vi "Results_file_Plotter.vi"() -> ()   [LabVIEW 2013]
uses:
  Anemometry/Anemometry Sub Vis/Data_plotting_vis/Plot_Slice.ctl
  Anemometry/Anemometry Sub Vis/Data_plotting_vis/Plotter_Mode.ctl
  Anemometry/Anemometry Sub Vis/Data_plotting_vis/Data_File_Type.ctl
  Anemometry/Anemometry Sub Vis/File/Setup_Filetype.ctl
  Anemometry/Anemometry Sub Vis/Controls/Global_mode.ctl
  Anemometry/Anemometry Sub Vis/Data_plotting_vis/Results_plotter_Global.vi
  Anemometry/Anemometry Sub Vis/Globals/Trav_pos_global.vi
  Instance           1 28Saved   Results_file_Plotter .vi
  Anemometry/Anemometry Sub Vis/Globals/Constants_global.vi
panel:
  out "Edit Raw DF?":bool
  in  "Tab Control":T1(tab)=enum."Save "
  in  "Template":path
  in  "Empty":bool
  in  "Result files to read":path[](array[path])
  in  "Add results file":bool
  in  "File Types to Read":T2
  in  "Dot Plot?":bool
  in  "Vector Plot?":bool
  in  "Ordinate Name":string
  out "2nd Add label":string
  out "First Add label":string
  in  "Additional X Values":dbl[](array[numeric]) format="%.2f"
  in  "Additional Y Values":dbl[](array[numeric]) format="%.2f"
  in  "Show Results Space Analysis":bool
  in  "Show Plot Space Analysis":bool
  in  "Multi Ordinate":i32[](listbox)
  in  "Multi Ordinate?":bool
  in  "Ordinate":u16(ring) items=["Project", "Case2", "Case", "Date", "File", "Ref Velocity (m/s) X=5m Y=-0.780m Z=1m", "Source Location X (mm)", "Source Location Y (mm)", "Source Location Z (mm)", "Source Internal Diameter (mm)", "Model Orientation", "Carrier Gas", "Trace Gas", "Q Source (l/min)", "Q Trace (l/min)", "Source Density Ratio", "Source", "X (mm)", "Y (mm)", "Z (mm)", "Location XY", "Location XZ", "Profiles", "U/U(ref)", "V/U(ref)", "W/U(ref)", "u^2/U_{ref}^2", "v^2/U_{ref}^2", "w^2/U_{ref}^2", "uv/U_{ref}^2", "-uw/U_{ref}^2", "CU(ref)/Q (m^{-2})", "c'U(ref)/Q (m^{-2})", "uc/Q (m^{-2})", "vc/Q (m^{-2})", "wc/Q (m^{-2})", "Measurement Time (min)", "U (m/s)", "U (m/s) St Error", "V (m/s)", "W (m/s)", "u^2 (m/s)^2", "v^2 (m/s)^2", "w^2 (m/s)^2", "uv (m/s)^2", "uw (m/s)^2", "C Trace (ppm)", "C Trace (ppm) St Error", "c^2 (ppm)^2", "uc (ppm m/s)", "vc (ppm m/s)", "wc (ppm m/s)", "Raw Data Filename", "EnFlo_Tunnel Inlet_Temp St Deviation", "Instrumentation", "Number of FFID Samples per Block", "Total Number of FFID Spikes Removed", "LDA (U) Timescale Estimate Integrated to 25%", "Number Of Measurement Blocks", "LDA Sampling Rate (Hz)", "Number of LDA Samples per Block", "Multi Run Start Time", "Bkgnd FF (C)", "Bkgnd Variance FF (C)", "Seconds since 1st Jan", "Drift%", "CU/Q Err", "EnFlo Lab labstrat1 Delta T", "GMU Carrier 2 Gas", "Emission Velocity m/s", "Emission Ratio", "FF (C) Standard Error in Variance", "GMU Source Type", "Aero_Tunnel Speed Meas Velocity", "Multi Run Row Number", "LDA (W) Standard Error in Mean", "LDA (U) Standard Error in Variance", "EnFlo_Tunnel FFID Temp", "FF (C) Calibration Filename", "Source2 Enable", "GMU Source Dem Q", "Multi Run Command Filename", "Thermistor Temp", "University Outside Temp", "Spires", "Run", "EnFlo_Tunnel Usonic_Ref_2 Velocity", "Roughness", "Dem_Uref", "Comments", "X Tunnel (mm)", "EnFlo_Tunnel Trav Origin X Offset", "Run_", "EnFlo_Tunnel Metadata Source Number", "EnFlo_Tunnel Metadata Model Trees"]
  in  "Intensity Plot?":bool
  in  "Absisca":u16(ring) items=["Project", "Case2", "Case", "Date", "File", "Ref Velocity (m/s) X=5m Y=-0.780m Z=1m", "Source Location X (mm)", "Source Location Y (mm)", "Source Location Z (mm)", "Source Internal Diameter (mm)", "Model Orientation", "Carrier Gas", "Trace Gas", "Q Source (l/min)", "Q Trace (l/min)", "Source Density Ratio", "Source", "X (mm)", "Y (mm)", "Z (mm)", "Location XY", "Location XZ", "Profiles", "U/U(ref)", "V/U(ref)", "W/U(ref)", "u^2/U_{ref}^2", "v^2/U_{ref}^2", "w^2/U_{ref}^2", "uv/U_{ref}^2", "-uw/U_{ref}^2", "CU(ref)/Q (m^{-2})", "c'U(ref)/Q (m^{-2})", "uc/Q (m^{-2})", "vc/Q (m^{-2})", "wc/Q (m^{-2})", "Measurement Time (min)", "U (m/s)", "U (m/s) St Error", "V (m/s)", "W (m/s)", "u^2 (m/s)^2", "v^2 (m/s)^2", "w^2 (m/s)^2", "uv (m/s)^2", "uw (m/s)^2", "C Trace (ppm)", "C Trace (ppm) St Error", "c^2 (ppm)^2", "uc (ppm m/s)", "vc (ppm m/s)", "wc (ppm m/s)", "Raw Data Filename", "EnFlo_Tunnel Inlet_Temp St Deviation", "Instrumentation", "Number of FFID Samples per Block", "Total Number of FFID Spikes Removed", "LDA (U) Timescale Estimate Integrated to 25%", "Number Of Measurement Blocks", "LDA Sampling Rate (Hz)", "Number of LDA Samples per Block", "Multi Run Start Time", "Bkgnd FF (C)", "Bkgnd Variance FF (C)", "Seconds since 1st Jan", "Drift%", "CU/Q Err", "EnFlo Lab labstrat1 Delta T", "GMU Carrier 2 Gas", "Emission Velocity m/s", "Emission Ratio", "FF (C) Standard Error in Variance", "GMU Source Type", "Aero_Tunnel Speed Meas Velocity", "Multi Run Row Number", "LDA (W) Standard Error in Mean", "LDA (U) Standard Error in Variance", "EnFlo_Tunnel FFID Temp", "FF (C) Calibration Filename", "Source2 Enable", "GMU Source Dem Q", "Multi Run Command Filename", "Thermistor Temp", "University Outside Temp", "Spires", "Run", "EnFlo_Tunnel Usonic_Ref_2 Velocity", "Roughness", "Dem_Uref", "Comments", "X Tunnel (mm)", "EnFlo_Tunnel Trav Origin X Offset", "Run_", "EnFlo_Tunnel Metadata Source Number", "EnFlo_Tunnel Metadata Model Trees"]
  in  "Job Directory":path
  in  "Save Averaged rows":bool
  in  "Save Surface Fit":bool
  in  "Output Filename":path
  in  "Save Data in Rows":bool
  in  "Save Plot data":bool
  in  "Header":string
  in  "Process Point":bool
  in  "Kill Point":bool
  out "Table":string[][](table)
  in  "Post Process Plotted Data":bool
  in  "...using routine":string
  in  "Calculate new metadata":bool
  in  "Add /Edit metadata":bool
  in  "Delete Plotted data from file":bool
  in  "Save Setup":bool
  in  "Load Setup":bool
  in  "stop":bool
  out "Current":string="Graph Scales"
  in  "Single Series":i32[](listbox)=[0]
  in  "Edit Template File":bool
  in  "color and symbol":bool
  out "nRows":i32
  in  "Filter Bins 2":i32[](listbox)=[0]
  in  "Filter 6":u16(ring)
  in  "Filter 5":u16(ring)
  in  "Filter 4":u16(ring)
  in  "Filter 3":u16(ring) items=["Show All (55)", "Lateral Profile (25)", "Vertical Profile (30)", "NOT Lateral Profile (30)", "NOT Vertical Profile (25)"]
  in  "Filter Array":u16[](array[ring])=[0, 0, 0, 0, 0, 0] items=["Don't Filter", "Project", "Case2", "Case", "Date", "File", "Ref Velocity (m/s) X=5m Y=-0.780m Z=1m", "Source Location X (mm)", "Source Location Y (mm)", "Source Location Z (mm)", "Source Internal Diameter (mm)", "Model Orientation", "Carrier Gas", "Trace Gas", "Q Source (l/min)", "Q Trace (l/min)", "Source Density Ratio", "Source", "X (mm)", "Y (mm)", "Z (mm)", "Location XY", "Location XZ", "Profiles", "U/U(ref)", "V/U(ref)", "W/U(ref)", "u^2/U_{ref}^2", "v^2/U_{ref}^2", "w^2/U_{ref}^2", "uv/U_{ref}^2", "-uw/U_{ref}^2", "CU(ref)/Q (m^{-2})", "c'U(ref)/Q (m^{-2})", "uc/Q (m^{-2})", "vc/Q (m^{-2})", "wc/Q (m^{-2})", "Measurement Time (min)", "U (m/s)", "U (m/s) St Error", "V (m/s)", "W (m/s)", "u^2 (m/s)^2", "v^2 (m/s)^2", "w^2 (m/s)^2", "uv (m/s)^2", "uw (m/s)^2", "C Trace (ppm)", "C Trace (ppm) St Error", "c^2 (ppm)^2", "uc (ppm m/s)", "vc (ppm m/s)", "wc (ppm m/s)", "Raw Data Filename", "EnFlo_Tunnel Inlet_Temp St Deviation", "Instrumentation", "Number of FFID Samples per Block", "Total Number of FFID Spikes Removed", "LDA (U) Timescale Estimate Integrated to 25%", "Number Of Measurement Blocks", "LDA Sampling Rate (Hz)", "Number of LDA Samples per Block", "Multi Run Start Time", "Bkgnd FF (C)", "Bkgnd Variance FF (C)", "Seconds since 1st Jan", "Drift%", "CU/Q Err", "EnFlo Lab labstrat1 Delta T", "GMU Carrier 2 Gas", "Emission Velocity m/s", "Emission Ratio", "FF (C) Standard Error in Variance", "GMU Source Type", "Aero_Tunnel Speed Meas Velocity", "Multi Run Row Number", "LDA (W) Standard Error in Mean", "LDA (U) Standard Error in Variance", "EnFlo_Tunnel FFID Temp", "FF (C) Calibration Filename", "Source2 Enable", "GMU Source Dem Q", "Multi Run Command Filename", "Thermistor Temp", "University Outside Temp", "Spires", "Run", "EnFlo_Tunnel Usonic_Ref_2 Velocity", "Roughness", "Dem_Uref", "Comments", "X Tunnel (mm)", "EnFlo_Tunnel Trav Origin X Offset", "Run_", "EnFlo_Tunnel Metadata Source Number", "EnFlo_Tunnel Metadata Model Trees"]
  in  "Filter Bins 1":i32[](listbox)=[0]
  in  "Create picture Vi Name":string caption="Picture VI:"
  in  "Save Plot as jpg":bool
  in  "Reload Files":bool
  out "Selected Row":i32
  out "Selected Row?":bool
  out "Warning!":string
  out "XY Plot":cluster{dbl[], dbl[]}[](graph)
  out "Edit Raw Data Header Info":bool
  out "Raw DF in Orig Pos?":bool
  out "Intensity Graph":dbl[][](graph)
  in  "Bkgnd Value":dbl
  in  "Update":bool
  in  "Plot Resolution":bool
  in  "Point Size":i32(slide)=1 scale=0.0..10.0
  in  "No of Contours":i32=20
  in  "Slice mode":T3
  in  "Z Ch Name":u16(ring) items=["Project", "Case2", "Case", "Date", "File", "Ref Velocity (m/s) X=5m Y=-0.780m Z=1m", "Source Location X (mm)", "Source Location Y (mm)", "Source Location Z (mm)", "Source Internal Diameter (mm)", "Model Orientation", "Carrier Gas", "Trace Gas", "Q Source (l/min)", "Q Trace (l/min)", "Source Density Ratio", "Source", "X (mm)", "Y (mm)", "Z (mm)", "Location XY", "Location XZ", "Profiles", "U/U(ref)", "V/U(ref)", "W/U(ref)", "u^2/U_{ref}^2", "v^2/U_{ref}^2", "w^2/U_{ref}^2", "uv/U_{ref}^2", "-uw/U_{ref}^2", "CU(ref)/Q (m^{-2})", "c'U(ref)/Q (m^{-2})", "uc/Q (m^{-2})", "vc/Q (m^{-2})", "wc/Q (m^{-2})", "Measurement Time (min)", "U (m/s)", "U (m/s) St Error", "V (m/s)", "W (m/s)", "u^2 (m/s)^2", "v^2 (m/s)^2", "w^2 (m/s)^2", "uv (m/s)^2", "uw (m/s)^2", "C Trace (ppm)", "C Trace (ppm) St Error", "c^2 (ppm)^2", "uc (ppm m/s)", "vc (ppm m/s)", "wc (ppm m/s)", "Raw Data Filename", "EnFlo_Tunnel Inlet_Temp St Deviation", "Instrumentation", "Number of FFID Samples per Block", "Total Number of FFID Spikes Removed", "LDA (U) Timescale Estimate Integrated to 25%", "Number Of Measurement Blocks", "LDA Sampling Rate (Hz)", "Number of LDA Samples per Block", "Multi Run Start Time", "Bkgnd FF (C)", "Bkgnd Variance FF (C)", "Seconds since 1st Jan", "Drift%", "CU/Q Err", "EnFlo Lab labstrat1 Delta T", "GMU Carrier 2 Gas", "Emission Velocity m/s", "Emission Ratio", "FF (C) Standard Error in Variance", "GMU Source Type", "Aero_Tunnel Speed Meas Velocity", "Multi Run Row Number", "LDA (W) Standard Error in Mean", "LDA (U) Standard Error in Variance", "EnFlo_Tunnel FFID Temp", "FF (C) Calibration Filename", "Source2 Enable", "GMU Source Dem Q", "Multi Run Command Filename", "Thermistor Temp", "University Outside Temp", "Spires", "Run", "EnFlo_Tunnel Usonic_Ref_2 Velocity", "Roughness", "Dem_Uref", "Comments", "X Tunnel (mm)", "EnFlo_Tunnel Trav Origin X Offset", "Run_", "EnFlo_Tunnel Metadata Source Number", "EnFlo_Tunnel Metadata Model Trees"]
  in  "Y Ch Name":u16(ring) items=["Project", "Case2", "Case", "Date", "File", "Ref Velocity (m/s) X=5m Y=-0.780m Z=1m", "Source Location X (mm)", "Source Location Y (mm)", "Source Location Z (mm)", "Source Internal Diameter (mm)", "Model Orientation", "Carrier Gas", "Trace Gas", "Q Source (l/min)", "Q Trace (l/min)", "Source Density Ratio", "Source", "X (mm)", "Y (mm)", "Z (mm)", "Location XY", "Location XZ", "Profiles", "U/U(ref)", "V/U(ref)", "W/U(ref)", "u^2/U_{ref}^2", "v^2/U_{ref}^2", "w^2/U_{ref}^2", "uv/U_{ref}^2", "-uw/U_{ref}^2", "CU(ref)/Q (m^{-2})", "c'U(ref)/Q (m^{-2})", "uc/Q (m^{-2})", "vc/Q (m^{-2})", "wc/Q (m^{-2})", "Measurement Time (min)", "U (m/s)", "U (m/s) St Error", "V (m/s)", "W (m/s)", "u^2 (m/s)^2", "v^2 (m/s)^2", "w^2 (m/s)^2", "uv (m/s)^2", "uw (m/s)^2", "C Trace (ppm)", "C Trace (ppm) St Error", "c^2 (ppm)^2", "uc (ppm m/s)", "vc (ppm m/s)", "wc (ppm m/s)", "Raw Data Filename", "EnFlo_Tunnel Inlet_Temp St Deviation", "Instrumentation", "Number of FFID Samples per Block", "Total Number of FFID Spikes Removed", "LDA (U) Timescale Estimate Integrated to 25%", "Number Of Measurement Blocks", "LDA Sampling Rate (Hz)", "Number of LDA Samples per Block", "Multi Run Start Time", "Bkgnd FF (C)", "Bkgnd Variance FF (C)", "Seconds since 1st Jan", "Drift%", "CU/Q Err", "EnFlo Lab labstrat1 Delta T", "GMU Carrier 2 Gas", "Emission Velocity m/s", "Emission Ratio", "FF (C) Standard Error in Variance", "GMU Source Type", "Aero_Tunnel Speed Meas Velocity", "Multi Run Row Number", "LDA (W) Standard Error in Mean", "LDA (U) Standard Error in Variance", "EnFlo_Tunnel FFID Temp", "FF (C) Calibration Filename", "Source2 Enable", "GMU Source Dem Q", "Multi Run Command Filename", "Thermistor Temp", "University Outside Temp", "Spires", "Run", "EnFlo_Tunnel Usonic_Ref_2 Velocity", "Roughness", "Dem_Uref", "Comments", "X Tunnel (mm)", "EnFlo_Tunnel Trav Origin X Offset", "Run_", "EnFlo_Tunnel Metadata Source Number", "EnFlo_Tunnel Metadata Model Trees"]
  in  "X Ch Name":u16(ring) items=["Project", "Case2", "Case", "Date", "File", "Ref Velocity (m/s) X=5m Y=-0.780m Z=1m", "Source Location X (mm)", "Source Location Y (mm)", "Source Location Z (mm)", "Source Internal Diameter (mm)", "Model Orientation", "Carrier Gas", "Trace Gas", "Q Source (l/min)", "Q Trace (l/min)", "Source Density Ratio", "Source", "X (mm)", "Y (mm)", "Z (mm)", "Location XY", "Location XZ", "Profiles", "U/U(ref)", "V/U(ref)", "W/U(ref)", "u^2/U_{ref}^2", "v^2/U_{ref}^2", "w^2/U_{ref}^2", "uv/U_{ref}^2", "-uw/U_{ref}^2", "CU(ref)/Q (m^{-2})", "c'U(ref)/Q (m^{-2})", "uc/Q (m^{-2})", "vc/Q (m^{-2})", "wc/Q (m^{-2})", "Measurement Time (min)", "U (m/s)", "U (m/s) St Error", "V (m/s)", "W (m/s)", "u^2 (m/s)^2", "v^2 (m/s)^2", "w^2 (m/s)^2", "uv (m/s)^2", "uw (m/s)^2", "C Trace (ppm)", "C Trace (ppm) St Error", "c^2 (ppm)^2", "uc (ppm m/s)", "vc (ppm m/s)", "wc (ppm m/s)", "Raw Data Filename", "EnFlo_Tunnel Inlet_Temp St Deviation", "Instrumentation", "Number of FFID Samples per Block", "Total Number of FFID Spikes Removed", "LDA (U) Timescale Estimate Integrated to 25%", "Number Of Measurement Blocks", "LDA Sampling Rate (Hz)", "Number of LDA Samples per Block", "Multi Run Start Time", "Bkgnd FF (C)", "Bkgnd Variance FF (C)", "Seconds since 1st Jan", "Drift%", "CU/Q Err", "EnFlo Lab labstrat1 Delta T", "GMU Carrier 2 Gas", "Emission Velocity m/s", "Emission Ratio", "FF (C) Standard Error in Variance", "GMU Source Type", "Aero_Tunnel Speed Meas Velocity", "Multi Run Row Number", "LDA (W) Standard Error in Mean", "LDA (U) Standard Error in Variance", "EnFlo_Tunnel FFID Temp", "FF (C) Calibration Filename", "Source2 Enable", "GMU Source Dem Q", "Multi Run Command Filename", "Thermistor Temp", "University Outside Temp", "Spires", "Run", "EnFlo_Tunnel Usonic_Ref_2 Velocity", "Roughness", "Dem_Uref", "Comments", "X Tunnel (mm)", "EnFlo_Tunnel Trav Origin X Offset", "Run_", "EnFlo_Tunnel Metadata Source Number", "EnFlo_Tunnel Metadata Model Trees"]
  in  "Resolution":dbl=1.0 min=0.0 format="%.4f"
  out "Surface Area":dbl format="%^_6g"
  out "Surface Integral":dbl format="%^_6g"
  out "Surface Average":dbl format="%^#.6g"
  out "Uadvec":dbl
  in  "Full_Res_Results_Folder":path
  out "Last used Template":path
  out "Cursor index":i32
  out "Choosen Path":path
  in  "VI Refnum Calculation":refnum<vi>
  out "Filetype":string[](array[string])
  out "Mode":T4
  out "Plotted rows only?":bool
  in  "type specifier VI Refnum (for type only) 2":refnum<vi>
  in  "type specifier VI Refnum (for type only)":refnum<vi>
  out "Accept Array":bool[][](array[boolean])
  out "Previous slice mode":T3
  out "Slice mode Change?":bool
  out "Non-Blank Rows":bool[](array[boolean])
  out "File Index":i32
  out "Tolerances":dbl[](array[numeric]) format="%.2f"
  in  "Results files choosen":path[](array[path])
  in  "Transpose":bool
  out "Plotted Series":bool[][](array[boolean])
  in  "Results file":path
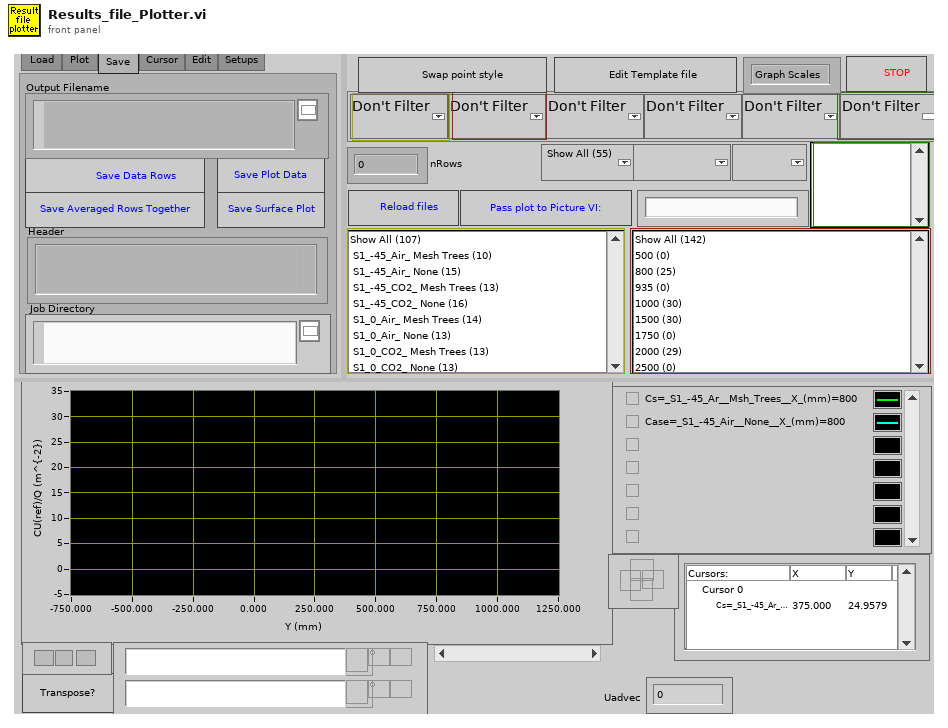
[diagram p1: front panel]
types:
  T1 = enum32{"Load ", "Plot ", "Save ", "Cursor", "Edit", "Setups"}
  T2 = typedef "Data_File_Type.ctl" = enum16{"Read All File Types", "Results Files Only", "Raw Data Files Only", "Calibration Files Only", "Gas Desk Files Only", "Old Results Files Only", "Tabulated Data Files Only"}
  T3 = typedef "Plot_Slice.ctl" = enum16{"XY Slice (Plan)", "YX Slice (Plan)", "YZ Slice (Cross)", "ZY Slice (Cross)", "XZ Slice (Side)", "ZX Slice (Side)"}
  T4 = typedef "Plotter_Mode.ctl" = enum16{"Save file", "Delete unwanted rows", "Edit Values with constants", "Edit values per row", "Edit Raw Data file header", "Post Process Plotted Rows"}
  T5 = typedef "Setup_Filetype.ctl" = enum16{"Measurement Setups", "Calibration Setups", "General", "Results File Plotter Setups", "Speed Calib Tweaks"}
  T6 = enum16{"Zero or one", "One", "Zero or more", "One or more"}
  T7 = typedef "Global_mode.ctl" = enum16{"Read Global", "Load Global From File", "Write Global to File"}
  T8 = enum16{"Edit Existing Template File", "Create New Template File"}
  T9 = enum16{"Show only data summary", "Show data summary", "No data summary"}
  T10 = typedef "All_Setup.ctl" = cluster{"Result files to read":path[], "Template":path, "Transpose":bool, "Additional X Values":dbl[], "Additional Y Values":dbl[], "Ordinate":u16, "Absisca":u16, "Filter Array":u16[], "color and symbol":bool, "Output Filename":path, "Jpg Vi Name":string, "Intensity Plot?":bool, "Multi Ordinate?":bool, "Filter Bins 1":i32[], "Filter Bins 2":i32[], "Multi Ordinate":i32[]}
  T11 = enum16{"Left Button", "Center Button", "Right Button", "Window Close"}
  T12 = enum32{"existing file", "new file", "new or existing file", "existing dir", "new dir", "new or existing dir", "existing file (use LLBs)", "new file (use LLBs)", "new or existing file (use LLBs)", "new or existing file or directory (use LLBs)"}
  T13 = cluster{"Plot Color":u32, "Plot Interpolation":u8, "Point Style":u8, "Line Style":u8, "Fill/Pt. Color":u32, "Line Width":u8, "Bar Plot Style":u8, "Fill To":i16}[]
  T14 = cluster{"X Max":dbl, "Y Max ":dbl, "X Scale":cluster{"Xo":dbl, "delta X":dbl}, "Y Scale":cluster{"Xo":dbl, "delta X":dbl}, "X Values":dbl[], "Y Values":dbl[], "Z Max":dbl, "Z Min":dbl}
  T15 = typedef "Group_Binning.ctl" = cluster{"Index":i32, "Tolerance":dbl, "Precision":string}
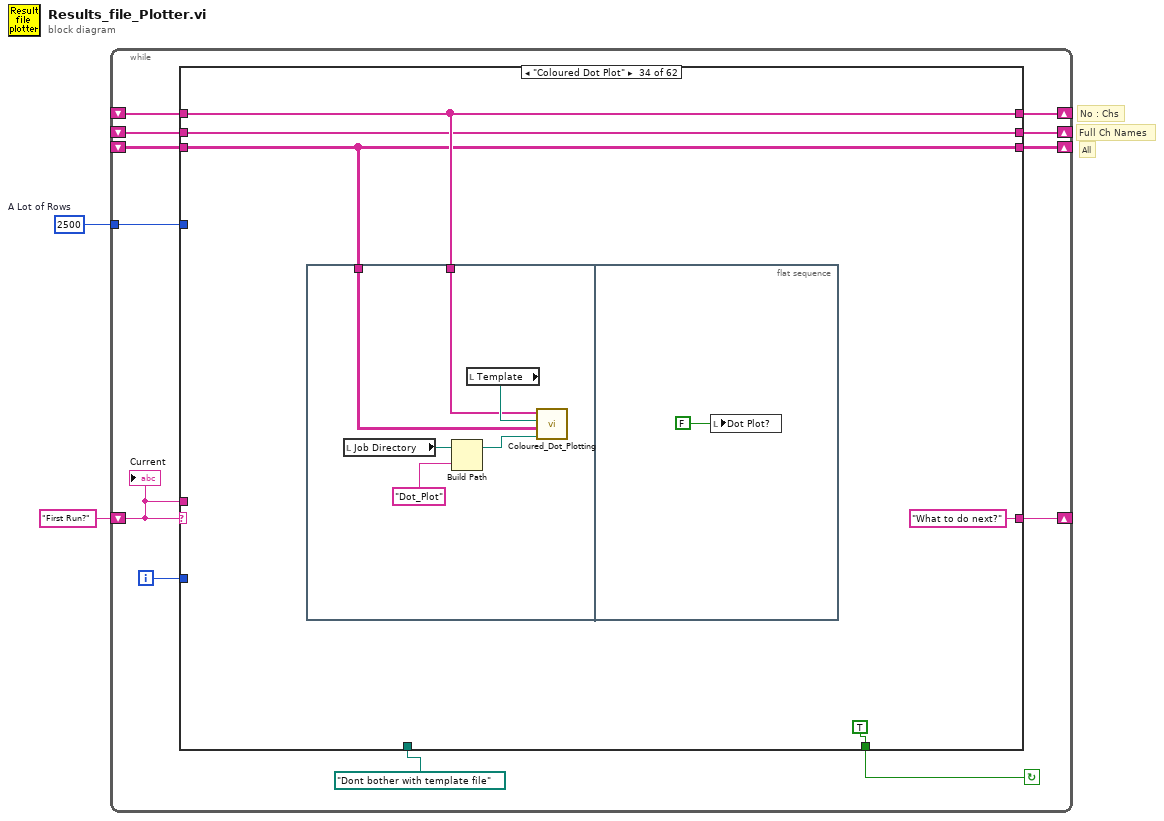
[diagram p0: block diagram]
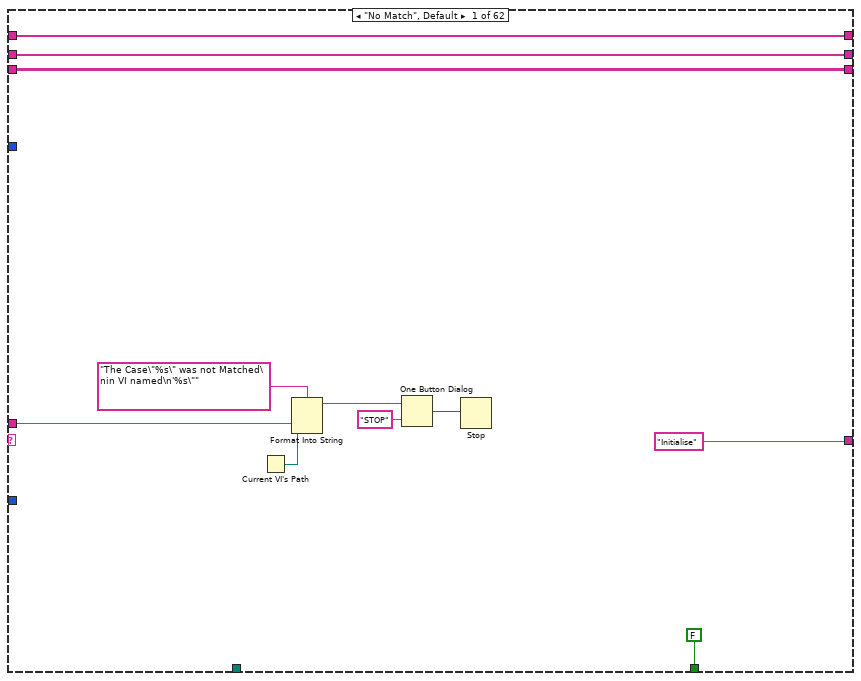
[diagram p2: hidden frame]
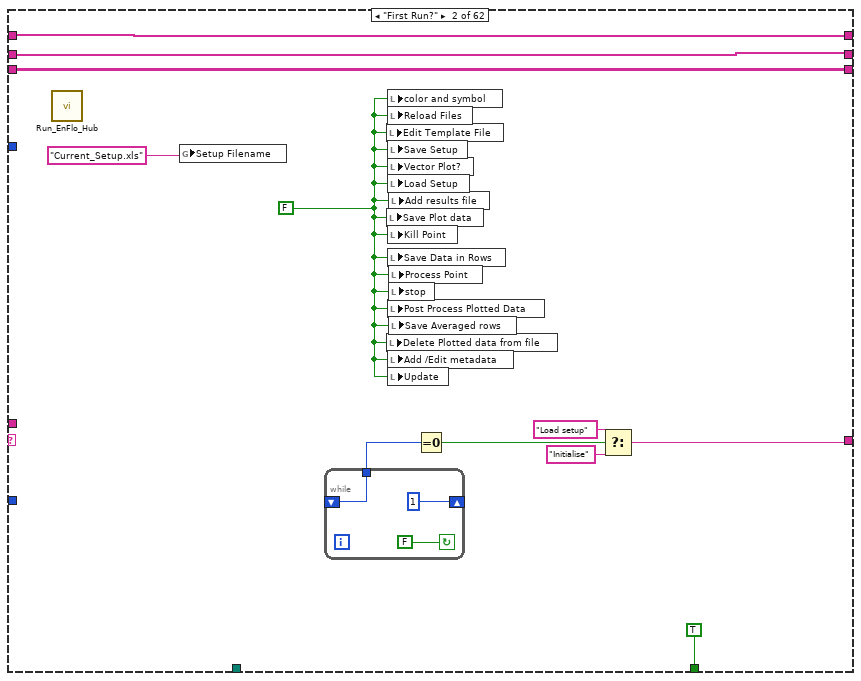
[diagram p3: hidden frame]
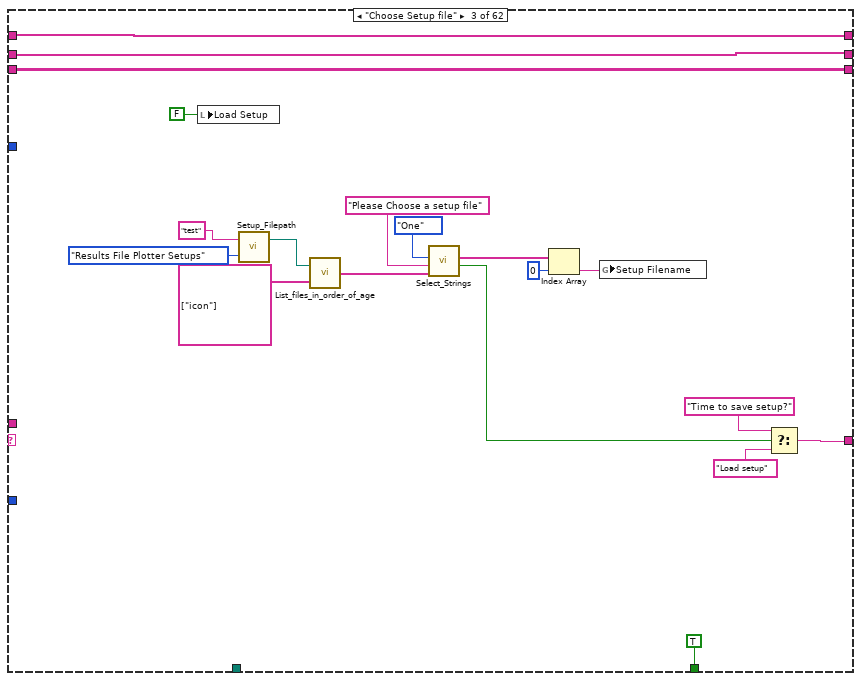
[diagram p4: hidden frame]
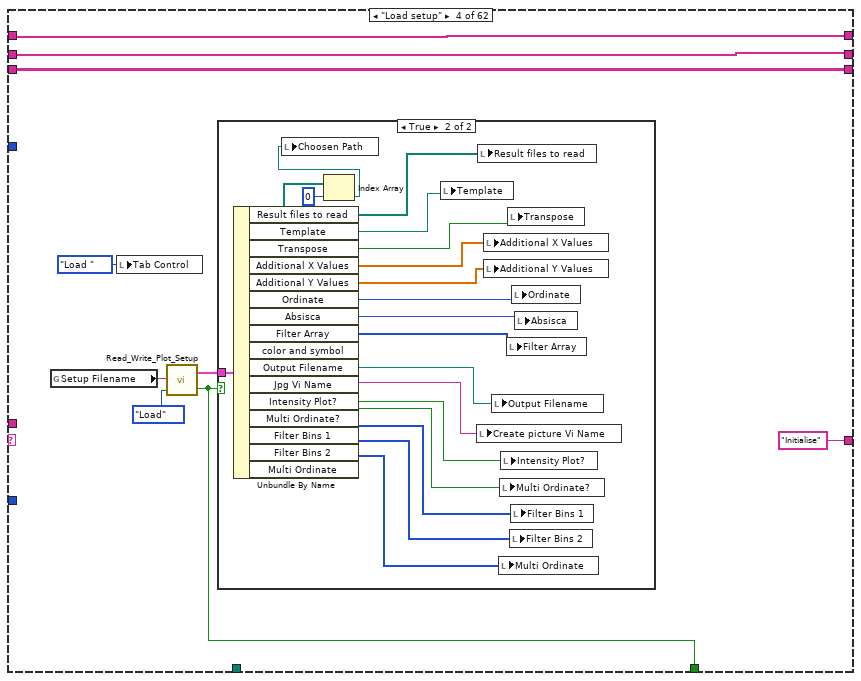
[diagram p5: hidden frame]
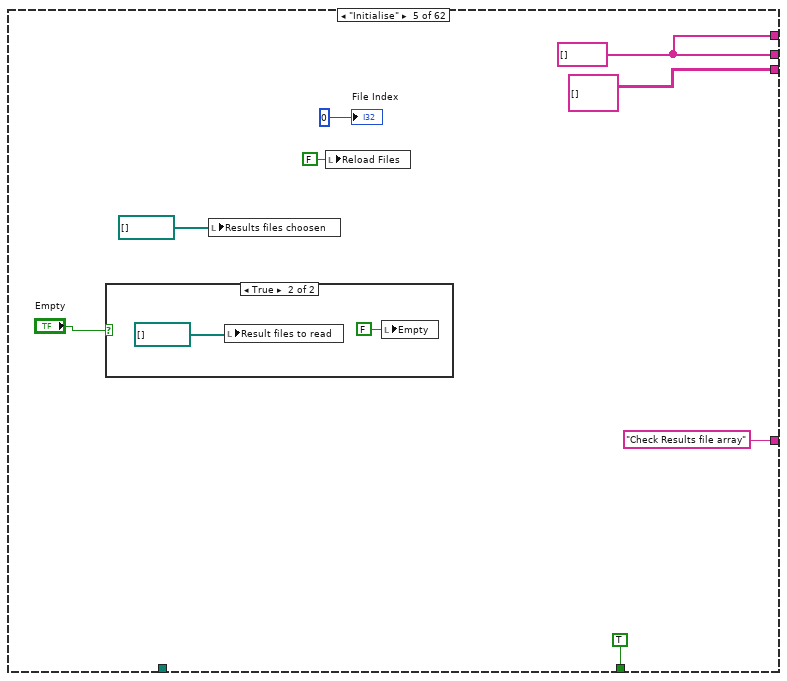
[diagram p7: hidden frame]
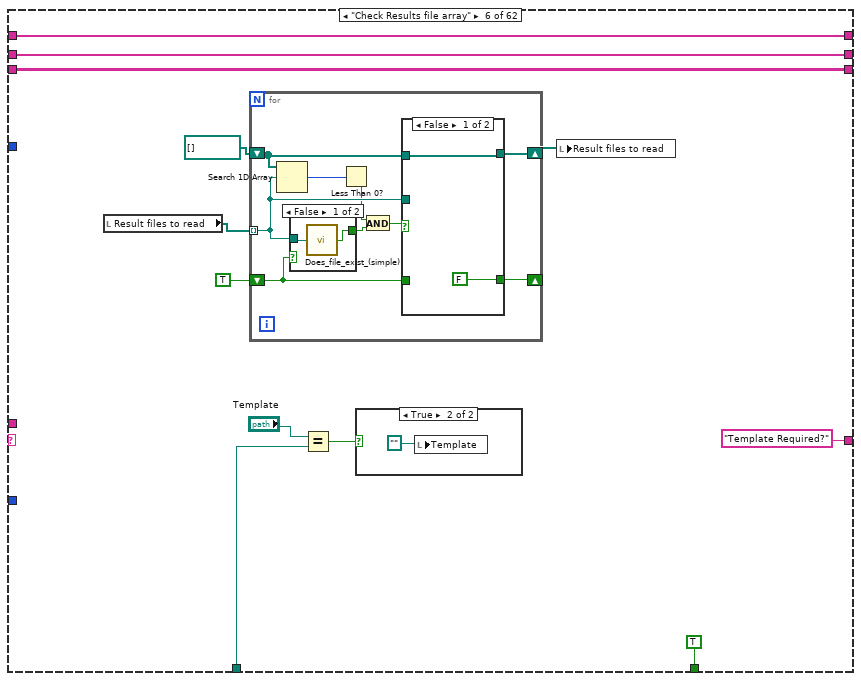
[diagram p9: hidden frame]
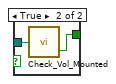
[diagram p11: hidden frame]
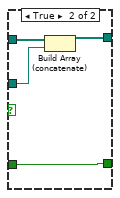
[diagram p12: hidden frame]
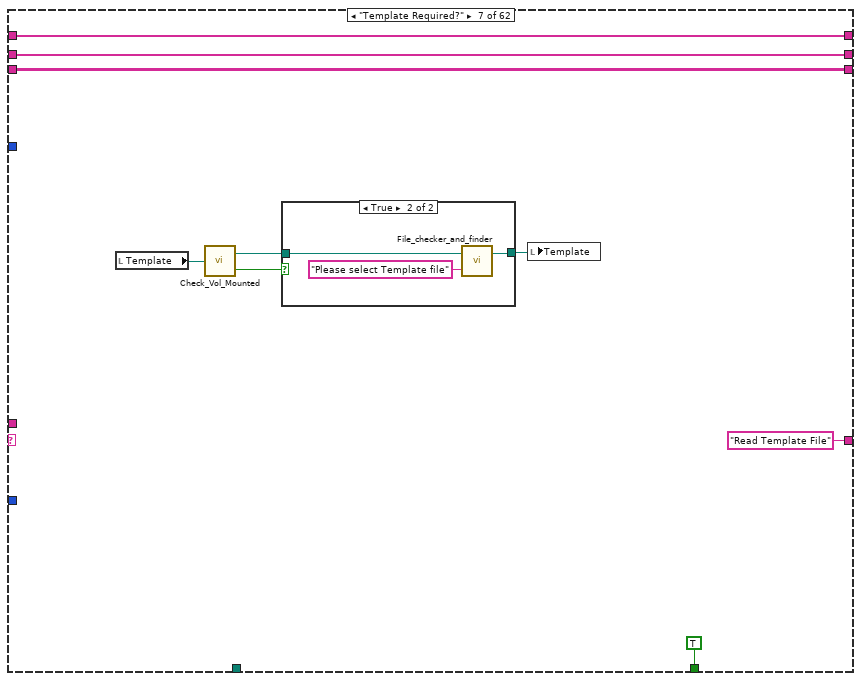
[diagram p13: hidden frame]
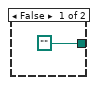
[diagram p14: hidden frame]
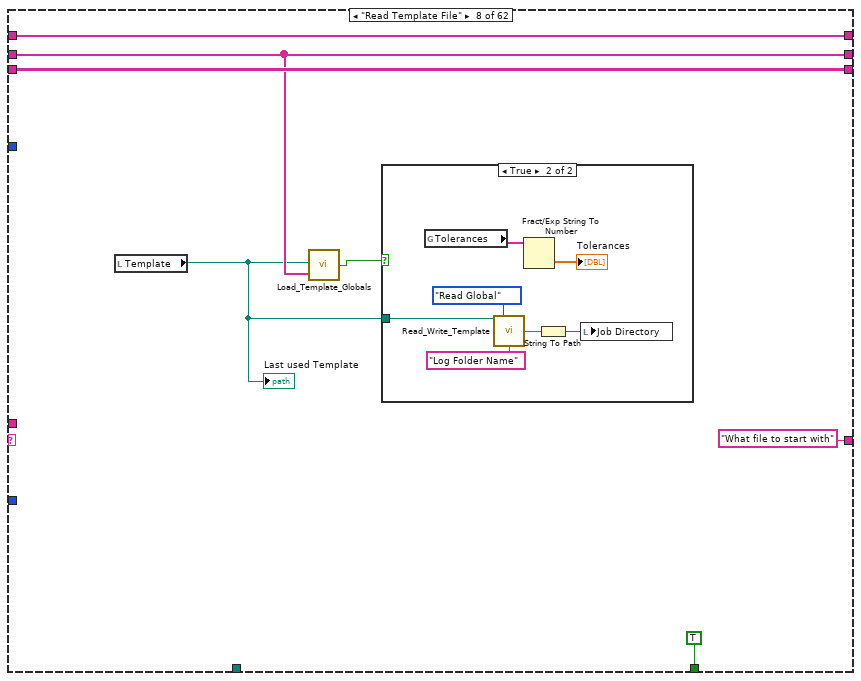
[diagram p15: hidden frame]
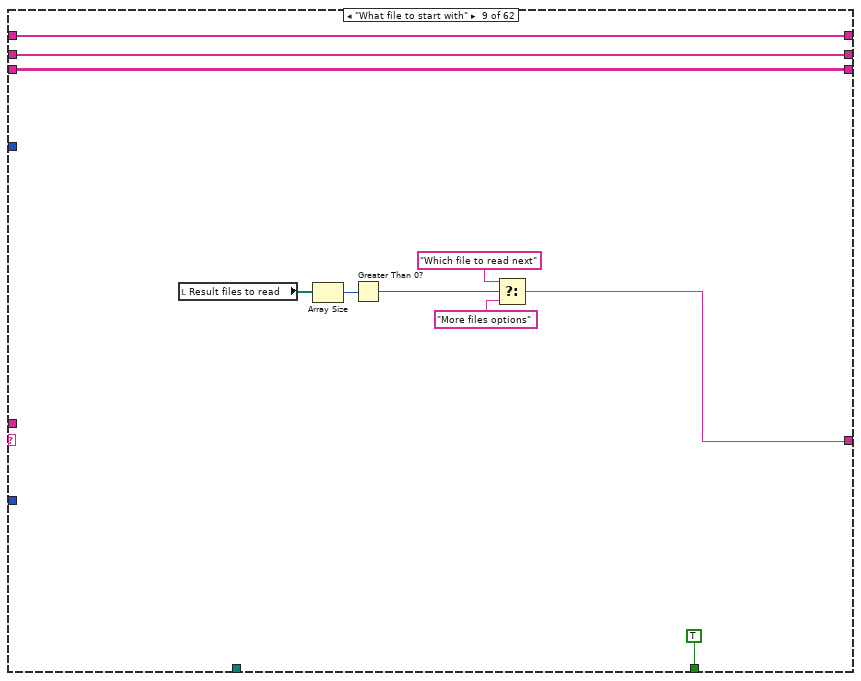
[diagram p17: hidden frame]
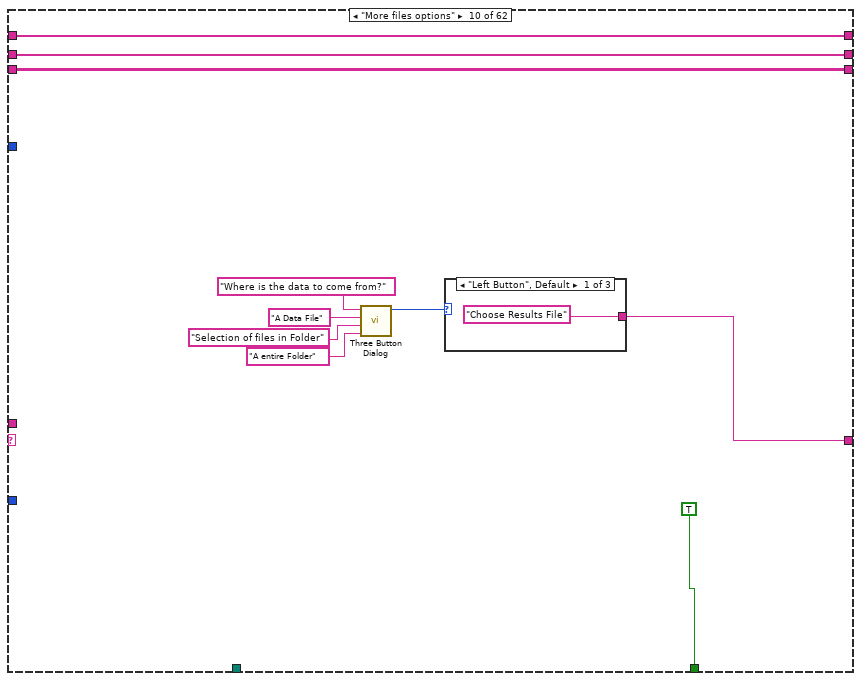
[diagram p18: hidden frame]
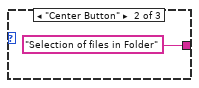
[diagram p19: hidden frame]
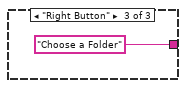
[diagram p20: hidden frame]
diagram:
  w1 = 2500  # A Lot of Rows
  # "No : Chs"
  # "Full Ch Names"
  # "All"
  n1 = while {
    shift-left: _ -> [w7]
    shift-right: [w8] -> _
    shift-left: "First Run?" -> [w11]
    shift-right: [w4] -> _
    shift-left: _ -> [w9]
    shift-right: [w14] -> _
    shift-left: _ -> [w12]
    shift-right: [w5] -> _
    tunnel: w1 -> [w3]
    i -> [w6]
    stop <- w13 continue-if-true
    n2 = case shown="\"Coloured Dot Plot\"" w11 {
      tunnel: w9 -> [w25 w35 w57 w65 _ w106 w134 w143 w164 w174 w186 w200 w231 w258 w281 w403 w425 w451 w476 w502 w556 w570 w607 w917 w988 w1043 w1068 w1087 w1173 w1224 w1254 w1554 w1570 w1582 w1609 w1639 w1705 w1738 w1813 w1836 w1851 w1915 w1967 w1993 w2202 w2214 w2240 w2366 w2510 w2544 w2559 w2584 w2611 w2654 w2672 w2715 w2818 w2852 w3216 w3231 w3267 w3275]
      tunnel: [w25 w35 w57 w65 w91 w106 w134 w143 w164 w174 w186 w200 w231 w258 w279 w403 w425 w451 w476 w502 w556 w570 w607 w917 w988 w1043 w1068 w1087 w1173 w1224 w1252 w1554 w1570 w1582 w1609 w1639 w1705 w1738 w1813 w1836 w1851 w1915 w1967 w1991 w2202 w2214 w2238 w2359 w2510 w2544 w2559 w2584 w2611 w2654 w2672 w2715 w2818 w2852 w3216 w3231 w3267 w3275] -> w14
      tunnel: ["Initialise" w28 w52 "Initialise" ("t") "Check Results file array" ("t") "Template Required?" "Read Template File" "What file to start with" w155 w170 "Which file to read next" "Which file to read next" "Which file to read next" w254 w276 w394 "What is present?" "Ordinate Selector Type" w473 "Which rows are Non-Blank?" w549 "Create Selectors" w596 "Re Plot Data?" w983 "Prepare Filter2 strings" "Plot Data" w1084 "Add Axis names" "Analyse Plot Space" w1255 "What to do next?" "What to do next?" ("t") "What to do next?" ("t") w1591 w1632 w1683 w1736 w1807 w1832 w1850 w1914 "Initialise" w1994 w2193 "Create Selectors" w2241 w2367 w2508 w2542 w2549 w2568 "Save XY plot as jpg" "Create Selectors" w2669 w2718 w2802 w2857 "Save Setup" ("t") "Initialise" ("t") w3236 "Time to save setup?"] -> w4
      tunnel: [FALSE TRUE TRUE w61 TRUE TRUE TRUE TRUE TRUE TRUE TRUE TRUE TRUE w249 w283 TRUE TRUE TRUE TRUE TRUE TRUE TRUE TRUE TRUE TRUE TRUE TRUE w1085 TRUE TRUE w1256 TRUE TRUE ("OK?") TRUE ("OK?") TRUE TRUE ("OK?") TRUE ("OK?") w1734 TRUE TRUE w1849 w1913 TRUE w1995 TRUE ("OK?") TRUE ("OK?") w2242 w2368 TRUE TRUE TRUE TRUE TRUE TRUE TRUE TRUE TRUE TRUE TRUE TRUE w3245 TRUE ("OK?")] -> w13
      tunnel: w12 -> [w24 w34 w56 w64 _ w105 w133 w145 w163 w173 w185 w199 w230 w257 w282 w399 w424 w452 w477 w503 w555 w568 w602 w919 w977 w1045 w1070 w1086 w1175 w1226 w1253 w1553 w1569 w1581 w1608 w1650 w1704 w1737 w1812 w1835 w1848 w1912 w1966 w1992 w2201 w2211 w2239 w2365 w2511 w2543 w2558 w2588 w2614 w2653 w2671 w2714 w2817 w2851 w3215 w3230 w3266 w3274]
      tunnel: w11 -> [w16 _ _ _ _ _ _ _ _ _ _ _ _ _ _ _ _ _ _ _ _ _ _ _ _ _ _ _ _ _ _ _ _ _ _ _ _ _ _ _ _ _ _ _ _ _ _ _ _ _ _ _ _ _ _ _ _ _ _ _ _ _]
      tunnel: path "Dont bother with template file" ("Template File") -> [_ _ _ _ _ w99 _ _ _ _ _ _ _ _ _ _ _ _ _ _ _ _ _ _ _ _ _ _ _ _ _ _ _ _ _ _ _ _ _ _ _ _ _ _ _ _ _ _ _ _ _ _ _ _ _ _ _ _ w3213 w3225 _ _]
      tunnel: [w15 w33 w55 w66 w91 w104 w132 w144 w161 w171 w183 w197 w228 w256 w278 w387 w423 w453 w475 w501 w547 w569 w600 w916 w979 w1036 w1063 w1083 w1167 w1219 w1248 w1550 w1571 w1583 w1607 w1640 w1706 w1739 w1811 w1834 w1847 w1911 w1965 w1985 w2203 w2219 w2229 w2362 w2520 w2545 w2560 w2585 w2612 w2655 w2673 w2719 w2819 w2858 w3217 w3232 w3268 w3276] -> w8
      tunnel: w7 -> [w15 w33 w55 w66 _ w104 w132 w144 w161 w171 w183 w197 w228 w256 w277 w387 w423 w453 w475 w501 w547 w569 w600 w916 w979 w1036 w1063 w1083 w1167 w1219 w1247 w1550 w1571 w1583 w1607 w1640 w1706 w1739 w1811 w1834 w1847 w1911 w1965 w1984 w2203 w2219 w2233 w2361 w2520 w2545 w2560 w2585 w2612 w2655 w2673 w2719 w2819 w2858 w3217 w3232 w3268 w3276]
      tunnel: w6 -> [_ _ _ _ _ _ _ _ _ _ _ _ _ _ _ _ _ _ _ _ _ _ _ _ _ _ _ _ _ _ _ _ _ _ _ _ _ w1735 _ _ _ _ _ _ _ _ _ _ _ _ _ _ _ _ _ _ _ _ _ _ _ _]
      tunnel: [w24 w34 w56 w64 string[][] [] w105 w133 w145 w163 w173 w185 w199 w230 w257 w280 w399 w424 w452 w477 w503 w555 w568 w602 w919 w977 w1045 w1070 w1086 w1175 w1226 w1251 w1553 w1569 w1581 w1608 w1650 w1704 w1737 w1812 w1835 w1848 w1912 w1966 w1990 w2201 w2211 w2237 w2358 w2511 w2543 w2558 w2588 w2614 w2653 w2671 w2714 w2817 w2851 w3215 w3230 w3266 w3274] -> w5
      tunnel: w3 -> [_ _ _ _ _ _ _ _ _ _ _ _ _ _ _ _ _ _ _ _ _ _ _ _ _ _ _ _ _ _ _ _ _ _ _ _ _ _ _ w1830 _ w1910 _ _ _ _ _ _ _ _ _ _ _ _ w2668 w2712 _ w2849 _ _ _ _]
      frame "No Match", Default {
        n3 = Current VI's Path() -> (path=w17:path)
        n4 = Format Into String(format string="The Case\"%s\" was not Matched\nin VI named\n'%s\"" ("Format String"), w16, w17) -> (resulting string=w20:string)  [unwired: 2 in, 1 out]
        n5 = One Button Dialog(message=w20, button name ("OK")="STOP") -> (true=w18:bool)
        n6 = Stop(stop? (T)=w18) -> ()
      }
      frame "First Run?" {
        w26 = FALSE ("Save Plot data")
        n7 = call "Run_EnFlo_Hub.vi"() -> ()  [unwired: 8 out]
        n8 = global write "Results_plotter_Global.vi" "Setup Filename"("Current_Setup.xls" ("Setup filename")) -> ()
        n9 = while {
          shift-right: [1] -> _
          shift-left: _ -> [w38]
          tunnel: [w38] -> w30
          stop <- FALSE continue-if-true
        }
        n10 = local write "Edit Template File"(w26) -> ()
        n11 = local write "Save Plot data"(w26) -> ()
        n12 = local write "Delete Plotted data from file"(w26) -> ()
        n13 = local write "color and symbol"(w26) -> ()
        n14 = local write "Reload Files"(w26) -> ()
        n15 = local write "Save Setup"(w26) -> ()
        n16 = local write "Vector Plot?"(w26) -> ()
        n17 = local write "Load Setup"(w26) -> ()
        n18 = local write "Kill Point"(w26) -> ()
        n19 = local write "Save Data in Rows"(w26) -> ()
        n20 = local write "Post Process Plotted Data"(w26) -> ()
        n21 = local write "Add /Edit metadata"(w26) -> ()
        n22 = local write "Update"(w26) -> ()
        n23 = local write "Add results file"(w26) -> ()
        n24 = local write "Process Point"(w26) -> ()
        n25 = local write "stop"(w26) -> ()
        n26 = local write "Save Averaged rows"(w26) -> ()
        n27 = Equal To 0?(x=w30) -> (x = 0?=w29:bool)
        n28 = Select(t="Load setup", s=w29, f="Initialise") -> (s? t:f=w28:string)
      }
      frame "Choose Setup file" {
        n29 = local write "Load Setup"(FALSE ("Save Setup")) -> ()
        n30 = call "Setup_Filepath.vi"("Setup File Type"=Setup_Filetype."Results File Plotter Setups", "Filename in"="test") -> ("Directory"=w40:path)  [unwired: 1 out]
        n31 = call "List_files_in_order_of_age.vi"("Files to Hide"=string[] ["icon"], "Folder"=w40) -> ("file names"=w51:string[])
        n32 = call "Select_Strings.vi"("Available Ch names"=w51, "Message"="Please Choose a setup file", "Selector mode"=T6."One") -> ("Cancel"=w45:bool, "Selected Channel Names"=w48:string[])  [unwired: 1 in, 3 out]
        n33 = Index Array(array=w48, index=0) -> (element=w46:string)
        n34 = global write "Results_plotter_Global.vi" "Setup Filename"(w46) -> ()
        n35 = Select(t="Time to save setup?", s=w45, f="Load setup") -> (s? t:f=w52:string)
      }
      frame "Load setup" {
        n36 = global read "Results_plotter_Global.vi" "Setup Filename"() -> (w60:string)
        n37 = local write "Tab Control"(T1."Load " ("Tab Control")) -> ()
        n38 = call "Read_Write_Plot_Setup.vi"("Mode"=enum16{"Load", "Save"}."Load", "Setup filename"=w60) -> ("OK?"=w61:bool, "Cluster 2"=w62:T10)  [unwired: 1 in]
        n39 = case shown="True" w61 {
          tunnel: w62 -> [_ w85]
          frame False {
          }
          frame True {
            n40 = Unbundle By Name(w85) -> ("Result files to read"=w70:path[], "Template"=w68:path, "Transpose"=w75:bool, "Additional X Values"=w76:dbl[], "Additional Y Values"=w77:dbl[], "Ordinate"=w78:u16, "Absisca"=w79:u16, "Filter Array"=w80:u16[], "Output Filename"=w81:path, "Jpg Vi Name"=w82:string, "Intensity Plot?"=w83:bool, "Multi Ordinate?"=w84:bool, "Filter Bins 1"=w74:i32[], "Filter Bins 2"=w73:i32[], "Multi Ordinate"=w72:i32[])  [unwired: 1 out]
            n41 = Index Array(array=w70, index=0) -> (element=w69:path)
            n42 = local write "Choosen Path"(w69) -> ()
            n43 = local write "Template"(w68) -> ()
            n44 = local write "Create picture Vi Name"(w82) -> ()
            n45 = local write "Result files to read"(w70) -> ()
            n46 = local write "Additional X Values"(w76) -> ()
            n47 = local write "Additional Y Values"(w77) -> ()
            n48 = local write "Output Filename"(w81) -> ()
            n49 = local write "Multi Ordinate"(w72) -> ()
            n50 = local write "Multi Ordinate?"(w84) -> ()
            n51 = local write "Intensity Plot?"(w83) -> ()
            n52 = local write "Filter Array"(w80) -> ()
            n53 = local write "Transpose"(w75) -> ()
            n54 = local write "Filter Bins 2"(w73) -> ()
            n55 = local write "Filter Bins 1"(w74) -> ()
            n56 = local write "Ordinate"(w78) -> ()
            n57 = local write "Absisca"(w79) -> ()
          }
        }
      }
      frame "Initialise" {
        w91 = string[] [] ("Channel names")
        n58 = case shown="True" "Empty" {
          frame False {
          }
          frame True {
            n59 = local write "Result files to read"(path[] [] ("Result files to read")) -> ()
            n60 = local write "Empty"(FALSE ("Empty")) -> ()
          }
        }
        n61 = local write "Results files choosen"(path[] [] ("Results file choosen")) -> ()
        n62 = local write "Reload Files"(FALSE ("Reload Files")) -> ()
        "File Index" <- 0
      }
      frame "Check Results file array" {
        n63 = local read "Result files to read"() -> (w103:path[])
        n64 = for {
          shift-right: [w117] -> w101
          shift-left: path[] [] -> [w116]
          tunnel: w103 -> [w115] mode=indexing
          shift-right: [w110] -> _
          shift-left: TRUE -> [w109]
          n65 = Search 1D Array(1D array=w116, element=w115) -> (index of element=w114:i32)  [unwired: 1 out]
          n66 = case shown="False" w109 {
            tunnel: w115 -> [w119 w121]
            tunnel: [w118 w120] -> w112
            frame False {
              n67 = call "Does_file_exist_(simple).vi"("Pathname"=w119) -> ("exists?"=w118:bool)
            }
            frame True {
              n68 = call "Check_Vol_Mounted.vi"("Filename"=w121) -> ("exists?"=w120:bool)  [unwired: 1 out]
            }
          }
          n69 = Less Than 0?(x=w114) -> (x < 0?=w111:bool)
          n70 = And(x=w111, y=w112) -> (x .and. y?=w113:bool)
          n71 = case shown="False" w113 {
            tunnel: w116 -> [w123 w127]
            tunnel: w115 -> [_ w126]
            tunnel: [w123 w125] -> w117
            tunnel: [FALSE w124] -> w110
            tunnel: w109 -> [_ w124]
            frame False {
            }
            frame True {
              n72 = Build Array (concatenate)(w127, w126) -> (w125:path[])
            }
          }
        }
        n73 = Equal?(x="Template", y=w99) -> (x = y?=w98:bool)
        n74 = case shown="True" w98 {
          frame False {
          }
          frame True {
            n75 = local write "Template"(path "") -> ()
          }
        }
        n76 = local write "Result files to read"(w101) -> ()
      }
      frame "Template Required?" {
        n77 = local read "Template"() -> (w131:path)
        n78 = call "Check_Vol_Mounted.vi"("Filename"=w131) -> ("Filename Out"=w130:path, "exists?"=w129:bool)
        n79 = case shown="True" w129 {
          tunnel: w130 -> [_ w139]
          tunnel: [path "" w138] -> w128
          frame False {
          }
          frame True {
            n80 = call "File_checker_and_finder.vi"("Promp if not found"="Please select Template file", "Filename In"=w139) -> ("Filename Out"=w138:path)  [unwired: 1 out]
          }
        }
        n81 = local write "Template"(w128) -> ()
      }
      frame "Read Template File" {
        n82 = local read "Template"() -> (w141:path)
        "Last used Template" <- w141
        n83 = call "Load_Template_Globals.vi"("Channel Names"=w143, "Template-read"=w141) -> ("Valid Template File?"=w142:bool)
        n84 = case shown="True" w142 {
          tunnel: w141 -> [_ w149]
          frame False {
          }
          frame True {
            n85 = global read "Results_plotter_Global.vi" "Tolerances"() -> (w153:string[])
            n86 = call "Read_Write_Template.vi"("Template File"=w149, "Mode"=Global_mode."Read Global", "Data type"="Log Folder Name" ("Variable name")) -> ("Single Value Out"=w151:string)  [unwired: 5 in, 7 out]
            n87 = Fract/Exp String To Number(string=w153) -> (number=→"Tolerances":dbl[])  [unwired: 4 out]
            n88 = String To Path(string=w151) -> (path=w148:path)
            n89 = local write "Job Directory"(w148) -> ()
          }
        }
      }
      frame "What file to start with" {
        n90 = local read "Result files to read"() -> (w160:path[])
        n91 = Array Size(array=w160) -> (size(s)=w159:i32)
        n92 = Greater Than 0?(x=w159) -> (x > 0?=w156:bool)
        n93 = Select(t="Which file to read next", s=w156, f="More files options") -> (s? t:f=w155:string)
      }
      frame "More files options" {
        n94 = call <vilib>:"Three Button Dialog.vi"("Right Button Text (\"Cancel\")"="A entire Folder" ("F button name (\"Cancel\")"), "Center Button Text (\"No\")"="Selection of files in Folder" ("T button name (\"OK\")"), "Left Button Text (\"Yes\")"="A Data File" ("T button name (\"OK\")"), "message"="Where is the data to come from?") -> ("Which Button?"=w169:T11)  [unwired: 1 in, 6 out]
        n95 = case shown="\"Left Button\", Default" w169 {
          tunnel: ["Choose Results File" "Selection of files in Folder" "Choose a Folder"] -> w170
          frame "Left Button", Default {
          }
          frame "Center Button" {
          }
          frame "Right Button" {
          }
        }
      }
      frame "Choose Results File" {
        (unwired) T12."existing file" ("select mode (2)")
        n96 = local read "Choosen Path"() -> (w178:path)
        n97 = File Dialog(7:"Please Choose a Results File" ("Promp if not found"), 11:w178) -> (1:w180:bool, 3:w179:path)  [unwired: 1 in, 6 out]
        "Choosen Path" <- w179
        n98 = case shown="False" w180 {
          tunnel: w179 -> [w187 _]
          frame False {
            n99 = local read "Result files to read"() -> (w188:path[])
            n100 = Build Array (concatenate)(w188, w187) -> (w189:path[])
            n101 = local write "Result files to read"(w189) -> ()
          }
          frame True {
          }
        }
      }
      frame "Choose a Folder" {
        n102 = local read "Choosen Path"() -> (w191:path)
        n103 = File Dialog(7:"Please Choose the folder that contains the Results files to be plotted" ("prompt"), 11:w191) -> (3:w190:path)  [unwired: 1 in, 7 out]
        n104 = local write "Choosen Path"(w190) -> ()
        n105 = call "Get_folder_and_filenames.vi"("file path (dialog if empty)"=w190) -> ("Files"=w192:path[])  [unwired: 1 out]
        n106 = for {
          shift-right: [w211] -> w193
          shift-left: "Result files to read" -> [w210]
          tunnel: w192 -> [w208] mode=indexing
          n107 = Search 1D Array(1D array=w210, element=w208) -> (index of element=w209:i32)  [unwired: 1 out]
          n108 = Strip Path(path=w208) -> (name=w207:string)  [unwired: 1 out]
          n109 = Less Than 0?(x=w209) -> (x < 0?=w206:bool)
          n110 = call "Add_filename_suffix.vi"("Filename"=w207) -> ("Original Suffix"=w204:string)  [unwired: 1 in, 3 out]
          n111 = call "Match_Pat_Case_In.vi"("String to match"=".jpg" ("x"), "String"=w204) -> ("offset past match"=w202:i32)  [unwired: 1 in, 3 out]
          n112 = Less Than 0?(x=w202) -> (x < 0?=w201:bool)
          n113 = And(x=w206, y=w201) -> (x .and. y?=w205:bool)
          n114 = case shown="True" w205 {
            tunnel: w210 -> [w212 w215]
            tunnel: w208 -> [_ w214]
            tunnel: [w212 w213] -> w211
            frame False {
            }
            frame True {
              n115 = Build Array (concatenate)(w215, w214) -> (w213:path[])
            }
          }
        }
        n116 = local write "Result files to read"(w193) -> ()
      }
      frame "Selection of files in Folder" {
        n117 = local read "Choosen Path"() -> (w217:path)
        n118 = local read "Result files to read"() -> (w220:path[])
        n119 = File Dialog(7:"Please Choose the folder that contains the Results files to be plotted" ("prompt"), 11:w217) -> (3:w216:path)  [unwired: 1 in, 7 out]
        n120 = call "Get_folder_and_filenames.vi"("file path (dialog if empty)"=w216) -> ("Files"=w222:path[])  [unwired: 1 out]
        n121 = local write "Choosen Path"(w216) -> ()
        n122 = for {
          tunnel: w222 -> [w245] mode=indexing
          tunnel: [w244] -> w225 mode=indexing
          n123 = Strip Path(path=w245) -> (name=w244:string)  [unwired: 1 out]
        }
        n124 = call "Select_Strings.vi"("Available Ch names"=w225, "Message"="Please select the desired data files", "Selector mode"=T6."Zero or more") -> ("Ch Indicies Choosen"=w223:i32[])  [unwired: 1 in, 4 out]
        n125 = for {
          tunnel: w223 -> [w243] mode=indexing
          tunnel: w222 -> [w242]
          tunnel: [w241] -> w218 mode=indexing
          n126 = Index Array(array=w242, index=w243) -> (element=w241:path)
        }
        n127 = for {
          shift-right: [w236] -> w219
          shift-left: w220 -> [w235]
          tunnel: w218 -> [w234] mode=indexing
          n128 = Search 1D Array(1D array=w235, element=w234) -> (index of element=w233:i32)  [unwired: 1 out]
          n129 = Less Than 0?(x=w233) -> (x < 0?=w232:bool)
          n130 = case shown="True" w232 {
            tunnel: w235 -> [w237 w240]
            tunnel: w234 -> [_ w239]
            tunnel: [w237 w238] -> w236
            frame False {
            }
            frame True {
              n131 = Build Array (concatenate)(w240, w239) -> (w238:path[])
            }
          }
        }
        n132 = local write "Result files to read"(w219) -> ()
      }
      frame "Which file to read next" {
        n133 = local read "Result files to read"() -> (w255:path[])
        n134 = local read "File Index"() -> (w252:i32)
        n135 = Array Size(array=w255) -> (size(s)=w253:i32)
        n136 = Equal?(x=w253, y=w252) -> (x = y?=w251:bool)
        n137 = case shown="False" w251 {
          tunnel: w255 -> [w261 _]
          tunnel: [w262 "Load Selectors"] -> w254
          tunnel: w252 -> [w260 w274]
          tunnel: [w259 w274] -> w247
          frame False {
            n138 = Index Array(array=w261, index=w260) -> (element=w263:path)
            n139 = Search 1D Array(1D array="Results files choosen", element=w263) -> (index of element=w265:i32)  [unwired: 1 out]
            n140 = call "Add_filename_suffix.vi"() -> ()  [unwired: 2 in, 4 out]
            n141 = case shown="-1" w265 {
              tunnel: "Results files choosen" -> [_ w273]
              tunnel: w263 -> [w269 w272]
              tunnel: ["Which file to read next" "Load Data"] -> w262
              frame 0, Default {
                n142 = Format Into String(format string="The filename\n \"%s\"\n has already been chosen" ("Format String"), w269) -> (resulting string=w267:string)  [unwired: 2 in, 1 out]
                n143 = One Button Dialog(message=w267) -> ()  [unwired: 2 out]
              }
              frame -1 {
                n144 = Build Array (concatenate)(w273, w272) -> (w271:path[])
                n145 = local write "Results files choosen"(w271) -> ()
              }
            }
            n146 = local write "Results file"(w263) -> ()
            n147 = Increment(x=w260) -> (x+1=w259:i32)
          }
          frame True {
          }
        }
        n148 = local read "stop"() -> (w250:bool)
        n149 = Decrement(x=w247) -> (x-1=w246:i32)
        n150 = Build Array(w246) -> (w248:i32[])
        n151 = Not(x=w250) -> (.not. x?=w249:bool)
        n152 = local write "File Index"(w247) -> ()
        n153 = property on="Result files to read" class="Arr (strict)"("Index Values"=w248) -> ()  [unwired: 2 in, 2 out]
      }
      frame "Load Data" {
        n154 = stacked-sequence {
          seq-local: [w288 _] -> [_ w348]
          seq-local: [w287 _] -> [_ w353]
          seq-local: [w286 _] -> [_ w352]
          seq-local: [w284 _] -> [_ w351]
          tunnel: [TRUE _] -> w283
          tunnel: w282 -> [w302 w354]
          tunnel: w281 -> [w301 _]
          tunnel: [w300 _] -> w280
          tunnel: [w299 _] -> w279
          tunnel: [w298 _] -> w278
          tunnel: w277 -> [w297 _]
          tunnel: ["Which file to read next" _] -> w276
          frame #0 {
            w291 = TRUE  # Add Extra Channels?
            n155 = local read "Template"() -> (w295:path)
            n156 = call "Read_Data_file.vi"("Results file"="Results file", "Add Extra Channels?"=w291, "Template File"=w295, "Desired File Types"="File Types to Read") -> ("Row numbers"=w286:i32[], "Template File Out"=w292:path, "Filetype"=w287:string, "Results file Out"=w288:path, "Ch names Out"=w293:string[], "Channel Values Out"=w289:string[][])  [unwired: 1 in, 9 out]
            n157 = local write "Template"(w292) -> ()
            n158 = Array Size(array=w293) -> (size(s)=w294:i32)
            n159 = Greater Than 0?(x=w294) -> (x > 0?=w284:bool)
            n160 = case shown="True" w284 {
              tunnel: w302 -> [w304 w318]
              tunnel: w301 -> [w306 w312]
              tunnel: w289 -> [_ w310]
              tunnel: [w304 w308] -> w300
              tunnel: [w306 w316] -> w299
              tunnel: [w305 w307] -> w298
              tunnel: w297 -> [w305 _]
              tunnel: w293 -> [_ w311]
              frame False {
              }
              frame True {
                n161 = for {
                  tunnel: w310 -> [w320] mode=indexing
                  tunnel: [w319] -> w309 mode=indexing
                  n162 = for {
                    tunnel: w320 -> [w322] mode=indexing
                    tunnel: [w321] -> w319 mode=indexing
                    n163 = call "Fast_string_Replace.vi"("Replace match with:"="[", "Input String"=w322, "regular expression"="(") -> ("Output String"=w323:string)  [unwired: 2 out]
                    n164 = call "Fast_string_Replace.vi"("Replace match with:"="]", "Input String"=w323, "regular expression"=")") -> ("Output String"=w321:string)  [unwired: 2 out]
                  }
                }
                n165 = call "Merge_channel_names.vi"("Preferred Channel array"=w312, "Channel array"=w311) -> ("Merged Channels"=w316:string[], "Preferred Channels Changed?"=w314:bool, "Channel Array Changed?"=w315:bool)
                n166 = for {
                  tunnel: w316 -> [w345] mode=indexing
                  tunnel: [w342] -> w307 mode=indexing
                  n167 = call "Fast_string_Replace.vi"("Replace match with:"=" ", "Input String"=w345, "regular expression"=":") -> ("Output String"=w341:string)  [unwired: 2 out]
                  n168 = call "Fast_string_Replace.vi"("Replace match with:"=" ", "Input String"=w341, "regular expression"="  ") -> ("Output String"=w340:string)  [unwired: 2 out]
                  n169 = call <vilib>:"Trim Whitespace.vi"("string"=w340) -> ("trimmed string"=w342:string)  [unwired: 1 in]
                }
                n170 = case shown="True" w314 {
                  tunnel: w318 -> [w333 w335]
                  tunnel: w312 -> [_ w337]
                  tunnel: [w333 w334] -> w313
                  tunnel: w316 -> [_ w336]
                  frame False {
                  }
                  frame True {
                    n171 = call "Merge_2D_values.vi"("Values In"=w335, "Present Channels"=w337, "Desired Channels"=w336) -> ("Values Out"=w334:string[][])
                  }
                }
                n172 = case shown="True" w315 {
                  tunnel: [w328 w332] -> w317
                  tunnel: w311 -> [_ w331]
                  tunnel: w309 -> [w328 w330]
                  tunnel: w316 -> [_ w329]
                  frame False {
                  }
                  frame True {
                    n173 = call "Merge_2D_values.vi"("Values In"=w330, "Present Channels"=w331, "Desired Channels"=w329) -> ("Values Out"=w332:string[][])
                  }
                }
                n174 = global write "Results_plotter_Global.vi" "Channel names"(w307) -> ()
                n175 = Build Array (concatenate)(w313, w317) -> (w308:string[][])
                n176 = global write "Results_plotter_Global.vi" "All Data"(w308) -> ()
              }
            }
          }
          frame #1 {
            n177 = local read "File Index"() -> (w350:i32)
            n178 = Decrement(x=w350) -> (x-1=w349:i32)
            n179 = local read "Result files to read"() -> (w347:path[])
            n180 = case shown="True" w351 {
              tunnel: w354 -> [_ w367]
              tunnel: w353 -> [_ w365]
              tunnel: w352 -> [_ w363]
              tunnel: w349 -> [w355 w361]
              tunnel: w348 -> [_ w360]
              tunnel: w347 -> [w357 w362]
              tunnel: [w356 w359] -> w346
              frame False {
                n181 = Delete From Array(array=w357, length=1, index=w355) -> (array with subset deleted=w356:path[])  [unwired: 1 out]
                n182 = local write "File Index"(w355) -> ()
              }
              frame True {
                n183 = Array Size(array=w367) -> (size(s)=w369:i32[])
                n184 = Index Array(array=w369, index=0 ("Index")) -> (element=w366:i32)
                n185 = for {
                  tunnel: w361 -> [w386]
                  tunnel: [w385] -> w371 mode=indexing
                  tunnel: w366 -> [w382]
                  tunnel: w363 -> [w381] mode=indexing
                  i -> [w383]
                  n186 = Add(x=w383, y=w382) -> (x+y=w384:i32)
                  n187 = Build Array(w386, w381, w384) -> (w385:i32[])
                }
                n188 = case shown="1, Default" w361 {
                  tunnel: w371 -> [w374 w379]
                  tunnel: [w374 w378] -> w370
                  tunnel: w365 -> [w373 w377]
                  tunnel: [w372 w375] -> w364
                  frame 0 {
                    n189 = Build Array(w373) -> (w372:string[])
                  }
                  frame 1, Default {
                    n190 = global read "Results_plotter_Global.vi" "Row Reference"() -> (w380:i32[][])
                    n191 = local read "Filetype"() -> (w376:string[])
                    n192 = Build Array (concatenate)(w376, w377) -> (w375:string[])
                    n193 = Build Array (concatenate)(w380, w379) -> (w378:i32[][])
                  }
                }
                "Filetype" <- w364
                n194 = Replace Array Subset(array=w362, new element=w360, index=w361) -> (w359:path[])
                n195 = global write "Results_plotter_Global.vi" "Row Reference"(w370) -> ()
              }
            }
            n196 = local write "Result files to read"(w346) -> ()
          }
        }
      }
      frame "Load Selectors" {
        n197 = while {
          shift-right: [w407] -> w392
          shift-left: _ -> [w409]
          tunnel: [w409] -> w391
          tunnel: w387 -> [w407]
          stop <- FALSE continue-if-true
        }
        n198 = Array Size(array=w399) -> (size(s)=w398:i32[])
        n199 = local read "Tolerances"() -> (w395:dbl[])
        n200 = Index Array(array=w398, index=0 ("Index")) -> (element=→"nRows":i32)
        n201 = Equal?(x=w392, y=w391) -> (x = y?=w390:bool)
        n202 = Build Array (concatenate)("Don't Filter" ("Input Element"), w387) -> (w404:string[])
        n203 = Array Size(array=w387) -> (size(s)=w401:i32)
        n204 = Array Size(array=w395) -> (size(s)=w400:i32)
        n205 = property on="Multi Ordinate" class="LstBox (strict)"("Item Names"=w387) -> ()  [unwired: 2 in, 2 out]
        n206 = property on="Z Ch Name" class="Ring (strict)"("Strings []"=w387) -> ()  [unwired: 2 in, 2 out]
        n207 = property on="Y Ch Name" class="Ring (strict)"("Strings []"=w387) -> ()  [unwired: 2 in, 2 out]
        n208 = property on="X Ch Name" class="Ring (strict)"("Strings []"=w387) -> ()  [unwired: 2 in, 2 out]
        n209 = property on="X Axis" class="Ring (strict)"("Strings []"=w387) -> ()  [unwired: 2 in, 2 out]
        n210 = property on="Ordinate" class="Ring (strict)"("Strings []"=w387) -> ()  [unwired: 2 in, 2 out]
        n211 = property on="Filter on column 1:" class="Ring (strict)"("Strings []"=w404) -> ()  [unwired: 2 in, 2 out]
        n212 = Not Equal?(x=w401, y=w400) -> (x != y?=w402:bool)
        n213 = case shown="True" w402 {
          tunnel: w401 -> [_ w416]
          tunnel: w400 -> [_ w415]
          tunnel: w395 -> [_ w412]
          frame False {
          }
          frame True {
            n214 = Subtract(x=w416, y=w415) -> (x-y=w414:i32)
            n215 = Initialize Array(1.0 ("Element Data"), w414) -> (w411:dbl[])
            n216 = Build Array (concatenate)(w412, w411) -> (w410:dbl[])
            n217 = local write "Tolerances"(w410) -> ()
          }
        }
        n218 = global write "Results_plotter_Global.vi" "First Loop"(TRUE) -> ()
        n219 = Select(t="What is present?", s=w390, f="Set Axis Channels") -> (s? t:f=w394:string)
      }
      frame "Set Axis Channels" {
        n220 = Array Size(array=w423) -> (size(s)=w422:i32)
        n221 = Build Array("X" ("regular expression"), "Y" ("regular expression"), "Z" ("regular expression")) -> (w417:string[])
        n222 = Decrement(x=w422) -> (x-1=w421:i32)
        n223 = for {
          tunnel: w423 -> [w435]
          tunnel: w421 -> [w434]
          tunnel: w417 -> [w433] mode=indexing
          i -> [w429]
          n224 = while {
            tunnel: w435 -> [w449] mode=indexing
            tunnel: w434 -> [w448]
            tunnel: w433 -> [w446]
            tunnel: [w439] -> w432
            tunnel: [w444] -> w431
            i -> [w444]
            stop <- w447 continue-if-true
            n225 = call "Match_Pat_Case_In.vi"("String to match"=w446, "String"=w449) -> ("offset past match"=w443:i32)  [unwired: 1 in, 3 out]
            n226 = In Range and Coerce(upper limit=4, x=w443, lower limit=0) -> (In Range?=w440:bool)  [unwired: 1 out]
            n227 = Less?(x=w444, y=w448) -> (x < y?=w445:bool)
            n228 = Not(x=w440) -> (.not. x?=w439:bool)
            n229 = And(x=w439, y=w445) -> (x .and. y?=w447:bool)
          }
          n230 = Select(t=0, s=w432, f=w431) -> (s? t:f=w428:i32)
          n231 = case shown="1" w429 {
            tunnel: w428 -> [w436 w437 w438]
            frame 0, Default {
              n232 = local write "X Ch Name"(w436) -> ()
            }
            frame 1 {
              n233 = local write "Y Ch Name"(w437) -> ()
            }
            frame 2 {
              n234 = local write "Z Ch Name"(w438) -> ()
            }
          }
        }
      }
      frame "What is present?" {
        n235 = case shown="True" "Show Results Space Analysis" {
          tunnel: w453 -> [_ w457]
          tunnel: w452 -> [_ w456]
          frame False {
          }
          frame True {
            n236 = stacked-sequence {
              tunnel: w457 -> [w461]
              tunnel: w456 -> [w460]
              frame #0 {
                w458 = FALSE  # Summarise All
                n237 = call "Summarise.vi"("Channel Names"=w461, "Data"=w460, "Summarise All"=w458) -> ("Summary"=w459:string[][])  [unwired: 2 in]
                n238 = call "Results_Space_Analysis.vi"("Table"=w459) -> ()
              }
            }
          }
        }
      }
      frame "Ordinate Selector Type" {
        n239 = while {
          tunnel: [w480] -> w471
          shift-left: _ -> [w480]
          shift-right: ["Slice mode"] -> w472
          stop <- FALSE continue-if-true
          "Previous slice mode" <- w480
        }
        n240 = Not(x="Multi Ordinate?") -> (.not. x?=w466:bool)
        n241 = property on="Multi Ordinate" class="LstBox (strict)"("Visible"="Multi Ordinate?") -> ()  [unwired: 2 in, 2 out]
        n242 = property on="Ordinate Name" class="Str"("Visible"="Multi Ordinate?") -> ()  [unwired: 2 in, 2 out]
        n243 = property on="Ordinate" class="Ring (strict)"("Visible"=w466) -> ()  [unwired: 2 in, 2 out]
        n244 = property on="First Add label" class="Str"("Visible"=w466) -> ()  [unwired: 2 in, 2 out]
        n245 = property on="2nd Add label" class="Str"("Visible"=w466) -> ()  [unwired: 2 in, 2 out]
        n246 = property on="Additional Y Values" class="Arr (strict)"("Visible"=w466) -> ()  [unwired: 2 in, 2 out]
        n247 = property on="Additional X Values" class="Arr (strict)"("Visible"=w466) -> ()  [unwired: 2 in, 2 out]
        n248 = Not Equal?(x=w472, y=w471) -> (x != y?=w463:bool)
        n249 = local read "Intensity Plot?"() -> (w470:bool)
        n250 = Or(x=w463, y="Update") -> (x .or. y?=w464:bool)
        n251 = global read "Results_plotter_Global.vi" "First Loop"() -> (w467:bool)
        n252 = case shown="False" "Multi Ordinate?" {
          frame False {
            n253 = Build Array("Ordinate") -> (w482:u16[])
            n254 = local write "Multi Ordinate"(w482) -> ()
          }
          frame True {
          }
        }
        n255 = Compound Arithmetic op=AND(invert w467, w464, w470) -> (w469:bool)
        "Slice mode Change?" <- w469
        n256 = Select(t="Change Slice mode", s=w469, f="Which rows are Non-Blank?") -> (s? t:f=w473:string)
      }
      frame "Change Slice mode" {
        n257 = local read "Previous slice mode"() -> (w486:T3)
        n258 = local read "Slice mode"() -> (w500:T3)
        n259 = case shown="\"YX Slice (Plan)\"" w500 {
          tunnel: [w512 w517 w524 w529 w536 w542] -> w499
          tunnel: "Y Ch Name" -> [w510 w517 w524 w530 w535 w540]
          tunnel: "X Ch Name" -> [w512 w516 w523 w528 w536 w541]
          tunnel: [w511 w518 w523 w528 w535 w540] -> w490
          tunnel: "Z Ch Name" -> [w511 w518 w522 w529 w534 w542]
          tunnel: [w510 w516 w522 w530 w534 w541] -> w488
          tunnel: w486 -> [w509 w514 w520 w526 w533 w538]
          tunnel: [w507 w513 w519 w525 w532 w537] -> w485
          frame "XY Slice (Plan)" {
            n260 = Equal?(x=Plot_Slice."YX Slice (Plan)" ("Previous slice mode"), y=w509) -> (x = y?=w507:bool)
          }
          frame "YX Slice (Plan)" {
            n261 = Equal?(x=Plot_Slice."XY Slice (Plan)" ("Previous slice mode"), y=w514) -> (x = y?=w513:bool)
          }
          frame "YZ Slice (Cross)" {
            n262 = Equal?(x=Plot_Slice."ZY Slice (Cross)" ("Previous slice mode"), y=w520) -> (x = y?=w519:bool)
          }
          frame "ZY Slice (Cross)" {
            n263 = Equal?(x=Plot_Slice."YZ Slice (Cross)" ("Previous slice mode"), y=w526) -> (x = y?=w525:bool)
          }
          frame "XZ Slice (Side)" {
            n264 = Equal?(x=Plot_Slice."ZX Slice (Side)" ("Previous slice mode"), y=w533) -> (x = y?=w532:bool)
          }
          frame "ZX Slice (Side)" {
            n265 = Equal?(x=Plot_Slice."XZ Slice (Side)" ("Previous slice mode"), y=w538) -> (x = y?=w537:bool)
          }
        }
        n266 = case shown="True" w485 {
          frame False {
          }
          frame True {
            n267 = local read "Transpose"() -> (w506:bool)
            n268 = Not(x=w506) -> (.not. x?=w505:bool)
            n269 = local write "Transpose"(w505) -> ()
          }
        }
        n270 = local write "Update"(FALSE ("Update")) -> ()
        n271 = Increment(x=w490) -> (x+1=w493:u16)
        n272 = Increment(x=w488) -> (x+1=w492:u16)
        n273 = local read "Filter Array"() -> (w497:u16[])
        n274 = Array Subset(array=w497, index=2 ("Array Index")) -> (w495:u16[])  [unwired: 1 in]
        n275 = Build Array (concatenate)(w493, w492, w495) -> (w494:u16[])
        n276 = local write "Filter Array"(w494) -> ()
        n277 = local write "Absisca"(w499) -> ()
      }
      frame "Which rows are Non-Blank?" {
        n278 = while {
          tunnel: [w559] -> w553
          tunnel: [w560] -> w554
          shift-left: _ -> [w561]
          shift-right: [w562] -> w546
          shift-left: _ -> [w564]
          shift-right: [w563] -> _
          stop <- FALSE continue-if-true
          n279 = local read "Multi Ordinate"() -> (w562:i32[])
          n280 = local read "Absisca"() -> (w563:u16)
          n281 = Equal?(x=w563, y=w564) -> (x = y?=w560:bool)
          n282 = Equal?(x=w562, y=w561) -> (x = y?=w559:bool)
        }
        n283 = global read "Results_plotter_Global.vi" "First Loop"() -> (w548:bool)
        n284 = Compound Arithmetic op=AND(invert w548, w554, w553) -> (w552:bool)
        n285 = Array Size(array=w546) -> (size(s)=w545:i32)
        n286 = Greater?(x=w545, y=1) -> (0:w543:bool)
        n287 = global write "Results_plotter_Global.vi" "Multi Ordinate?"(w543) -> ()
        n288 = Select(t="Create Selectors", s=w552, f="Evaluate Blank Rows") -> (s? t:f=w549:string)
      }
      frame "Evaluate Blank Rows" {
        n289 = local read "Multi Ordinate"() -> (w566:i32[])
        n290 = local read "Absisca"() -> (w567:u16)
        n291 = for {
          tunnel: w568 -> [w574] mode=indexing
          tunnel: w567 -> [w577]
          tunnel: w566 -> [w576]
          tunnel: [w573] -> w565 mode=indexing
          n292 = Index Array(array=w574, index=w577) -> (element=w578:string)
          n293 = call "Convert_to_number.vi"("string"=w578) -> ("Number"=w579:dbl)  [unwired: 1 out]
          n294 = Not A Number/Path/Refnum?(number/path/refnum=w579) -> (NaN/Path/Refnum?=w575:bool)
          n295 = case shown="False" w575 {
            tunnel: w576 -> [w583 _]
            tunnel: w574 -> [w582 _]
            tunnel: [w580 FALSE] -> w573
            frame False {
              n296 = for {
                tunnel: w583 -> [w589] mode=indexing
                tunnel: w582 -> [w587]
                tunnel: [w584] -> w581 mode=indexing
                n297 = Index Array(array=w587, index=w589) -> (element=w588:string)
                n298 = call "Convert_to_number.vi"("string"=w588) -> ("Number"=w586:dbl)  [unwired: 1 out]
                n299 = Not A Number/Path/Refnum?(number/path/refnum=w586) -> (NaN/Path/Refnum?=w585:bool)
                n300 = Not(x=w585) -> (.not. x?=w584:bool)
              }
              n301 = Or Array Elements(Boolean array=w581) -> (logical OR=w580:bool)
            }
            frame True {
            }
          }
        }
        "Non-Blank Rows" <- w565
      }
      frame "Create Selectors" {
        n302 = local read "Non-Blank Rows"() -> (w594:bool[])
        n303 = local read "Tolerances"() -> (w592:dbl[])
        n304 = global read "Results_plotter_Global.vi" "Precision"() -> (w591:string[])
        n305 = Array Size(array=w602) -> (size(s)=w601:i32[])
        n306 = Index Array(array=w601, index=0 ("Index")) -> (element=w604:i32)
        n307 = for {
          tunnel: w602 -> [w620]
          tunnel: "Filter Array" -> [w612] mode=indexing
          shift-right: [w619] -> w593
          shift-left: _ -> [w617]
          tunnel: w604 -> [w618]
          tunnel: [w615] -> w599 mode=indexing
          tunnel: w594 -> [w614]
          tunnel: w592 -> [w613]
          tunnel: w591 -> [w610]
          i -> [w616]
          n308 = Decrement(x=w612) -> (x-1=w609:u16)
          n309 = Index Array(array=w610, index=w609) -> (element=w608:string)
          n310 = Index Array(array=w613, index=w609) -> (element=w611:dbl)
          n311 = case shown="0, Default" w616 {
            tunnel: w620 -> [w633 w669 w710 w751 w792 w835 w876]
            tunnel: w612 -> [w632 w668 w709 w750 w791 w834 w875]
            tunnel: w611 -> [w631 w667 w708 w749 w790 w833 w874]
            tunnel: [w630 w666 w707 w748 w789 w832 w873] -> w619
            tunnel: w618 -> [w628 w665 w706 w747 w788 w831 w872]
            tunnel: w617 -> [_ w664 w705 w746 w787 w830 w871]
            tunnel: w616 -> [w627 w663 w702 w743 w784 w829 w868]
            tunnel: [w623 w658 w701 w742 w783 w824 w867] -> w615
            tunnel: w614 -> [w622 w657 w700 w741 w782 w823 w866]
            tunnel: w608 -> [w621 w656 w699 w740 w781 w822 w865]
            frame 0, Default {
              n312 = case shown="1, Default" w632 {
                tunnel: w633 -> [w639 w649]
                tunnel: w632 -> [w640 w648]
                tunnel: w631 -> [_ w655]
                tunnel: [w635 w652] -> w630
                tunnel: "Filter Bins 1" -> [_ w653]
                tunnel: [string[] [] ("Write Attribute") w654] -> w629
                tunnel: w628 -> [w637 _]
                tunnel: w627 -> [w643 w651]
                tunnel: [i32[] [0] ("Filter Bins Out") w650] -> w625
                tunnel: [TRUE ("Unchanged?") w647] -> w623
                tunnel: w622 -> [_ w646]
                tunnel: w621 -> [_ w645]
                frame 0 {
                  n313 = call "Create_filter_points.vi"("Channel to Filter On"=w640, "Index"=w643, "Ch Values In"=w639) -> ()  [unwired: 4 in, 4 out]
                  n314 = Initialize Array(TRUE, w637) -> (w636:bool[])
                  n315 = Build Array(w636) -> (w635:bool[][])
                }
                frame 1, Default {
                  n316 = call "Create_filter_points.vi"("Non-Blank Rows"=w646, "Precision"=w645, "Channel to Filter On"=w648, "Tolerance"=w655, "Index"=w651, "Filter Bins 1"=w653, "Ch Values In"=w649) -> ("Unchanged?"=w647:bool, "Accept array"=w652:bool[][], "Filter Bins Out"=w650:i32[], "Bin Names"=w654:string[])
                }
              }
              n317 = Equal?(x="Filter Bins 1", y=w625) -> (x = y?=w624:bool)
              n318 = case shown="False" w624 {
                tunnel: w625 -> [w634 _]
                frame False {
                  n319 = local write "Filter Bins 1"(w634) -> ()
                }
                frame True {
                }
              }
              n320 = property on="Filter bins 1" class="LstBox (strict)"("Item Names"=w629) -> ()  [unwired: 2 in, 2 out]
            }
            frame 1 {
              n321 = case shown="0" w668 {
                tunnel: w669 -> [_ w681]
                tunnel: w668 -> [w672 w680]
                tunnel: w667 -> [_ w688]
                tunnel: [w676 w684] -> w666
                tunnel: "Filter Bins 2" -> [_ w686]
                tunnel: [string[] [] ("Write Attribute") w690] -> w662
                tunnel: w665 -> [_ _]
                tunnel: w664 -> [w676 w689]
                tunnel: w663 -> [w675 w687]
                tunnel: [i32[] [0] ("Filter Bins Out") w682] -> w661
                tunnel: [TRUE ("Unchanged?") w679] -> w658
                tunnel: w657 -> [_ w678]
                tunnel: w656 -> [_ w677]
                frame 0 {
                  n322 = call "Create_filter_points.vi"("Channel to Filter On"=w672, "Index"=w675) -> ()  [unwired: 5 in, 4 out]
                }
                frame 1, Default {
                  n323 = call "Create_filter_points.vi"("Non-Blank Rows"=w678, "Precision"=w677, "Channel to Filter On"=w680, "Tolerance"=w688, "Index"=w687, "Filter Bins 1"=w686, "Ch Values In"=w681) -> ("Unchanged?"=w679:bool, "Accept array"=w685:bool[][], "Filter Bins Out"=w682:i32[], "Bin Names"=w690:string[])
                  n324 = for {
                    tunnel: w689 -> [w695]
                    tunnel: w685 -> [w694] mode=indexing
                    shift-right: [w691] -> w684
                    shift-left: bool[][] [] -> [w693]
                    n325 = for {
                      tunnel: w694 -> [w698]
                      tunnel: w695 -> [w697] mode=indexing
                      tunnel: [w696] -> _ mode=indexing
                      tunnel: [w696] -> w692 mode=indexing
                      n326 = And(x=w698, y=w697) -> (x .and. y?=w696:bool[])
                    }
                    n327 = Build Array (concatenate)(w693, w692) -> (w691:bool[][])
                  }
                }
              }
              n328 = Equal?(x="Filter Bins 2", y=w661) -> (x = y?=w659:bool)
              n329 = case shown="False" w659 {
                tunnel: w661 -> [w670 _]
                frame False {
                  n330 = local write "Filter Bins 2"(w670) -> ()
                }
                frame True {
                }
              }
              n331 = property on="Filter Bins 2" class="LstBox (strict)"("Item Names"=w662) -> ()  [unwired: 2 in, 2 out]
            }
            frame 2 {
              n332 = case shown="0" w709 {
                tunnel: w710 -> [_ w720]
                tunnel: w709 -> [w713 w721]
                tunnel: w708 -> [_ w732]
                tunnel: [w716 w733] -> w707
                tunnel: "Filter 3" -> [_ w724]
                tunnel: [string[] [] ("Write Attribute") w735] -> w703
                tunnel: w706 -> [_ _]
                tunnel: w705 -> [w716 w734]
                tunnel: w702 -> [w715 w727]
                tunnel: [TRUE ("Unchanged?") w719] -> w701
                tunnel: w700 -> [_ w718]
                tunnel: w699 -> [_ w717]
                frame 0 {
                  n333 = call "Create_filter_points.vi"("Channel to Filter On"=w713, "Index"=w715) -> ()  [unwired: 5 in, 4 out]
                  n334 = local write "Filter 3"(0) -> ()
                }
                frame 1, Default {
                  n335 = Build Array(w724) -> (w731:u16[])
                  n336 = call "Create_filter_points.vi"("Non-Blank Rows"=w718, "Precision"=w717, "Channel to Filter On"=w721, "Tolerance"=w732, "Index"=w727, "Filter Bins 1"=w731, "Ch Values In"=w720) -> ("Unchanged?"=w719:bool, "Accept array"=w729:bool[][], "Filter Bins Out"=w725:i32[], "Bin Names"=w735:string[])
                  n337 = Index Array(array=w725, index=0 ("Index")) -> (element=w722:i32)
                  n338 = Index Array(array=w729, index (row)=0 ("Index")) -> (element=w728:bool[])  [unwired: 1 in]
                  n339 = Equal?(x=w724, y=w722) -> (x = y?=w723:bool)
                  n340 = case shown="True" w723 {
                    tunnel: w722 -> [w736 _]
                    frame False {
                      n341 = local write "Filter 3"(w736) -> ()
                    }
                    frame True {
                    }
                  }
                  n342 = for {
                    tunnel: w728 -> [w739]
                    tunnel: w734 -> [w738] mode=indexing
                    tunnel: [w737] -> w733 mode=indexing
                    n343 = And(x=w739, y=w738) -> (x .and. y?=w737:bool[])
                  }
                }
              }
              n344 = property on="Filter 3" class="Ring (strict)"("Strings []"=w703) -> ()  [unwired: 2 in, 2 out]
            }
            frame 3 {
              n345 = case shown="1, Default" w750 {
                tunnel: w751 -> [_ w762]
                tunnel: w750 -> [w754 w761]
                tunnel: w749 -> [_ w773]
                tunnel: [w757 w774] -> w748
                tunnel: "Filter 4" -> [_ w765]
                tunnel: [string[] [] ("Write Attribute") w776] -> w744
                tunnel: w747 -> [_ _]
                tunnel: w746 -> [w757 w775]
                tunnel: w743 -> [w756 w768]
                tunnel: [TRUE ("Unchanged?") w760] -> w742
                tunnel: w741 -> [_ w759]
                tunnel: w740 -> [_ w758]
                frame 0 {
                  n346 = call "Create_filter_points.vi"("Channel to Filter On"=w754, "Index"=w756) -> ()  [unwired: 5 in, 4 out]
                  n347 = local write "Filter 4"(0) -> ()
                }
                frame 1, Default {
                  n348 = Build Array(w765) -> (w772:u16[])
                  n349 = call "Create_filter_points.vi"("Non-Blank Rows"=w759, "Precision"=w758, "Channel to Filter On"=w761, "Tolerance"=w773, "Index"=w768, "Filter Bins 1"=w772, "Ch Values In"=w762) -> ("Unchanged?"=w760:bool, "Accept array"=w770:bool[][], "Filter Bins Out"=w766:i32[], "Bin Names"=w776:string[])
                  n350 = Index Array(array=w766, index=0 ("Index")) -> (element=w764:i32)
                  n351 = Equal?(x=w765, y=w764) -> (x = y?=w763:bool)
                  n352 = Index Array(array=w770, index (row)=0 ("Index")) -> (element=w769:bool[])  [unwired: 1 in]
                  n353 = case shown="False" w763 {
                    tunnel: w764 -> [w777 _]
                    frame False {
                      n354 = local write "Filter 4"(w777) -> ()
                    }
                    frame True {
                    }
                  }
                  n355 = for {
                    tunnel: w769 -> [w780]
                    tunnel: w775 -> [w779] mode=indexing
                    tunnel: [w778] -> w774 mode=indexing
                    n356 = And(x=w780, y=w779) -> (x .and. y?=w778:bool[])
                  }
                }
              }
              n357 = property on="Filter 4" class="Ring (strict)"("Strings []"=w744) -> ()  [unwired: 2 in, 2 out]
            }
            frame 4 {
              n358 = case shown="1, Default" w791 {
                tunnel: w792 -> [_ w803]
                tunnel: w791 -> [w795 w802]
                tunnel: w790 -> [_ w814]
                tunnel: [w798 w815] -> w789
                tunnel: "Filter 5" -> [_ w805]
                tunnel: [string[] [] ("Write Attribute") w817] -> w785
                tunnel: w788 -> [_ _]
                tunnel: w787 -> [w798 w816]
                tunnel: w784 -> [w797 w809]
                tunnel: [TRUE ("Unchanged?") w801] -> w783
                tunnel: w782 -> [_ w800]
                tunnel: w781 -> [_ w799]
                frame 0 {
                  n359 = call "Create_filter_points.vi"("Channel to Filter On"=w795, "Index"=w797) -> ()  [unwired: 5 in, 4 out]
                  n360 = local write "Filter 5"(0) -> ()
                }
                frame 1, Default {
                  n361 = Build Array(w805) -> (w813:u16[])
                  n362 = call "Create_filter_points.vi"("Non-Blank Rows"=w800, "Precision"=w799, "Channel to Filter On"=w802, "Tolerance"=w814, "Index"=w809, "Filter Bins 1"=w813, "Ch Values In"=w803) -> ("Unchanged?"=w801:bool, "Accept array"=w811:bool[][], "Filter Bins Out"=w807:i32[], "Bin Names"=w817:string[])
                  n363 = Index Array(array=w807, index=0 ("Index")) -> (element=w806:i32)
                  n364 = Equal?(x=w805, y=w806) -> (x = y?=w804:bool)
                  n365 = Index Array(array=w811, index (row)=0 ("Index")) -> (element=w810:bool[])  [unwired: 1 in]
                  n366 = case shown="False" w804 {
                    tunnel: w806 -> [w818 _]
                    frame False {
                      n367 = local write "Filter 5"(w818) -> ()
                    }
                    frame True {
                    }
                  }
                  n368 = for {
                    tunnel: w810 -> [w821]
                    tunnel: w816 -> [w820] mode=indexing
                    tunnel: [w819] -> w815 mode=indexing
                    n369 = And(x=w821, y=w820) -> (x .and. y?=w819:bool[])
                  }
                }
              }
              n370 = property on="Filter 5" class="Ring (strict)"("Strings []"=w785) -> ()  [unwired: 2 in, 2 out]
            }
            frame 5 {
              n371 = case shown="1, Default" w834 {
                tunnel: w835 -> [_ w852]
                tunnel: w834 -> [w838 w851]
                tunnel: w833 -> [_ w856]
                tunnel: [w842 w843] -> w832
                tunnel: "Single Series" -> [_ w854]
                tunnel: [string[] [] ("Write Attribute") w858] -> w828
                tunnel: w831 -> [_ _]
                tunnel: w830 -> [w842 w857]
                tunnel: w829 -> [w841 w855]
                tunnel: [i32[] [0] ("Filter Bins Out") w853] -> w827
                tunnel: [TRUE ("Unchanged?") w850] -> w824
                tunnel: w823 -> [_ w849]
                tunnel: w822 -> [_ w848]
                frame 0 {
                  n372 = call "Create_filter_points.vi"("Channel to Filter On"=w838, "Index"=w841) -> ()  [unwired: 5 in, 4 out]
                }
                frame 1, Default {
                  n373 = call "Create_filter_points.vi"("Non-Blank Rows"=w849, "Precision"=w848, "Channel to Filter On"=w851, "Tolerance"=w856, "Index"=w855, "Filter Bins 1"=w854, "Ch Values In"=w852) -> ("Unchanged?"=w850:bool, "Accept array"=w845:bool[][], "Filter Bins Out"=w853:i32[], "Bin Names"=w858:string[])
                  n374 = Index Array(array=w845, index (row)=0 ("Index")) -> (element=w846:bool[])  [unwired: 1 in]
                  n375 = for {
                    shift-right: [w859] -> w844
                    shift-left: w846 -> [w861]
                    tunnel: w845 -> [w860] mode=indexing
                    n376 = Or(x=w860, y=w861) -> (x .or. y?=w859:bool[])
                  }
                  n377 = for {
                    tunnel: w844 -> [w864]
                    tunnel: w857 -> [w863] mode=indexing
                    tunnel: [w862] -> w843 mode=indexing
                    n378 = And(x=w864, y=w863) -> (x .and. y?=w862:bool[])
                  }
                }
              }
              n379 = Equal?(x="Single Series", y=w827) -> (x = y?=w825:bool)
              n380 = case shown="False" w825 {
                tunnel: w827 -> [w836 _]
                frame False {
                  n381 = local write "Single Series"(w836) -> ()
                }
                frame True {
                }
              }
              n382 = property on="Single Series" class="LstBox (strict)"("Item Names"=w828) -> ()  [unwired: 2 in, 2 out]
            }
            frame 6 {
              n383 = case shown="1, Default" w875 {
                tunnel: w876 -> [_ w887]
                tunnel: w875 -> [w879 w886]
                tunnel: w874 -> [_ w894]
                tunnel: [w882 w899] -> w873
                tunnel: "Filter 6" -> [_ w889]
                tunnel: [string[] [] ("Write Attribute") w901] -> w869
                tunnel: w872 -> [_ _]
                tunnel: w871 -> [w882 w900]
                tunnel: w868 -> [w881 w893]
                tunnel: [TRUE ("Unchanged?") w885] -> w867
                tunnel: w866 -> [_ w884]
                tunnel: w865 -> [_ w883]
                frame 0 {
                  n384 = call "Create_filter_points.vi"("Channel to Filter On"=w879, "Index"=w881) -> ()  [unwired: 5 in, 4 out]
                  n385 = local write "Filter 6"(0) -> ()
                }
                frame 1, Default {
                  n386 = Build Array(w889) -> (w895:u16[])
                  n387 = call "Create_filter_points.vi"("Non-Blank Rows"=w884, "Precision"=w883, "Channel to Filter On"=w886, "Tolerance"=w894, "Index"=w893, "Filter Bins 1"=w895, "Ch Values In"=w887) -> ("Unchanged?"=w885:bool, "Accept array"=w897:bool[][], "Filter Bins Out"=w891:i32[], "Bin Names"=w901:string[])
                  n388 = Index Array(array=w891, index=0 ("Index")) -> (element=w890:i32)
                  n389 = Equal?(x=w889, y=w890) -> (x = y?=w888:bool)
                  n390 = Index Array(array=w897, index (row)=0 ("Index")) -> (element=w896:bool[])  [unwired: 1 in]
                  n391 = case shown="False" w888 {
                    tunnel: w890 -> [w902 _]
                    frame False {
                      n392 = local write "Filter 6"(w902) -> ()
                    }
                    frame True {
                    }
                  }
                  n393 = for {
                    tunnel: w896 -> [w905]
                    tunnel: w900 -> [w904] mode=indexing
                    tunnel: [w903] -> w899 mode=indexing
                    n394 = And(x=w905, y=w904) -> (x .and. y?=w903:bool[])
                  }
                }
              }
              n395 = property on="Filter 6" class="Ring (strict)"("Strings []"=w869) -> ()  [unwired: 2 in, 2 out]
            }
          }
        }
        "Accept Array" <- w593
        n396 = And Array Elements(Boolean array=w599) -> (logical AND=w598:bool)
        n397 = Select(t="Select all for Filter 2", s=w598, f="Create Selectors") -> (s? t:f=w596:string)
      }
      frame "Select all for Filter 2" {
        n398 = local read "Slice mode Change?"() -> (w915:bool)
        n399 = property on="Filter bins 1" class="LstBox (strict)"() -> ("Item Names"=w911:string[], "Top Row"=w910:i32)  [unwired: 2 in, 2 out]
        n400 = case shown="True" w915 {
          frame False {
          }
          frame True {
            n401 = property on="Filter Bins 2" class="LstBox (strict)"() -> ("Item Names"=w931:string[])  [unwired: 2 in, 2 out]
            n402 = Array Size(array=w931) -> (size(s)=w930:i32)
            n403 = Build Array("Blanks", "Numeric", "Non Numeric", "Non Blanks", "Show All" ("Input Element")) -> (w924:string[])
            n404 = local read "Filter Bins 1"() -> (w933:i32[])
            n405 = while {
              tunnel: w931 -> [w946] mode=indexing
              tunnel: w930 -> [w949]
              shift-right: [w940] -> w922
              shift-left: i32[] [] -> [w941]
              tunnel: w924 -> [w943]
              i -> [w942]
              stop <- w947 stop-if-true
              n406 = String Subset(string=w946, length (rest)=4 ("length (rest)")) -> (substring=w951:string)  [unwired: 1 out]
              n407 = Match Pattern(string=w946, regular expression=" (") -> (before substring=w944:string)  [unwired: 4 out]
              n408 = Search 1D Array(1D array=w943, element=w944) -> (index of element=w939:i32)  [unwired: 1 out]
              n409 = Equal?(x="NOT ", y=w951) -> (x = y?=w938:bool)
              n410 = Equal?(x=w949, y=w942) -> (x = y?=w948:bool)
              n411 = Less Than 0?(x=w939) -> (x < 0?=w937:bool)
              n412 = Or(x=w938, y=w948) -> (x .or. y?=w947:bool)
              n413 = Compound Arithmetic op=AND(w937, invert w938) -> (w936:bool)
              n414 = case shown="False" w936 {
                tunnel: w942 -> [_ w956]
                tunnel: w941 -> [w953 w955]
                tunnel: [w953 w954] -> w940
                frame False {
                }
                frame True {
                  n415 = Build Array (concatenate)(w955, w956) -> (w954:i32[])
                }
              }
            }
            n416 = Array Size(array=w933) -> (size(s)=w935:i32)
            n417 = case shown="1" w935 {
              tunnel: [w957 w960] -> w934
              tunnel: w933 -> [_ w959]
              tunnel: i32[] [1] ("Filter Bins 1") -> [w957 w958]
              frame 0, Default {
              }
              frame 1 {
                n418 = Index Array(array=w959, index=0 ("Index")) -> (element=w962:i32)
                n419 = Greater Than 0?(x=w962) -> (x > 0?=w961:bool)
                n420 = Select(t=w959, s=w961, f=w958) -> (s? t:f=w960:i32[])
              }
            }
            n421 = local write "Filter Bins 1"(w934) -> ()
            n422 = local write "Filter Bins 2"(w922) -> ()
          }
        }
        n423 = Array Size(array=w911) -> (size(s)=w912:i32)
        n424 = Less?(x=w912, y=w910) -> (x < y?=w913:bool)
        n425 = case shown="True" w913 {
          frame False {
          }
          frame True {
            n426 = property on="Filter bins 1" class="LstBox (strict)"("Top Row"=0 ("Active Row:Active Row Number")) -> ()  [unwired: 2 in, 2 out]
          }
        }
        n427 = property on="Filter Bins 2" class="LstBox (strict)"() -> ("Item Names"=w909:string[], "Top Row"=w907:i32)  [unwired: 2 in, 2 out]
        n428 = Array Size(array=w909) -> (size(s)=w908:i32)
        n429 = Less?(x=w908, y=w907) -> (x < y?=w906:bool)
        n430 = case shown="True" w906 {
          frame False {
          }
          frame True {
            n431 = property on="Filter Bins 2" class="LstBox (strict)"("Top Row"=0 ("Active Row:Active Row Number")) -> ()  [unwired: 2 in, 2 out]
          }
        }
      }
      frame "Re Plot Data?" {
        n432 = while {
          tunnel: [w1010] -> w972
          shift-left: _ -> [w1012]
          shift-right: [w1011] -> _
          tunnel: [w1015] -> w978
          shift-left: _ -> [w1013]
          shift-right: [w1014] -> _
          tunnel: [w1019] -> w980
          shift-left: _ -> [w1018]
          shift-right: [w1017] -> w964
          tunnel: [w1020] -> w981
          shift-left: _ -> [w1022]
          shift-right: [w1021] -> _
          tunnel: [w1024] -> w982
          shift-left: _ -> [w1023]
          shift-right: [w1016] -> _
          tunnel: [w1025] -> w985
          tunnel: [w1026] -> w986
          shift-left: _ -> [w1027]
          shift-right: [w1028] -> _
          shift-left: _ -> [w1030]
          shift-right: [w1029] -> _
          tunnel: [w1031] -> w965
          shift-left: _ -> [w1032]
          shift-right: [w1033] -> _
          tunnel: [w1008] -> w975
          shift-right: [w1005] -> _
          shift-left: _ -> [w1004]
          tunnel: [w1007] -> w974
          shift-right: [w1003] -> _
          shift-left: _ -> [w1006]
          tunnel: [w1000] -> w973
          shift-right: [w1001] -> _
          shift-left: _ -> [w1002]
          shift-right: [w998] -> _
          shift-left: _ -> [w999]
          tunnel: [w997] -> w967
          stop <- FALSE continue-if-true
          n433 = local read "Ordinate Name"() -> (w998:string)
          n434 = local read "Additional X Values"() -> (w1005:dbl[])
          n435 = local read "Additional Y Values"() -> (w1003:dbl[])
          n436 = local read "Intensity Plot?"() -> (w1017:bool)
          n437 = local read "color and symbol"() -> (w1001:bool)
          n438 = local read "Accept Array"() -> (w1033:bool[][])
          n439 = local read "No of Contours"() -> (w1014:i32)
          n440 = local read "Point Size"() -> (w1011:i32)
          n441 = local read "Multi Ordinate"() -> (w1028:i32[])
          n442 = local read "Resolution"() -> (w1021:dbl)
          n443 = local read "Transpose"() -> (w1016:bool)
          n444 = local read "Absisca"() -> (w1029:u16)
          n445 = Equal?(x=w998, y=w999) -> (x = y?=w997:bool)
          n446 = Equal?(x=w1016, y=w1023) -> (x = y?=w1024:bool)
          n447 = Equal?(x=w1001, y=w1002) -> (x = y?=w1000:bool)
          n448 = Equal?(x=w1014, y=w1013) -> (x = y?=w1015:bool)
          n449 = Equal?(x=w1011, y=w1012) -> (x = y?=w1010:bool)
          n450 = Equal?(x=w1021, y=w1022) -> (x = y?=w1020:bool)
          n451 = Equal?(x=w1005, y=w1004) -> (x = y?=w1008:bool)
          n452 = Equal?(x=w1003, y=w1006) -> (x = y?=w1007:bool)
          n453 = Equal?(x=w1029, y=w1030) -> (x = y?=w1026:bool)
          n454 = Equal?(x=w1033, y=w1032) -> (x = y?=w1031:bool)
          n455 = Equal?(x=w1017, y=w1018) -> (x = y?=w1019:bool)
          n456 = Equal?(x=w1028, y=w1027) -> (x = y?=w1025:bool)
        }
        n457 = global read "Results_plotter_Global.vi" "First Loop"() -> (w976:bool)
        n458 = while {
          shift-right: [w996] -> _
          shift-left: _ -> [w995]
          shift-right: [w993] -> _
          shift-left: _ -> [w994]
          tunnel: [w992] -> w971
          tunnel: [w991] -> w970
          stop <- FALSE continue-if-true
          n459 = local read "Filter Bins 1"() -> (w993:i32[])
          n460 = local read "Filter Bins 2"() -> (w996:i32[])
          n461 = Equal?(x=w993, y=w994) -> (x = y?=w991:bool)
          n462 = Equal?(x=w996, y=w995) -> (x = y?=w992:bool)
        }
        n463 = Not(x=w964) -> (.not. x?=w968:bool)
        n464 = property on="Resolution" class="DigNum (strict)"("Visible"=w964) -> ()  [unwired: 2 in, 2 out]
        n465 = property on="Bkgnd Value" class="DigNum (strict)"("Visible"=w964) -> ()  [unwired: 2 in, 2 out]
        n466 = property on="Intensity Graph" class="IntGraph (strict)"("Visible"=w964) -> ()  [unwired: 2 in, 2 out]
        n467 = property on="XY Plot" class="XYGraph (strict)"("Visible"=w968) -> ()  [unwired: 2 in, 2 out]
        n468 = Compound Arithmetic op=AND(w971, w970) -> (w969:bool)
        n469 = Compound Arithmetic op=AND(w967, w969, w972, w973, w978, w981, w982, w986, w985, w965, w980, w975, w974, invert w976) -> (w984:bool)
        n470 = Select(t="What to do next?", s=w984, f="Prepare for Plotting") -> (s? t:f=w983:string)
      }
      frame "Prepare for Plotting" {
        n471 = local read "Filter Array"() -> (w1042:u16[])
        n472 = local read "Multi Ordinate"() -> (w1037:i32[])
        n473 = Index Array(array=w1042, index=0 ("Index")) -> (element=w1039:u16)
        n474 = Equal To 0?(x=w1039) -> (x = 0?=w1040:bool)
        n475 = for {
          tunnel: w1037 -> [w1048] mode=indexing
          tunnel: [w1047] -> w1035 mode=indexing
          tunnel: w1036 -> [w1046]
          n476 = Index Array(array=w1046, index=w1048) -> (element=w1047:string)
        }
        n477 = case shown="False" w1040 {
          tunnel: w1039 -> [w1054 _]
          tunnel: w1036 -> [w1052 _]
          tunnel: [w1049 string[] []] -> w1034
          frame False {
            n478 = Decrement(x=w1054) -> (x-1=w1053:u16)
            n479 = local read "Filter Bins 1"() -> (w1056:i32[])
            n480 = property on="Filter bins 1" class="LstBox (strict)"() -> ("Item Names"=w1055:string[])  [unwired: 2 in, 2 out]
            n481 = Index Array(array=w1052, index=w1053) -> (element=w1050:string)
            n482 = for {
              tunnel: w1056 -> [w1059] mode=indexing
              tunnel: w1055 -> [w1058]
              tunnel: [w1057] -> w1051 mode=indexing
              n483 = Index Array(array=w1058, index=w1059) -> (element=w1057:string)
            }
            n484 = Build Array (concatenate)(w1050, w1051) -> (w1049:string[])
          }
          frame True {
          }
        }
        n485 = global write "Results_plotter_Global.vi" "Ordinate Strings"(w1035) -> ()
        n486 = global write "Results_plotter_Global.vi" "Filter 1 Strings"(w1034) -> ()
      }
      frame "Prepare Filter2 strings" {
        n487 = local read "Filter Array"() -> (w1067:u16[])
        n488 = Index Array(array=w1067, index=1 ("Index")) -> (element=w1064:u16)
        n489 = Equal To 0?(x=w1064) -> (x = 0?=w1065:bool)
        n490 = case shown="False" w1065 {
          tunnel: w1064 -> [w1076 _]
          tunnel: w1063 -> [w1074 _]
          tunnel: [w1071 string[] []] -> w1061
          frame False {
            n491 = Decrement(x=w1076) -> (x-1=w1075:u16)
            n492 = local read "Filter Bins 2"() -> (w1078:i32[])
            n493 = property on="Filter Bins 2" class="LstBox (strict)"() -> ("Item Names"=w1077:string[])  [unwired: 2 in, 2 out]
            n494 = Index Array(array=w1074, index=w1075) -> (element=w1072:string)
            n495 = for {
              tunnel: w1078 -> [w1081] mode=indexing
              tunnel: w1077 -> [w1080]
              tunnel: [w1079] -> w1073 mode=indexing
              n496 = Index Array(array=w1080, index=w1081) -> (element=w1079:string)
            }
            n497 = Build Array (concatenate)(w1072, w1073) -> (w1071:string[])
          }
          frame True {
          }
        }
        n498 = global write "Results_plotter_Global.vi" "Filter 2 Strings"(w1061) -> ()
      }
      frame "Plot Data" {
        n499 = stacked-sequence {
          seq-local: [w1088 _ _] -> [_ w1124 _]
          seq-local: [w1089 _ _] -> [_ w1123 _]
          tunnel: w1086 -> [_ w1133 _]
          tunnel: [_ TRUE _] -> w1085
          tunnel: [_ _ w1151] -> w1084
          tunnel: w1083 -> [w1090 _ _]
          frame #0 {
            n500 = global read "Results_plotter_Global.vi" "Ordinate Strings"() -> (w1088:string[])
            n501 = for {
              tunnel: w1088 -> [w1092] mode=indexing
              tunnel: w1090 -> [w1095]
              tunnel: [w1093] -> w1089 mode=indexing
              n502 = String Length(string=w1092) -> (length=w1091:i32)
              n503 = for {
                tunnel: w1092 -> [w1099]
                tunnel: w1095 -> [w1096] mode=indexing
                shift-right: [w1103] -> w1093
                shift-left: -1 -> [w1101]
                tunnel: w1091 -> [w1097]
                i -> [w1102]
                n504 = String Subset(string=w1096, length (rest)=w1097) -> (substring=w1098:string)  [unwired: 1 out]
                n505 = Equal?(x=w1098, y=w1099) -> (x = y?=w1100:bool)
                n506 = case shown="True" w1100 {
                  tunnel: [w1115 w1118] -> w1103
                  tunnel: w1102 -> [w1114 _]
                  tunnel: w1101 -> [w1113 w1118]
                  tunnel: w1097 -> [w1112 _]
                  tunnel: w1096 -> [w1111 _]
                  frame True {
                    n507 = String Subset(string=w1111, offset (0)=w1112) -> (substring=w1105:string)  [unwired: 1 out]
                    n508 = call <vilib>:"Trim Whitespace.vi"("string"=w1105) -> ("trimmed string"=w1104:string)  [unwired: 1 in]
                    n509 = Equal?(x=w1104, y="Err") -> (x = y?=w1107:bool)
                    n510 = Equal?(x=w1104, y="err") -> (x = y?=w1108:bool)
                    n511 = Or(x=w1107, y=w1108) -> (x .or. y?=w1106:bool)
                    n512 = case shown="True" w1106 {
                      tunnel: [w1116 w1117] -> w1115
                      tunnel: w1114 -> [w1116 _]
                      tunnel: w1113 -> [_ w1117]
                      frame True {
                      }
                      frame False {
                      }
                    }
                  }
                  frame False {
                  }
                }
              }
            }
          }
          frame #1 {
            n513 = global read "Results_plotter_Global.vi" "Filter 1 Strings"() -> (w1119:string[])
            n514 = global read "Results_plotter_Global.vi" "Filter 2 Strings"() -> (w1120:string[])
            n515 = local read "Accept Array"() -> (w1135:bool[][])
            n516 = local read "Multi Ordinate?"() -> (w1129:bool)
            n517 = Select(t=5, s=w1129, f=2 ("y")) -> (s? t:f=w1127:i32)
            n518 = global write "Results_plotter_Global.vi" "Ordinate"("Multi Ordinate") -> ()
            n519 = global write "Results_plotter_Global.vi" "Absisca"("Absisca") -> ()
            n520 = global write "Results_plotter_Global.vi" "Transpose"("Transpose") -> ()
            n521 = while {
              shift-right: [w1138] -> w1132
              shift-left: _ -> [w1139]
              tunnel: "color and symbol" -> [w1140]
              tunnel: w1127 -> [w1136]
              stop <- FALSE continue-if-true
              n522 = case shown="True" w1140 {
                tunnel: w1139 -> [w1147 w1149]
                tunnel: [w1146 w1149] -> w1138
                tunnel: w1136 -> [w1141 _]
                frame True {
                  n523 = Add(x=w1147, y=1) -> (x+y=w1144:i32)
                  n524 = local write "color and symbol"(FALSE ("color and symbol")) -> ()
                  n525 = Greater?(x=w1144, y=w1141) -> (0:w1145:bool)
                  n526 = Select(t=0, s=w1145, f=w1144) -> (s? t:f=w1146:i32)
                }
                frame False {
                }
              }
            }
            n527 = call "Plot_XY_data.vi"("Channel Values"=w1133, "Ordinate Strings"=w1124, "Swap color and symbol"=w1132, "Error Bar Chs"=w1123, "Accept Array"=w1135, "Filter 1 Strings"=w1119, "Filter 2 Strings"=w1120, "Ordinate"="Multi Ordinate", "Absisca"="Absisca", "Transpose"="Transpose") -> ("Accept Array Out"=→"Plotted Series":bool[][])  [unwired: 5 out]
          }
          frame #2 {
            n528 = Select(t="Intensity plot", s="Intensity Plot?", f="Add Legend and scales") -> (s? t:f=w1151:string)
            n529 = property on="Surface Area" class="DigNum (strict)"("Visible"="Intensity Plot?") -> ()  [unwired: 2 in, 2 out]
            n530 = property on="Surface Integral" class="DigNum (strict)"("Visible"="Intensity Plot?") -> ()  [unwired: 2 in, 2 out]
            n531 = property on="Surface Average" class="DigNum (strict)"("Visible"="Intensity Plot?") -> ()  [unwired: 2 in, 2 out]
            n532 = property on="X Ch Name" class="Ring (strict)"("Visible"="Intensity Plot?") -> ()  [unwired: 2 in, 2 out]
            n533 = property on="Y Ch Name" class="Ring (strict)"("Visible"="Intensity Plot?") -> ()  [unwired: 2 in, 2 out]
            n534 = property on="Z Ch Name" class="Ring (strict)"("Visible"="Intensity Plot?") -> ()  [unwired: 2 in, 2 out]
            n535 = property on="Point Size" class="Slide (strict)"("Visible"="Intensity Plot?") -> ()  [unwired: 2 in, 2 out]
            n536 = property on="No of Contours" class="DigNum (strict)"("Visible"="Intensity Plot?") -> ()  [unwired: 2 in, 2 out]
            n537 = property on="Slice mode" class="Enum (strict)"("Visible"="Intensity Plot?") -> ()  [unwired: 2 in, 2 out]
            n538 = property on="Plot Resolution" class="Bool (strict)"("Visible"="Intensity Plot?") -> ()  [unwired: 2 in, 2 out]
            n539 = property on="Update" class="Bool (strict)"("Visible"="Intensity Plot?") -> ()  [unwired: 2 in, 2 out]
          }
        }
      }
      frame "Add Legend and scales" {
        n540 = local read "Transpose"() -> (w1157:bool)
        n541 = global read "Results_plotter_Global.vi" "Plot Index values"() -> (w1160:dbl[][])
        n542 = global read "Results_plotter_Global.vi" "XY Graph Cluster"() -> (→"XY Plot":cluster{dbl[], dbl[]}[])
        n543 = Select(t=1 ("index (row)"), s=w1157, f=0 ("index (row)")) -> (s? t:f=w1154:i32)
        n544 = Index Array(array=w1160, index (row)=w1154) -> (element=w1159:dbl[])  [unwired: 1 in]
        n545 = Array Max & Min(array=w1159) -> (max value=w1158:dbl)  [unwired: 3 out]
        n546 = global read "Results_plotter_Global.vi" "Point info"() -> (w1165:T13)
        n547 = global read "Results_plotter_Global.vi" "Legend"() -> (w1166:string[])
        n548 = Greater?(x=w1158, y=2680560000.0) -> (0:w1162:bool)
        n549 = case shown="False" w1162 {
          tunnel: [w1177 u8 7 ("X Scale.Format & Precision:Precision")] -> w1161
          tunnel: w1158 -> [w1183 _]
          frame False {
            n550 = Absolute Value(x=w1183) -> (abs(x)=w1176:dbl)
            n551 = In Range and Coerce(upper limit=100000.0 ("y"), x=w1176, lower limit=0.0001) -> (In Range?=w1180:bool)  [unwired: 1 out]
            n552 = Select(t=u8 0 ("f"), s=w1180, f=u8 1) -> (s? t:f=w1177:u8)
          }
          frame True {
          }
        }
        n553 = local write "Warning!"("") -> ()
        n554 = for {
          tunnel: w1166 -> [w1193] mode=indexing
          tunnel: w1165 -> [w1202] mode=indexing
          tunnel: [w1203] -> w1170
          i -> [w1203]
          n555 = String Length(string=w1193) -> (length=w1199:i32)
          n556 = Subtract(x=w1199, y=2) -> (x-y=w1197:i32)
          n557 = String Subset(string=w1193, length (rest)=w1197) -> (substring=w1191:string)  [unwired: 1 out]
          n558 = call "Abbreviate_string.vi"("Input String"=w1191, "Max String Length"=35) -> ("Output String"=w1190:string)
          n559 = Unbundle By Name(w1202) -> ("Point Style"=w1201:u8, "Fill/Pt. Color"=w1200:u32)
          n560 = call "Fast_string_Replace.vi"("Replace match with:"="_", "Input String"=w1190, "regular expression"=" ") -> ("Output String"=w1194:string)  [unwired: 1 in, 1 out]
          n561 = property on="XY Plot" class="XYGraph (strict)"("Active Plot"=w1203, "Plot.Plot Name"=w1194, "Plot.Point Style"=w1201, "Plot.Fill/Point Color"=w1200, "Plot.Plot Color"=w1200) -> ()  [unwired: 2 in, 2 out]
        }
        n562 = Increment(x=w1170) -> (x+1=w1169:i32)
        n563 = property on="XY Plot" class="XYGraph (strict)"("X Scale.Format & Precision:Format"=w1161) -> ()  [unwired: 2 in, 2 out]
        n564 = for {
          N: 10 -> [_]
          tunnel: w1169 -> [w1188]
          i -> [w1189]
          w1185 = u32 0
          n565 = Add(x=w1188, y=w1189) -> (x+y=w1187:i32)
          n566 = property on="XY Plot" class="XYGraph (strict)"("Active Plot"=w1187, "Plot.Plot Name"="" ("Write Attribute"), "Plot.Plot Color"=w1185, "Plot.Fill/Point Color"=w1185) -> ()  [unwired: 2 in, 2 out]
        }
      }
      frame "Add Axis names" {
        n567 = local read "Multi Ordinate"() -> (w1218:i32[])
        n568 = for {
          tunnel: w1218 -> [w1235] mode=indexing
          shift-right: [w1232] -> w1211
          shift-left: "" -> [w1231]
          tunnel: w1219 -> [w1234]
          tunnel: [w1227] -> w1210
          i -> [w1227]
          n569 = Index Array(array=w1234, index=w1235) -> (element=w1233:string)
          n570 = String Length(string=w1231) -> (length=w1230:i32)
          n571 = Less?(x=w1230, y=40) -> (x < y?=w1228:bool)
          n572 = case shown="True" w1228 {
            tunnel: w1233 -> [_ w1240]
            tunnel: [w1236 w1239] -> w1232
            tunnel: w1231 -> [w1236 w1237]
            frame False {
            }
            frame True {
              n573 = Concatenate Strings(w1237, w1240, "   ") -> (w1239:string)
            }
          }
        }
        n574 = Greater Than 0?(x=w1210) -> (x > 0?=w1208:bool)
        n575 = local read "Transpose"() -> (w1221:bool)
        n576 = local read "Absisca"() -> (w1222:u16)
        n577 = Index Array(array=w1219, index=w1222) -> (element=w1220:string)
        n578 = String Length(string=w1211) -> (length=w1214:i32)
        n579 = Empty String/Path?(string/path="Ordinate Name") -> (empty?=w1209:bool)
        n580 = Subtract(x=w1214, y=3) -> (x-y=w1212:i32)
        n581 = Compound Arithmetic op=AND(invert w1209, w1208) -> (w1207:bool)
        n582 = String Subset(string=w1211, length (rest)=w1212) -> (substring=w1206:string)  [unwired: 1 out]
        n583 = Select(t="Ordinate Name", s=w1207, f=w1206) -> (s? t:f=w1204:string)
        n584 = case shown="False" w1221 {
          tunnel: [w1241 w1244] -> w1217
          tunnel: w1204 -> [w1242 w1244]
          tunnel: [w1242 w1243] -> w1216
          tunnel: w1220 -> [w1241 w1243]
          frame False {
          }
          frame True {
          }
        }
        n585 = global write "Results_plotter_Global.vi" "X Axis Name"(w1217) -> ()
        n586 = global write "Results_plotter_Global.vi" "Y Axis Name"(w1216) -> ()
        n587 = global write "Results_plotter_Global.vi" "Value plotted Name"(w1204) -> ()
        n588 = property on="XY Plot" class="XYGraph (strict)"("X Scale.Name Label.Text"=w1217, "Y Scale.Name Label.Text"=w1216) -> ()  [unwired: 2 in, 2 out]
      }
      frame "Intensity plot" {
        # "Max"
        # "Min"
        n589 = global read "Results_plotter_Global.vi" "XY Graph Cluster"() -> (w1245:cluster{dbl[], dbl[]}[])
        n590 = local read "Tolerances"() -> (w1250:dbl[])
        n591 = local read "Absisca"() -> (w1249:u16)
        n592 = local read "Transpose"() -> (w1246:bool)
        n593 = stacked-sequence {
          seq-local: [w1263 _ _ _ _ _ _ _ _ _ _ _ _ _] -> [_ _ _ w1328 w1335 _ w1362 _ _ _ _ _ _ _]
          seq-local: [_ w1279 _ _ _ _ _ _ _ _ _ _ _ _] -> [_ _ _ _ w1334 _ w1361 _ _ _ _ _ _ _]
          seq-local: [_ _ w1311 _ _ _ _ _ _ _ _ _ _ _] -> [_ _ _ _ _ _ w1370 _ _ _ _ _ _ _]
          seq-local: [_ _ _ _ _ _ w1372 _ _ _ _ _ _ _] -> [_ _ _ _ _ _ _ _ _ w1405 _ _ _ _]
          seq-local: [_ _ _ _ _ _ w1371 _ _ _ _ _ _ _] -> [_ _ _ _ _ _ _ _ _ w1406 _ _ _ _]
          seq-local: [_ w1275 _ _ _ _ _ _ _ _ _ _ _ _] -> [_ _ _ _ _ _ _ _ _ _ w1470 _ _ _]
          seq-local: [_ _ _ w1326 _ _ _ _ _ _ _ _ _ _] -> [_ _ _ _ w1333 _ w1366 _ _ _ _ _ _ _]
          seq-local: [_ _ _ _ _ _ _ _ _ _ _ _ w1496 _] -> [_ _ _ _ _ _ _ _ _ _ _ _ _ w1546]
          seq-local: [_ _ _ _ _ _ _ _ _ _ _ _ w1495 _] -> [_ _ _ _ _ _ _ _ _ _ _ _ _ w1547]
          seq-local: [_ _ _ w1325 _ _ _ _ _ _ _ _ _ _] -> [_ _ _ _ _ w1348 _ _ _ _ _ _ _ _]
          seq-local: [_ _ _ _ _ _ _ _ _ _ _ _ w1493 _] -> [_ _ _ _ _ _ _ _ _ _ _ _ _ w1539]
          seq-local: [_ _ _ _ _ _ w1354 _ _ _ _ _ _ _] -> [_ _ _ _ _ _ _ w1383 _ _ _ _ _ _]
          tunnel: [_ _ _ TRUE _ _ _ _ _ _ _ _ _ _] -> w1256
          tunnel: [_ _ _ _ _ _ _ _ _ _ _ _ _ "Analyse Plot Space"] -> w1255
          tunnel: w1253 -> [w1260 _ _ _ _ _ _ _ _ _ _ _ _ _]
          tunnel: w1254 -> [w1261 _ w1312 _ _ _ _ _ _ _ w1451 _ _ _]
          tunnel: [w1261 _ _ _ _ _ _ _ _ _ _ _ _ _] -> w1252
          tunnel: [w1260 _ _ _ _ _ _ _ _ _ _ _ _ _] -> w1251
          tunnel: w1250 -> [w1265 _ _ _ _ _ _ _ _ _ _ _ _ _]
          tunnel: w1245 -> [w1264 _ _ w1330 _ _ _ _ _ _ _ _ _ _]
          tunnel: w1249 -> [w1262 _ _ _ _ _ _ _ _ _ w1467 _ _ _]
          tunnel: w1246 -> [w1259 _ _ w1327 _ _ w1374 _ _ _ w1465 _ _ _]
          tunnel: [_ w1280 _ _ _ _ _ _ _ _ _ _ _ _] -> w1248
          tunnel: w1247 -> [_ w1280 _ _ _ _ _ _ _ _ w1452 _ _ _]
          frame #0 {
            n594 = Not(x=w1259) -> (.not. x?=w1258:bool)
            n595 = for {
              tunnel: w1264 -> [w1274] mode=indexing
              tunnel: w1258 -> [w1271]
              shift-right: [w1269] -> w1266
              shift-left: dbl[] [] -> [w1270]
              n596 = Unbundle(w1274) -> (w1273:dbl[], w1272:dbl[])
              n597 = Select(t=w1273, s=w1271, f=w1272) -> (s? t:f=w1268:dbl[])
              n598 = Build Array (concatenate)(w1270, w1268) -> (w1269:dbl[])
            }
            n599 = Index Array(array=w1265, index=w1262) -> (element=w1257:dbl)
            n600 = call "Numeric_bins.vi"("Values"=w1266, "Tolerance"=w1257) -> ("Bin Centres"=w1263:dbl[])  [unwired: 2 out]
          }
          frame #1 {
            n601 = local read "Filter Bins 2"() -> (w1281:i32[])
            n602 = local read "Filter Bins 1"() -> (w1283:i32[])
            n603 = Array Size(array=w1281) -> (size(s)=w1285:i32)
            n604 = Array Size(array=w1283) -> (size(s)=w1286:i32)
            n605 = Greater?(x=w1286, y=w1285) -> (0:w1284:bool)
            n606 = case shown="False" w1284 {
              tunnel: w1283 -> [_ w1308]
              tunnel: [w1304 w1308] -> w1282
              tunnel: [w1305 w1307] -> w1277
              tunnel: w1281 -> [w1304 _]
              tunnel: [1 0] -> w1275
              frame False {
                n607 = property on="Filter Bins 2" class="LstBox (strict)"() -> ("Item Names"=w1305:string[])  [unwired: 2 in, 2 out]
              }
              frame True {
                n608 = property on="Filter Bins 1" class="LstBox (strict)"() -> ("Item Names"=w1307:string[])  [unwired: 2 in, 2 out]
              }
            }
            n609 = Array Size(array=w1277) -> (size(s)=w1276:i32)
            n610 = for {
              tunnel: w1282 -> [w1291] mode=indexing
              tunnel: w1277 -> [w1297]
              shift-right: [w1294] -> w1279
              shift-left: dbl[] [] -> [w1295]
              tunnel: w1276 -> [w1290]
              n611 = Index Array(array=w1297, index=w1291) -> (element=w1293:string)
              n612 = Less?(x=w1291, y=w1290) -> (x < y?=w1289:bool)
              n613 = Match Pattern(string=w1293, regular expression=" (0)") -> (offset past match=w1292:i32)  [unwired: 4 out]
              n614 = Less Than 0?(x=w1292) -> (x < 0?=w1288:bool)
              n615 = And(x=w1288, y=w1289) -> (x .and. y?=w1287:bool)
              n616 = case shown="True" w1287 {
                tunnel: w1295 -> [w1298 w1302]
                tunnel: [w1298 w1301] -> w1294
                tunnel: w1293 -> [_ w1300]
                frame False {
                }
                frame True {
                  n617 = Fract/Exp String To Number(string=w1300) -> (number=w1299:dbl)  [unwired: 4 out]
                  n618 = Build Array (concatenate)(w1302, w1299) -> (w1301:dbl[])
                }
              }
            }
          }
          frame #2 {
            n619 = local read "Template"() -> (w1310:path)
            n620 = call "Valid_Path.vi"("Filename"=w1310) -> ("Valid Path?"=w1309:bool)
            n621 = case shown="True" w1309 {
              tunnel: w1310 -> [_ w1322]
              tunnel: w1312 -> [_ w1321]
              tunnel: [nan w1318] -> w1311
              frame False {
              }
              frame True {
                n622 = local read "Multi Ordinate"() -> (w1317:i32[])
                n623 = call "Read_Write_Template.vi"("Template File"=w1322, "Mode"=Global_mode."Read Global", "Channel names In"=w1321, "Data type"="Minimum Value") -> ("1D Info Out"=w1320:string[])  [unwired: 4 in, 7 out]
                n624 = Index Array(array=w1317, index=0 ("Index")) -> (element=w1316:i32)
                n625 = Index Array(array=w1320, index=w1316) -> (element=w1319:string)
                n626 = Fract/Exp String To Number(string=w1319, default (0 dbl)=nan) -> (number=w1318:dbl)  [unwired: 3 out]
              }
            }
          }
          frame #3 {
            n627 = call "Grid_Data.vi"("Transpose"=w1327, "XY Graph"=w1330, "Bin Centres"=w1328) -> ("No of Duplicates"=w1325:i32, "Grided data"=w1326:dbl[][])
          }
          frame #4 {
            n628 = for {
              tunnel: w1335 -> [w1340]
              tunnel: w1334 -> [w1339] mode=indexing
              tunnel: w1333 -> [w1338] mode=indexing
              shift-right: [w1336] -> w1331
              shift-left: dbl[][] [] -> [w1337]
              n629 = for {
                tunnel: w1340 -> [w1346] mode=indexing
                tunnel: w1339 -> [w1341]
                tunnel: w1338 -> [w1345] mode=indexing
                shift-right: [w1342] -> w1336
                shift-left: w1337 -> [w1344]
                n630 = Build Array(w1346, w1341, w1345) -> (w1343:dbl[])
                n631 = Build Array (concatenate)(w1344, w1343) -> (w1342:dbl[][])
              }
            }
            n632 = global write "Results_plotter_Global.vi" "Intensity Plot data in rows"(w1331) -> ()
          }
          frame #5 {
            n633 = case shown="1, Default" w1348 {
              tunnel: w1348 -> [_ w1352]
              tunnel: ["" w1350] -> w1347
              frame 0 {
              }
              frame 1, Default {
                n634 = Format Into String(format string="%d duplicate points have been averaged together!", w1352) -> (resulting string=w1350:string)  [unwired: 2 in, 1 out]
              }
            }
            "Warning!" <- w1347
          }
          frame #6 {
            n635 = call "Insert_extra_rows_and_col.vi"("Row Values In"=w1361, "Additional Row Values"="Additional X Values", "Column Values In"=w1362, "Data In"=w1366, "Additional Column Values"="Additional Y Values") -> ("Row Values Out"=w1363:dbl[], "Column Values Out"=w1364:dbl[], "Data Out"=w1365:dbl[][])  [unwired: 2 out]
            n636 = Select(t="Resolution", s="Plot Resolution", f=0.0) -> (s? t:f=w1356:dbl)
            n637 = call "2D_interpolation.vi"("X Axis Current"=w1364, "Min Z Value In"=w1370, "Y axis Current"=w1363, "Bkgnd Value"="Bkgnd Value", "Plot In"=w1365, "Increment Value"=w1356, "Transpose"=w1374, "Point Size"="Point Size") -> ("min Z value"=w1372:dbl, "max Z value"=w1371:dbl, "Increment Value Out"=w1360:dbl, "Axis info"=w1354:T14, "Plot Out"=→"Intensity Graph":dbl[][], "Raw Interpolation"=w1353:dbl[][])  [unwired: 2 out]
            n638 = global write "Results_plotter_Global.vi" "Raw Interpolation"(w1353) -> ()
            n639 = local write "Resolution"(w1360) -> ()
          }
          frame #7 {
            n640 = Unbundle By Name(w1383) -> ("X Max"=w1382:dbl, "Y Max"=w1381:dbl, "X Scale"=w1380:cluster{"Xo":dbl, "delta X":dbl}, "Y Scale"=w1379:cluster{"Xo":dbl, "delta X":dbl}, "X Values"=w1378:dbl[], "Y Values"=w1377:dbl[], "Z Max"=w1376:dbl, "Z Min"=w1375:dbl)
            n641 = global write "Results_plotter_Global.vi" "X Scale"(w1380) -> ()
            n642 = global write "Results_plotter_Global.vi" "X Values"(w1378) -> ()
            n643 = global write "Results_plotter_Global.vi" "Y Values"(w1377) -> ()
            n644 = global write "Results_plotter_Global.vi" "Y Scale"(w1379) -> ()
            n645 = global write "Results_plotter_Global.vi" "Y Max"(w1381) -> ()
            n646 = global write "Results_plotter_Global.vi" "Z Max"(w1376) -> ()
            n647 = global write "Results_plotter_Global.vi" "Z Min"(w1375) -> ()
            n648 = global write "Results_plotter_Global.vi" "X Max"(w1382) -> ()
          }
          frame #8 {
            n649 = global read "Results_plotter_Global.vi" "X Scale"() -> (w1391:cluster{"Xo":dbl, "delta X":dbl})
            n650 = global read "Results_plotter_Global.vi" "Y Scale"() -> (w1387:cluster{"Xo":dbl, "delta X":dbl})
            n651 = global read "Results_plotter_Global.vi" "Y Max"() -> (w1388:dbl)
            n652 = global read "Results_plotter_Global.vi" "X Max"() -> (w1389:dbl)
            n653 = Unbundle By Name(w1387) -> ("Xo"=w1386:dbl)
            n654 = Unbundle By Name(w1391) -> ("Xo"=w1390:dbl)
            n655 = Subtract(x=w1388, y=w1386) -> (x-y=w1392:dbl)
            n656 = Subtract(x=w1389, y=w1390) -> (x-y=w1401:dbl)
            n657 = Greater?(x=w1401, y=5.0) -> (0:w1399:bool)
            n658 = Greater?(x=w1392, y=5.0) -> (0:w1394:bool)
            n659 = Select(t=u8 0 ("Write Attribute"), s=w1399, f=u8 3) -> (s? t:f=w1385:u8)
            n660 = Select(t=u8 0 ("Write Attribute"), s=w1394, f=u8 3) -> (s? t:f=w1384:u8)
            n661 = property on="Intensity Graph" class="IntGraph (strict)"("X Scale.Offset and Multiplier"=w1391, "X Scale.Range:Maximum"=w1389, "Y Scale.Offset and Multiplier"=w1387, "Y Scale.Range:Maximum"=w1388, "X Scale.Format & Precision:Precision"=w1385, "Y Scale.Format & Precision:Precision"=w1384) -> ()  [unwired: 2 in, 2 out]
          }
          frame #9 {
            n662 = Greater Than 0?(x=w1406) -> (x > 0?=w1403:bool)
            n663 = Less Than 0?(x=w1405) -> (x < 0?=w1404:bool)
            n664 = And(x=w1403, y=w1404) -> (x .and. y?=w1402:bool)
            n665 = case shown="False" w1402 {
              tunnel: w1406 -> [w1435 w1449]
              tunnel: [w1443 w1447] -> w1408
              tunnel: w1405 -> [w1431 w1444]
              frame True {
                (unwired) u32 3743
                (unwired) u32 16721152
                n666 = Absolute Value(x=w1431) -> (abs(x)=w1430:dbl)
                n667 = Absolute Value(x=w1435) -> (abs(x)=w1437:dbl)
                n668 = Absolute Value(x=w1431) -> (abs(x)=w1438:dbl)
                n669 = Max & Min(x=w1437, y=w1438) -> (max(x,y)=w1433:dbl)  [unwired: 1 out]
                n670 = Divide(x=w1430, y=w1433) -> (x/y=w1424:dbl)
                n671 = Subtract(x=1.0, y=w1424) -> (x-y=w1423:dbl)
                n672 = Multiply(x=w1423, y=u32 255) -> (x*y=w1429:dbl)
                n673 = To Unsigned Long Integer(number=w1429) -> (unsigned 32bit integer=w1413:u32)
                n674 = Multiply(x=w1413, y=u32 256) -> (x*y=w1415:u32)
                n675 = Multiply(x=w1413, y=u32 65536) -> (x*y=w1412:u32)
                n676 = Compound Arithmetic op=ADD(w1412, w1415, u32 255) -> (w1411:u32)
                n677 = Bundle("min Z value"=w1431, w1411) -> (w1440:cluster{"min Z value":dbl, u32})  [unwired: 1 out]
                n678 = Divide(x=w1435, y=w1433) -> (x/y=w1428:dbl)
                n679 = Bundle("max Z value"=0.0, u32 16777215) -> (w1439:cluster{"max Z value":dbl, u32})  [unwired: 1 out]
                n680 = Subtract(x=1.0, y=w1428) -> (x-y=w1426:dbl)
                n681 = Multiply(x=w1426, y=u32 255) -> (x*y=w1422:dbl)
                n682 = To Unsigned Long Integer(number=w1422) -> (unsigned 32bit integer=w1409:u32)
                n683 = Multiply(x=w1409, y=u32 256) -> (x*y=w1419:u32)
                n684 = Compound Arithmetic op=ADD(w1409, w1419, u32 16711680) -> (w1410:u32)
                n685 = Bundle("max Z value"=w1435, w1410) -> (w1442:cluster{"max Z value":dbl, u32})  [unwired: 1 out]
                n686 = Build Array(w1442, w1440) -> (w1441:cluster{"min Z value":dbl, u32}[])
                n687 = Build Array (concatenate)(w1441, w1439) -> (w1443:cluster{"max Z value":dbl, u32}[])
              }
              frame False {
                n688 = Bundle("max Z value"=w1449, u32 16721152) -> (w1446:cluster{"max Z value":dbl, u32})  [unwired: 1 out]
                n689 = Bundle("min Z value"=w1444, u32 3743) -> (w1445:cluster{"min Z value":dbl, u32})  [unwired: 1 out]
                n690 = Build Array(w1446, w1445) -> (w1447:cluster{"min Z value":dbl, u32}[])
              }
            }
            n691 = property on="Intensity Graph" class="IntGraph (strict)"("Ignore Array"=FALSE ("Write Attribute"), "Z Scale.Marker Values[]"=w1408) -> ()  [unwired: 2 in, 2 out]
          }
          frame #10 {
            n692 = local read "Filter Array"() -> (w1469:u16[])
            n693 = Index Array(array=w1469, index=w1470) -> (element=w1468:u16)
            n694 = Decrement(x=w1468) -> (x-1=w1466:u16)
            n695 = local read "Multi Ordinate"() -> (w1456:i32[])
            n696 = Index Array(array=w1452, index=w1466) -> (element=w1460:string)
            n697 = Index Array(array=w1452, index=w1467) -> (element=w1459:string)
            n698 = case shown="False" w1465 {
              tunnel: [w1472 w1474] -> w1458
              tunnel: w1460 -> [w1472 w1473]
              tunnel: w1459 -> [w1471 w1474]
              tunnel: [w1471 w1473] -> w1457
              frame False {
              }
              frame True {
              }
            }
            n699 = Index Array(array=w1456, index=0) -> (element=w1454:i32)
            n700 = Index Array(array=w1451, index=w1454) -> (element=w1453:string)
            n701 = global write "Results_plotter_Global.vi" "Value plotted Name"(w1453) -> ()
            n702 = property on="Intensity Graph" class="IntGraph (strict)"("X Scale.Name Label.Text"=w1457, "Y Scale.Name Label.Text"=w1458) -> ()  [unwired: 2 in, 2 out]
            n703 = global write "Results_plotter_Global.vi" "Y Axis Name"(w1457) -> ()
            n704 = global write "Results_plotter_Global.vi" "X Axis Name"(w1458) -> ()
            n705 = Format Into String(format string="Add %s values", w1460) -> (resulting string=→"First Add label":string)  [unwired: 2 in, 1 out]
            n706 = Format Into String(format string="Add %s values", w1459) -> (resulting string=→"2nd Add label":string)  [unwired: 2 in, 1 out]
          }
          frame #11 {
            n707 = property on="Intensity Graph" class="IntGraph (strict)"() -> ("Color Table"=w1476:u32[])  [unwired: 2 in, 2 out]
            n708 = Increment(x="No of Contours") -> (x+1=w1477:i32)
            n709 = Divide(x=255, y=w1477) -> (x/y=w1481:dbl)
            n710 = To Long Integer(number=w1481) -> (32bit integer=w1480:i32)
            n711 = for {
              tunnel: w1480 -> [w1489]
              tunnel: [w1486] -> w1475 mode=indexing
              tunnel: w1476 -> [w1485] mode=indexing
              tunnel: u32 0 -> [w1484]
              i -> [w1490]
              n712 = Increment(x=w1490) -> (x+1=w1487:i32)
              n713 = Quotient & Remainder(x=w1487, y=w1489) -> (x-y*floor(x/y)=w1488:i32)  [unwired: 1 out]
              n714 = case shown="0" w1488 {
                tunnel: [w1491 w1492] -> w1486
                tunnel: w1485 -> [_ w1492]
                tunnel: w1484 -> [w1491 _]
                frame 0 {
                }
                frame 1, Default {
                }
              }
            }
            n715 = property on="Intensity Graph" class="IntGraph (strict)"("Ignore Array"=TRUE ("Write Attribute"), "Color Table"=w1475) -> ()  [unwired: 2 in, 2 out]
          }
          frame #12 {
            n716 = global read "Results_plotter_Global.vi" "Raw Interpolation"() -> (w1494:dbl[][])
            n717 = Add Array Elements(numeric array=w1494) -> (sum=w1493:dbl)
            n718 = Array Size(array=w1494) -> (size(s)=w1504:i32[])
            n719 = Decrement(x=w1504) -> (x-1=w1502:i32[])
            n720 = Index Array(array=w1502, index=0) -> (element=w1503:i32)
            n721 = Index Array(array=w1502, index=1) -> (element=w1499:i32)
            n722 = for {
              N: w1503 -> [_]
              tunnel: w1494 -> [w1512]
              tunnel: w1499 -> [w1511]
              shift-right: [w1507] -> w1496
              shift-left: 0.0 -> [w1508]
              shift-right: [w1506] -> w1495
              shift-left: 0 -> [w1505]
              i -> [w1510]
              n723 = Increment(x=w1510) -> (x+1=w1509:i32)
              n724 = for {
                N: w1511 -> [_]
                tunnel: w1512 -> [w1521]
                tunnel: w1510 -> [w1526]
                tunnel: w1509 -> [w1524]
                shift-right: [w1517] -> w1507
                shift-left: w1508 -> [w1516]
                shift-right: [w1513] -> w1506
                shift-left: w1505 -> [w1514]
                i -> [w1525]
                n725 = Increment(x=w1525) -> (x+1=w1523:i32)
                n726 = Index Array(array=w1521, index (row)=w1526, index (col)=w1523) -> (element=w1522:dbl)
                n727 = Index Array(array=w1521, index (row)=w1524, index (col)=w1523) -> (element=w1519:dbl)
                n728 = Index Array(array=w1521, index (row)=w1526, index (col)=w1525) -> (element=w1527:dbl)
                n729 = Index Array(array=w1521, index (row)=w1524, index (col)=w1525) -> (element=w1520:dbl)
                n730 = Compound Arithmetic op=ADD(w1527, w1522, w1520, w1519) -> (w1515:dbl)
                n731 = Not A Number/Path/Refnum?(number/path/refnum=w1515) -> (NaN/Path/Refnum?=w1518:bool)
                n732 = case shown="False" w1518 {
                  tunnel: [w1531 w1535] -> w1517
                  tunnel: w1516 -> [w1533 w1535]
                  tunnel: w1515 -> [w1532 _]
                  tunnel: [w1530 w1534] -> w1513
                  tunnel: w1514 -> [w1529 w1534]
                  frame False {
                    n733 = Add(x=w1532, y=w1533) -> (x+y=w1531:dbl)
                    n734 = Add(x=1, y=w1529) -> (x+y=w1530:i32)
                  }
                  frame True {
                  }
                }
              }
            }
          }
          frame #13 {
            n735 = local read "Resolution"() -> (w1548:dbl)
            n736 = Divide(x=w1546, y=4.0) -> (x/y=w1544:dbl)
            n737 = Multiply(x=w1548, y=w1548) -> (x*y=w1540:dbl)
            n738 = Multiply(x=w1540, y=w1539) -> ()  [unwired: 1 out]
            n739 = Multiply(x=w1540, y=w1547) -> (x*y=w1541:dbl)
            "Surface Area" <- w1541
            n740 = Multiply(x=w1540, y=w1544) -> (x*y=w1537:dbl)
            "Surface Integral" <- w1537
            n741 = global write "Results_plotter_Global.vi" "Surface Area"(w1541) -> ()
            n742 = global write "Results_plotter_Global.vi" "Surface Integral"(w1537) -> ()
            n743 = Divide(x=16666667, y=w1537) -> (x/y=→"Uadvec":dbl)
            n744 = Divide(x=w1537, y=w1541) -> (x/y=→"Surface Average":dbl)
          }
        }
      }
      frame "Analyse Plot Space" {
        n745 = case shown="True" "Show Plot Space Analysis" {
          tunnel: w1553 -> [_ w1563]
          tunnel: w1550 -> [_ w1562]
          frame False {
          }
          frame True {
            w1559 = TRUE  # Summarise All
            n746 = global read "Results_plotter_Global.vi" "Plot Index values"() -> (w1557:dbl[][])
            n747 = Index Array(array=w1557, index (row)=2) -> (element=w1556:dbl[])  [unwired: 1 in]
            n748 = To Long Integer(number=w1556) -> (32bit integer=w1555:i32[])
            n749 = for {
              tunnel: w1555 -> [w1566] mode=indexing
              tunnel: w1563 -> [w1565]
              tunnel: [w1564] -> w1560 mode=indexing
              n750 = Index Array(array=w1565, index (row)=w1566) -> (element=w1564:string[])  [unwired: 1 in]
            }
            n751 = call "Summarise.vi"("Channel Names"=w1562, "Data"=w1560, "Summarise All"=w1559) -> ("Summary"=w1561:string[][])  [unwired: 2 in]
            n752 = call "Plot_Space_Analysis.vi"("Table"=w1561) -> ()
          }
        }
      }
      frame "Vector Plot" {
        n753 = flat-sequence {
          tunnel: w1571 -> [w1576]
          tunnel: w1569 -> [w1575]
          frame #0 {
            n754 = local read "Job Directory"() -> (w1574:path)
            n755 = Build Path(base path=w1574, name or relative path="Vectors") -> (appended path=w1573:path)
            n756 = local read "Template"() -> (w1577:path)
            n757 = call "Vector_Plotting.vi"("JobVectorDirectory"=w1573, "Data"=w1575, "Template Filename"=w1577, "Channel Names"=w1576) -> ()  [unwired: 1 in]
          }
          frame #1 {
            n758 = local write "Vector Plot?"(FALSE ("Vector Plot?")) -> ()
          }
        }
      }
      frame "Coloured Dot Plot" {
        n759 = flat-sequence {
          tunnel: w1583 -> [w1588]
          tunnel: w1581 -> [w1587]
          frame #0 {
            n760 = local read "Job Directory"() -> (w1586:path)
            n761 = Build Path(base path=w1586, name or relative path="Dot_Plot") -> (appended path=w1585:path)
            n762 = local read "Template"() -> (w1589:path)
            n763 = call "Coloured_Dot_Plotting.vi"("JobVectorDirectory"=w1585, "Data"=w1587, "Template Filename"=w1589, "Channel Names"=w1588) -> ()  [unwired: 1 in]
          }
          frame #1 {
            n764 = local write "Dot Plot?"(FALSE ("Vector Plot?")) -> ()
          }
        }
      }
      frame "What to do next?" {
        n765 = local read "Warning!"() -> (w1602:string)
        n766 = Empty String/Path?(string/path=w1602) -> (empty?=w1601:bool)
        n767 = Not(x=w1601) -> (.not. x?=w1600:bool)
        n768 = property on="Warning!" class="Str" props=["Visible", "Blinking", "Caption"]("Visible"=w1600, "Blinking"=w1600) -> ()  [unwired: 2 in, 3 out]
        n769 = case shown="False" "Add results file" {
          tunnel: [w1624 "More files options"] -> w1605
          tunnel: "Add results file" -> [_ _]
          tunnel: "Edit Template File" -> [w1615 _]
          frame False {
            n770 = Select(t="Edit template file", s=w1615, f="What to do next 2nd?") -> (s? t:f=w1613:string)
            n771 = Or(x="Save Plot data", y="Save Surface Fit") -> (x .or. y?=w1617:bool)
            n772 = Select(t="Save Plot Data", s=w1617, f=w1613) -> (s? t:f=w1620:string)
            n773 = Select(t="Create Plot summary", s="Save Plot as jpg", f=w1620) -> (s? t:f=w1611:string)
            n774 = Select(t="Save Data in Rows", s="Save Data in Rows", f=w1611) -> (s? t:f=w1624:string)
          }
          frame True {
            n775 = local write "Add results file"(FALSE) -> ()
          }
        }
        n776 = Select(t="End", s="stop", f=w1605) -> (s? t:f=w1596:string)
        n777 = Select(t="Vector Plot", s="Vector Plot?", f=w1596) -> (s? t:f=w1592:string)
        n778 = Select(t="Coloured Dot Plot", s="Dot Plot?", f=w1592) -> (s? t:f=w1591:string)
      }
      frame "What to do next 2nd?" {
        n779 = local read "Empty"() -> (w1648:bool)
        n780 = local read "Last used Template"() -> (w1636:path)
        n781 = local read "Template"() -> (w1628:path)
        n782 = Select(t="Empty Results file array", s=w1648, f="What to do next 3rd?") -> (s? t:f=w1631:string)
        n783 = global write "Results_plotter_Global.vi" "Template"(w1628) -> ()
        n784 = Not Equal?(x=w1636, y=w1628) -> (x != y?=w1635:bool)
        n785 = local read "Selected Row"() -> (w1627:i32)
        n786 = Select(t="What type of row averaging?", s="Save Averaged rows", f=w1631) -> (s? t:f=w1643:string)
        n787 = case shown="True" "Delete Plotted data from file" {
          tunnel: [w1678 "Full Res file manipulator" ("t")] -> w1641
          tunnel: w1643 -> [w1678 _]
          frame False {
          }
          frame True {
            n788 = local write "Plotted rows only?"(TRUE ("Save Plotted rows only?")) -> ()
            n789 = local write "Mode"(Plotter_Mode."Delete unwanted rows" ("Mode")) -> ()
          }
        }
        n790 = case shown="True" "Add /Edit metadata" {
          tunnel: [w1653 w1670] -> w1633
          tunnel: w1641 -> [w1654 w1671]
          tunnel: w1639 -> [_ w1669]
          tunnel: "Reload Files" -> [w1655 _]
          tunnel: [string[] [] ("New Chs Out") w1663] -> w1630
          tunnel: [string[][] [] w1662] -> w1629
          tunnel: w1627 -> [_ w1658]
          frame False {
            n791 = Select(t="Initialise", s=w1655, f=w1654) -> (s? t:f=w1653:string)
          }
          frame True {
            n792 = local read "Result files to read"() -> (w1664:path[])
            n793 = call "Edit_Channel_Panel.vi"("All Channel names"=w1669, "Result files to read"=w1664, "Selected Row"=w1658) -> ("New Values Out"=w1677:string[], "New Chs Out"=w1663:string[], "Cancel Out"=w1666:bool, "Edit Raw Data Header Info Out"=w1660:bool, "Plotted rows only?"=w1676:bool, "Selected Row?"=→"Selected Row?":bool, "Edit Raw data files?"=→"Edit Raw DF?":bool, "Raw data files in Orig Positions?"=→"Raw DF in Orig Pos?":bool, "Mode"=w1674:T4)  [unwired: 4 out]
            "Edit Raw Data Header Info" <- w1660
            n794 = Array Size(array=w1663) -> (size(s)=w1673:i32)
            n795 = Build Array(w1677) -> (w1662:string[][])
            n796 = local write "Add /Edit metadata"(FALSE ("Add /Edit metadata")) -> ()
            n797 = Greater Than 0?(x=w1673) -> (x > 0?=w1661:bool)
            n798 = local write "Plotted rows only?"(w1676) -> ()
            n799 = Or(x=w1660, y=w1661) -> (x .or. y?=w1659:bool)
            n800 = local write "Mode"(w1674) -> ()
            n801 = Compound Arithmetic op=AND(invert w1666, w1659) -> (w1665:bool)
            n802 = Select(t="Full Res file manipulator", s=w1665, f=w1671) -> (s? t:f=w1670:string)
          }
        }
        n803 = global write "Results_plotter_Global.vi" "New Chs In"(w1630) -> ()
        n804 = global write "Results_plotter_Global.vi" "New Values In"(w1629) -> ()
        n805 = Select(t="Initialise", s=w1635, f=w1633) -> (s? t:f=w1632:string)
      }
      frame "What to do next 3rd?" {
        n806 = local read "Show Results Space Analysis"() -> (w1693:bool)
        n807 = local read "Show Plot Space Analysis"() -> (w1692:bool)
        n808 = while {
          shift-right: [w1716] -> _
          shift-left: _ -> [w1715]
          shift-left: _ -> [w1714]
          shift-left: _ -> [w1713]
          tunnel: w1693 -> [w1716]
          shift-right: [w1721] -> _
          shift-left: _ -> [w1720]
          shift-left: _ -> [w1719]
          shift-left: _ -> [w1718]
          tunnel: w1692 -> [w1721]
          tunnel: [w1717] -> w1691
          tunnel: [w1712] -> w1690
          stop <- TRUE stop-if-true
          n809 = Compound Arithmetic op=AND(w1716, w1715, w1714, w1713) -> (w1712:bool)
          n810 = Compound Arithmetic op=AND(w1721, w1720, w1719, w1718) -> (w1717:bool)
        }
        n811 = Select(t="Run Calculation Routine", s="Calculate new metadata", f="Time to save setup?") -> (s? t:f=w1699:string)
        n812 = case shown="True" w1691 {
          frame False {
          }
          frame True {
            n813 = Open VI Reference(vi path="Plot_Space_Analysis.vi" ("VI path")) -> (vi reference=w1733:refnum<vi>, error out=w1732:errorcluster)  [unwired: 1 in, 4 out]
            n814 = property class="VI"(reference=w1733, error in=w1732) -> (reference out=w1731:refnum<vi>, error out=w1730:errorcluster, "Front Panel Window:Open"=w1728:bool)
            n815 = local write "Show Plot Space Analysis"(w1728) -> ()
            n816 = Close Reference(reference=w1731, error in (no error)=w1730) -> ()  [unwired: 1 out]
          }
        }
        n817 = case shown="True" w1690 {
          frame False {
          }
          frame True {
            n818 = Open VI Reference(vi path="Results_Space_Analysis.vi" ("VI path")) -> (vi reference=w1727:refnum<vi>, error out=w1726:errorcluster)  [unwired: 1 in, 4 out]
            n819 = property class="VI"(reference=w1727, error in=w1726) -> (reference out=w1725:refnum<vi>, error out=w1724:errorcluster, "Front Panel Window:Open"=w1722:bool)
            n820 = local write "Show Results Space Analysis"(w1722) -> ()
            n821 = Close Reference(reference=w1725, error in (no error)=w1724) -> ()  [unwired: 1 out]
          }
        }
        n822 = Select(t="Save Setup", s="Save Setup", f=w1699) -> (s? t:f=w1696:string)
        n823 = Select(t="Choose Setup file", s="Load Setup", f=w1696) -> (s? t:f=w1689:string)
        n824 = Or(x="Kill Point", y="Process Point") -> (x .or. y?=w1686:bool)
        n825 = Select(t="Process cursor point", s=w1686, f=w1689) -> (s? t:f=w1682:string)
        n826 = case shown="False" "Post Process Plotted Data" {
          tunnel: [w1707 "Full Res file manipulator" ("t")] -> w1683
          tunnel: w1682 -> [w1707 _]
          frame False {
          }
          frame True {
            n827 = local write "Plotted rows only?"(TRUE ("Plotted rows only?")) -> ()
            n828 = local write "Mode"(Plotter_Mode."Post Process Plotted Rows" ("Mode")) -> ()
          }
        }
      }
      frame "Time to save setup?" {
        n829 = stacked-sequence {
          seq-local: [w1743 _] -> [_ w1787]
          seq-local: [w1742 _] -> [_ w1786]
          tunnel: [w1751 _] -> w1736
          tunnel: w1735 -> [w1741 _]
          tunnel: [w1740 _] -> w1734
          frame #0 {
            n830 = while {
              shift-right: [w1773] -> _
              shift-left: _ -> [w1771]
              shift-right: [w1760] -> _
              shift-left: _ -> [w1768]
              tunnel: [w1760] -> w1750
              tunnel: [w1759] -> w1749
              shift-right: [w1761] -> _
              shift-left: _ -> [w1767]
              tunnel: [w1765] -> w1744
              tunnel: [w1762] -> w1745
              tunnel: [w1761] -> w1746
              tunnel: [w1758] -> w1742
              tunnel: w1741 -> [w1754]
              tunnel: [w1753] -> w1740
              stop <- FALSE continue-if-true
              n831 = Get Date/Time In Seconds() -> (seconds since 1Jan1904=w1769:timestamp)
              n832 = To Double Precision Float(number=w1769) -> (double precision float=w1772:dbl)
              n833 = local read "Show Plot Space Analysis"() -> (w1761:bool)
              n834 = Subtract(x=w1772, y=w1771) -> (x-y=w1775:dbl)
              n835 = local read "Show Results Space Analysis"() -> (w1760:bool)
              n836 = Greater?(x=w1775, y=600.0) -> (0:w1756:bool)
              n837 = Greater?(x=w1754, y=300) -> (0:w1752:bool)
              n838 = And(x=w1756, y=w1752) -> (x .and. y?=w1755:bool)
              n839 = case shown="False" w1755 {
                tunnel: [w1776 w1785] -> w1773
                tunnel: w1772 -> [w1777 w1785]
                tunnel: w1771 -> [w1778 _]
                tunnel: ["Check modification dates?" "Save Setup"] -> w1764
                tunnel: [TRUE w1782] -> w1753
                tunnel: w1752 -> [w1779 _]
                frame False {
                  n840 = Select(t=w1778, s=w1779, f=w1777) -> (s? t:f=w1776:dbl)
                }
                frame True {
                  n841 = global read "Trav_pos_global.vi" "Estimated Completion time"() -> (w1784:string)
                  n842 = Empty String/Path?(string/path=w1784) -> (empty?=w1782:bool)
                }
              }
              n843 = Not Equal?(x=w1761, y=w1767) -> (x != y?=w1762:bool)
              n844 = Not Equal?(x=w1760, y=w1768) -> (x != y?=w1759:bool)
              n845 = Compound Arithmetic op=AND(invert w1760, w1759) -> (w1758:bool)
              n846 = And(x=w1761, y=w1762) -> (x .and. y?=w1766:bool)
              n847 = Select(t="Analyse Plot Space", s=w1766, f=w1764) -> (s? t:f=w1765:string)
            }
            n848 = Compound Arithmetic op=AND(invert w1746, w1745) -> (w1743:bool)
            n849 = And(x=w1750, y=w1749) -> (x .and. y?=w1748:bool)
            n850 = Select(t="What is present?", s=w1748, f=w1744) -> (s? t:f=w1751:string)
          }
          frame #1 {
            n851 = case shown="True" w1786 {
              frame False {
              }
              frame True {
                n852 = Open VI Reference(vi path="Results_Space_Analysis.vi" ("VI path")) -> (vi reference=w1793:refnum<vi>, error out=w1792:errorcluster)  [unwired: 1 in, 4 out]
                n853 = property class="VI"(reference=w1793, error in=w1792, "Front Panel Window:Open"=FALSE) -> (reference out=w1791:refnum<vi>, error out=w1790:errorcluster)
                n854 = Close Reference(reference=w1791, error in (no error)=w1790) -> ()  [unwired: 1 out]
              }
            }
            n855 = case shown="True" w1787 {
              frame False {
              }
              frame True {
                n856 = Open VI Reference(vi path="Plot_Space_Analysis.vi" ("VI path")) -> (vi reference=w1799:refnum<vi>, error out=w1798:errorcluster)  [unwired: 1 in, 4 out]
                n857 = property class="VI"(reference=w1799, error in=w1798, "Front Panel Window:Open"=FALSE) -> (reference out=w1797:refnum<vi>, error out=w1796:errorcluster)
                n858 = Close Reference(reference=w1797, error in (no error)=w1796) -> ()  [unwired: 1 out]
              }
            }
          }
        }
      }
      frame "Check modification dates?" {
        n859 = while {
          shift-right: [w1819] -> _
          shift-left: _ -> [w1817]
          tunnel: [w1816] -> w1808
          stop <- FALSE continue-if-true
          n860 = Get Date/Time In Seconds() -> (seconds since 1Jan1904=w1814:timestamp)
          n861 = To Double Precision Float(number=w1814) -> (double precision float=w1818:dbl)
          n862 = Subtract(x=w1818, y=w1817) -> (x-y=w1822:dbl)
          n863 = Greater?(x=w1822, y=200.0) -> (0:w1820:bool)
          n864 = case shown="True" w1820 {
            tunnel: [w1824 w1827] -> w1819
            tunnel: w1818 -> [_ w1827]
            tunnel: w1817 -> [w1824 _]
            tunnel: [FALSE w1825] -> w1816
            frame False {
            }
            frame True {
              n865 = global read "Results_plotter_Global.vi" "First Loop"() -> (w1826:bool)
              n866 = Not(x=w1826) -> (.not. x?=w1825:bool)
            }
          }
        }
        n867 = Equal?(x="Tab Control", y=enum32{"Load ", "Plot ", "Save ", "Cursor"}."Cursor" ("Tab Control")) -> (x = y?=w1804:bool)
        n868 = global write "Results_plotter_Global.vi" "First Loop"(FALSE) -> ()
        n869 = Select(t="Read Cursor", s=w1804, f="Ordinate Selector Type") -> (s? t:f=w1802:string)
        n870 = Select(t="Files Modified?", s=w1808, f=w1802) -> (s? t:f=w1807:string)
      }
      frame "Files Modified?" {
        n871 = local read "nRows"() -> (w1831:i32)
        n872 = Less?(x=w1831, y=w1830) -> (x < y?=w1828:bool)
        n873 = case shown="True" w1828 {
          tunnel: [w1837 w1843] -> w1832
          tunnel: "Ordinate Selector Type" -> [w1837 w1838]
          frame False {
          }
          frame True {
            n874 = local read "Result files to read"() -> (w1842:path[])
            n875 = for {
              tunnel: w1842 -> [w1846] mode=indexing
              tunnel: [w1844] -> w1841 mode=indexing
              n876 = call "File_Modified_Since_Check.vi"("Pathname"=w1846, "Just Modified?"=TRUE) -> ("Modified?"=w1844:bool)
            }
            n877 = Or Array Elements(Boolean array=w1841) -> (logical OR=w1840:bool)
            n878 = Select(t="Initialise", s=w1840, f=w1838) -> (s? t:f=w1843:string)
          }
        }
      }
      frame "Read Cursor" {
        n879 = stacked-sequence {
          seq-local: [w1852 _] -> [_ w1887]
          tunnel: ["Ordinate Selector Type" _] -> w1850
          tunnel: [TRUE _] -> w1849
          tunnel: w1848 -> [_ w1886]
          tunnel: w1847 -> [_ w1885]
          frame #0 {
            n880 = property on="XY Plot" class="XYGraph (strict)"() -> ("Cursor.Cursor Position:Cursor X"=w1854:dbl, "Cursor.Cursor Position:Cursor Y"=w1853:dbl)  [unwired: 2 in, 2 out]
            n881 = local read "Transpose"() -> (w1867:bool)
            n882 = global read "Results_plotter_Global.vi" "Plot Index values"() -> (w1860:dbl[][])
            n883 = Index Array(array=w1860, index (row)=1) -> (element=w1858:dbl[])  [unwired: 1 in]
            n884 = Index Array(array=w1860, index (row)=2) -> (element=w1857:dbl[])  [unwired: 1 in]
            n885 = Index Array(array=w1860, index (row)=0) -> (element=w1859:dbl[])  [unwired: 1 in]
            n886 = case shown="True" w1867 {
              tunnel: [w1871 w1873] -> w1866
              tunnel: w1854 -> [w1871 w1872]
              tunnel: [w1870 w1872] -> w1865
              tunnel: w1853 -> [w1870 w1873]
              frame False {
              }
              frame True {
              }
            }
            n887 = for {
              tunnel: w1866 -> [w1882]
              tunnel: w1865 -> [w1881]
              tunnel: [w1876] -> w1864 mode=indexing
              tunnel: w1859 -> [w1875] mode=indexing
              tunnel: w1858 -> [w1874] mode=indexing
              n888 = Subtract(x=w1882, y=w1875) -> (x-y=w1880:dbl)
              n889 = Subtract(x=w1881, y=w1874) -> (x-y=w1879:dbl)
              n890 = Multiply(x=w1880, y=w1880) -> (x*y=w1877:dbl)
              n891 = Multiply(x=w1879, y=w1879) -> (x*y=w1878:dbl)
              n892 = Add(x=w1877, y=w1878) -> (x+y=w1876:dbl)
            }
            n893 = Array Max & Min(array=w1864) -> (min index (indices)=w1856:i32)  [unwired: 3 out]
            n894 = Index Array(array=w1857, index=w1856) -> (element=w1855:dbl)
            n895 = To Long Integer(number=w1855) -> (32bit integer=w1852:i32)
            "Cursor index" <- w1852
          }
          frame #1 {
            n896 = Index Array(array=w1886, index (row)=w1887) -> (element=w1884:string[])  [unwired: 1 in]
            n897 = for {
              tunnel: w1885 -> [w1895] mode=indexing
              tunnel: w1884 -> [w1888] mode=indexing
              tunnel: [w1894] -> w1883 mode=indexing
              n898 = while {
                shift-right: [w1907] -> _
                shift-left: w1888 -> [w1908]
                tunnel: [w1904] -> w1892
                tunnel: [w1903] -> w1890 mode=indexing
                i -> [w1904]
                stop <- w1905 continue-if-true
                n899 = Match Pattern(string=w1908, regular expression=":") -> (before substring=w1903:string, after substring=w1907:string, offset past match=w1906:i32)  [unwired: 2 out]
                n900 = Greater Than 0?(x=w1906) -> (x > 0?=w1905:bool)
              }
              n901 = Greater?(x=w1892, y=2) -> (0:w1891:bool)
              n902 = Reverse 1D Array(array=w1890) -> (reversed array=w1889:string[])
              n903 = case shown="True" w1891 {
                tunnel: w1895 -> [w1898 w1902]
                tunnel: [w1896 w1901] -> w1894
                tunnel: w1889 -> [_ w1900]
                tunnel: w1888 -> [w1897 w1899]
                frame False {
                  n904 = Build Array(w1898, w1897) -> (w1896:string[])
                }
                frame True {
                  n905 = Build Array (concatenate)(w1902, w1900, w1899) -> (w1901:string[])
                }
              }
            }
            "Table" <- w1883
          }
        }
      }
      frame "Process Cursor Point" {
        n906 = stacked-sequence {
          tunnel: [w1922] -> w1914
          tunnel: [TRUE] -> w1913
          tunnel: w1912 -> [_]
          tunnel: w1911 -> [_]
          tunnel: w1910 -> [w1923]
          frame #0 {
            n907 = local read "Kill Point"() -> (w1924:bool)
            n908 = global read "Results_plotter_Global.vi" "Row Reference"() -> (w1930:i32[][])
            n909 = local read "Cursor index"() -> (w1929:i32)
            n910 = Index Array(array=w1930, index (row)=w1929) -> (element=w1925:i32[])  [unwired: 1 in]
            n911 = local read "Result files to read"() -> (w1928:path[])
            n912 = Index Array(array=w1925, index #1=0 ("index"), index #2=1 ("index")) -> (element #1=w1927:i32, element #2=w1916:i32)
            "Selected Row" <- w1916
            n913 = Index Array(array=w1928, index=w1927) -> (element=w1921:path)
            n914 = call "GetRawDataFilePaths.vi"("Results file or Folder"=w1921) -> ("RawDataFilePaths"=w1920:string[])  [unwired: 9 in, 1 out]
            n915 = Index Array(array=w1920, index=w1916) -> (element=w1919:string)
            n916 = call "String_to_Pathname.vi"("Input String"=w1919) -> ("path"=w1918:path)
            n917 = case shown="True" w1924 {
              tunnel: w1921 -> [_ w1952]
              tunnel: w1916 -> [_ w1948]
              tunnel: w1923 -> [_ w1955]
              tunnel: ["What to do next?" ("t") w1954] -> w1922
              tunnel: w1918 -> [w1932 w1946]
              frame False {
                n918 = disable-structure shown="Enabled" {
                  disable-tunnel: w1932 -> [_ w1944]
                  frame Disabled {
                    n919 = local read "Table"() -> (w1943:string[][])
                    n920 = Index Array(array=w1943, index (col) #1=1 ("disabled index (col)"), index (col) #2=0 ("index (col)")) -> (element #1=w1936:string[], element #2=w1935:string[])  [unwired: 2 in]
                    n921 = Search 1D Array(1D array=w1935, element="Raw Data Filename") -> (index of element=w1939:i32)  [unwired: 1 in]
                    n922 = Index Array(array=w1936, index=w1939) -> (element=w1938:string)
                    n923 = call "String_to_Pathname.vi"("Input String"=w1938) -> ("path"=w1937:path)
                    n924 = call "Post_Process_Measurement.vi"("Raw data file"=w1937) -> ()  [unwired: 1 out]
                  }
                  frame Enabled {
                    n925 = call "Post_Process_Measurement.vi"("Raw data file"=w1944) -> ()  [unwired: 1 out]
                  }
                }
                n926 = local write "Process Point"(FALSE ("Kill Point")) -> ()
              }
              frame True {
                n927 = Strip Path(path=w1952) -> (name=w1947:string)  [unwired: 1 out]
                n928 = Strip Path(path=w1946) -> (name=w1945:string)  [unwired: 1 out]
                n929 = local read "nRows"() -> (w1957:i32)
                n930 = Format Into String(format string="Are you sure you want to remove the row in the results file \"%s\" generated from the raw data filename \"%s\"?", w1947, w1945) -> (resulting string=w1950:string)  [unwired: 2 in, 1 out]
                n931 = Less?(x=w1957, y=w1955) -> (x < y?=w1956:bool)
                n932 = Two Button Dialog(message=w1950) -> (T button?=w1949:bool)  [unwired: 2 out]
                n933 = case shown="True" w1956 {
                  tunnel: ["Create Selectors" "Initialise" ("t")] -> w1954
                  frame False {
                  }
                  frame True {
                  }
                }
                n934 = case shown="True" w1949 {
                  tunnel: w1952 -> [_ w1959]
                  tunnel: w1948 -> [_ w1958]
                  frame False {
                  }
                  frame True {
                    n935 = Build Array(w1958) -> (w1960:i32[])
                    n936 = call "Delete_unwanted_rows.vi"("Selected Rows"=w1960, "Filename"=w1959) -> ()  [unwired: 1 out]
                  }
                }
                n937 = local write "Kill Point"(FALSE ("Kill Point")) -> ()
              }
            }
          }
        }
      }
      frame "Edit template file" {
        n938 = stacked-sequence {
          frame #0 {
            n939 = local read "Template"() -> (w1969:path)
            n940 = call "Valid_Path.vi"("Filename"=w1969) -> ("Valid Path?"=w1968:bool)
            n941 = case shown="False" w1968 {
              tunnel: [T8."Edit Existing Template File" ("Mode") T8."Create New Template File" ("Mode")] -> w1972
              frame True {
              }
              frame False {
              }
            }
            n942 = local read "Results file"() -> (w1971:path)
            n943 = call "Edit_Template_File.vi"("Mode"=w1972, "Template Filename"=w1969, "Data Filename"=w1971) -> ("Template Filename Out"=w1970:path)  [unwired: 12 out]
            n944 = local write "Template"(w1970) -> ()
          }
          frame #1 {
            n945 = local read "Job Directory"() -> (w1975:path)
            n946 = Path To String(path=w1975) -> (string=w1978:string)
            n947 = call "Read_Write_Template.vi"("Mode"=Global_mode."Write Global to File", "Single Value In"=w1978, "Data type"="Log Folder Name" ("Variable name")) -> ()  [unwired: 5 in, 8 out]
            n948 = local write "Edit Template File"(FALSE ("Edit Template File")) -> ()
            n949 = Current VI's Path() -> (path=w1981:path)
            n950 = call "Open_Close_Front_Panel.ph.vi"("Front Panel Window:Open"=TRUE, "VI path"=w1981) -> ()  [unwired: 2 out]
          }
        }
      }
      frame "Save Plot Data" {
        n951 = global read "Results_plotter_Global.vi" "XY Graph Cluster"() -> (w1982:cluster{dbl[], dbl[]}[])
        n952 = local read "Tolerances"() -> (w1989:dbl[])
        n953 = local read "Absisca"() -> (w1988:u16)
        n954 = local read "Transpose"() -> (w1987:bool)
        n955 = local read "Multi Ordinate"() -> (w1986:i32[])
        n956 = global read "Results_plotter_Global.vi" "Precision"() -> (w1983:string[])
        n957 = stacked-sequence {
          seq-local: [w2000 _ _ _ _ _ _ _ _] -> [_ w2025 _ w2063 _ _ _ _ _]
          seq-local: [_ w2021 _ _ _ _ _ _ _] -> [_ _ _ _ _ _ _ w2185 _]
          seq-local: [_ _ _ _ _ w2115 _ _ _] -> [_ _ _ _ _ _ _ w2184 _]
          seq-local: [_ _ _ _ _ w2117 _ _ _] -> [_ _ _ _ _ _ w2153 _ _]
          seq-local: [_ _ _ w2061 _ _ _ _ _] -> [_ _ _ _ _ _ w2154 _ _]
          seq-local: [_ _ _ _ w2084 _ _ _ _] -> [_ _ _ _ _ w2110 _ _ _]
          seq-local: [w1997 _ _ _ _ _ _ _ _] -> [_ _ _ _ _ _ _ _ w2190]
          seq-local: [w1996 _ _ _ _ _ _ _ _] -> [_ w2013 _ _ _ _ _ _ _]
          seq-local: [_ _ w2042 _ _ _ _ _ _] -> [_ _ _ w2062 _ _ w2155 _ _]
          seq-local: [_ _ _ _ _ _ w2151 _ _] -> [_ _ _ _ _ _ _ w2182 _]
          tunnel: [_ _ _ _ _ _ _ _ TRUE] -> w1995
          tunnel: [_ _ _ _ _ _ _ _ w2188] -> w1994
          tunnel: w1992 -> [_ _ _ _ _ w2113 _ _ _]
          tunnel: w1993 -> [_ w2018 _ _ _ w2116 _ _ _]
          tunnel: [_ _ _ _ _ w2116 _ _ _] -> w1991
          tunnel: [_ _ _ _ _ w2113 _ _ _] -> w1990
          tunnel: w1989 -> [w2002 _ _ _ w2089 w2114 _ _ _]
          tunnel: w1982 -> [w2001 _ _ w2065 _ _ _ _ _]
          tunnel: w1988 -> [w1999 w2035 _ _ w2091 _ _ _ _]
          tunnel: w1987 -> [w1998 _ _ w2064 _ _ _ _ _]
          tunnel: w1986 -> [_ _ _ _ w2088 _ _ _ _]
          tunnel: [_ _ _ w2059 _ _ _ _ _] -> w1985
          tunnel: w1984 -> [_ _ w2045 w2059 _ _ _ _ _]
          tunnel: w1983 -> [_ _ _ w2058 _ w2109 _ _ _]
          frame #0 {
            n958 = local read "Save Surface Fit"() -> (w1997:bool)
            n959 = Not(x=w1998) -> (.not. x?=w2005:bool)
            n960 = for {
              tunnel: w2001 -> [w2012] mode=indexing
              tunnel: w2005 -> [w2009]
              shift-right: [w2007] -> w2003
              shift-left: dbl[] [] -> [w2008]
              n961 = Unbundle(w2012) -> (w2011:dbl[], w2010:dbl[])
              n962 = Select(t=w2011, s=w2009, f=w2010) -> (s? t:f=w2006:dbl[])
              n963 = Build Array (concatenate)(w2008, w2006) -> (w2007:dbl[])
            }
            n964 = Index Array(array=w2002, index=w1999) -> (element=w1996:dbl)
            n965 = call "Numeric_bins.vi"("Values"=w2003, "Tolerance"=w1996) -> ("Bin Centres"=w2000:dbl[])  [unwired: 2 out]
          }
          frame #1 {
            n966 = Index Array(array=w2018, index=w2035) -> (element=w2038:string)
            n967 = Match Pattern(string=w2038, regular expression=":") -> (before substring=w2037:string, after substring=w2036:string)  [unwired: 3 out]
            n968 = Concatenate Strings(w2037, " ", w2036, " =:" ("regular expression")) -> (w2020:string)
            n969 = Greater?(x=w2013, y=0.4) -> (0:w2033:bool)
            n970 = Greater?(x=w2013, y=0.09) -> (0:w2028:bool)
            n971 = call <vilib>:"Trim Whitespace.vi"("string"=w2020) -> ("trimmed string"=w2019:string)  [unwired: 1 in]
            n972 = Select(t=i16 0 ("precision (6)"), s=w2033, f=i16 2 ("precision (6)")) -> (s? t:f=w2029:i16)
            n973 = Select(t=w2029, s=w2028, f=i16 3) -> (s? t:f=w2026:i16)
            n974 = Number To Fractional String(number=w2025, precision (6)=w2026) -> (F-format string=w2024:string[])  [unwired: 2 out]
            n975 = for {
              tunnel: w2019 -> [w2041]
              tunnel: w2024 -> [w2039] mode=indexing
              tunnel: [w2040] -> w2023 mode=indexing
              n976 = Concatenate Strings(w2041, w2039) -> (w2040:string)
            }
            n977 = Build Array (concatenate)("Plot:Legend:" ("Input Element"), w2023, "End of:Plot Series:" ("Input Element")) -> (w2021:string[])
          }
          frame #2 {
            n978 = local read "Multi Ordinate?"() -> (w2044:bool)
            n979 = global read "Results_plotter_Global.vi" "Legend"() -> (w2043:string[])
            n980 = case shown="False" w2044 {
              tunnel: w2045 -> [w2049 _]
              tunnel: [w2046 w2057] -> w2042
              tunnel: w2043 -> [w2048 w2057]
              frame False {
                n981 = local read "Multi Ordinate"() -> (w2052:i32[])
                n982 = Index Array(array=w2052, index=0 ("Index")) -> (element=w2050:i32)
                n983 = Index Array(array=w2049, index=w2050) -> (element=w2047:string)
                n984 = for {
                  tunnel: w2048 -> [w2056] mode=indexing
                  tunnel: w2047 -> [w2055]
                  tunnel: [w2053] -> w2046 mode=indexing
                  n985 = Format Into String(format string="; %s", initial string=w2055, w2056) -> (resulting string=w2053:string)  [unwired: 1 in, 1 out]
                }
              }
              frame True {
              }
            }
          }
          frame #3 {
            n986 = call "Grid_Data.vi"("Transpose"=w2064, "XY Graph"=w2065, "Bin Centres"=w2063) -> ("Grided data"=w2060:dbl[][])  [unwired: 1 out]
            n987 = for {
              tunnel: w2062 -> [w2072] mode=indexing
              tunnel: [w2074] -> w2061 mode=indexing
              tunnel: w2060 -> [w2073] mode=indexing
              tunnel: w2059 -> [w2068]
              tunnel: w2058 -> [w2067]
              n988 = Match Pattern(string=w2072, regular expression=";") -> (before substring=w2069:string)  [unwired: 4 out]
              n989 = Search 1D Array(1D array=w2068, element=w2069) -> (index of element=w2070:i32)  [unwired: 1 out]
              n990 = Index Array(array=w2067, index=w2070) -> (element=w2066:string)
              n991 = for {
                tunnel: w2066 -> [w2079]
                tunnel: [w2078] -> w2075 mode=indexing
                tunnel: w2073 -> [w2076] mode=indexing
                n992 = Not A Number/Path/Refnum?(number/path/refnum=w2076) -> (NaN/Path/Refnum?=w2077:bool)
                n993 = case shown="True" w2077 {
                  tunnel: w2079 -> [w2082 _]
                  tunnel: [w2081 ""] -> w2078
                  tunnel: w2076 -> [w2080 _]
                  frame False {
                    n994 = call "Number_2_string.vi"("precision"=w2082, "number"=w2080) -> ("String"=w2081:string)
                  }
                  frame True {
                  }
                }
              }
              n995 = Build Array (concatenate)(w2072, w2075) -> (w2074:string[])
            }
          }
          frame #4 {
            n996 = Index Array(array=w2088, index=0 ("Index")) -> (element=w2086:i32)
            n997 = global read "Results_plotter_Global.vi" "Summarise"() -> (w2085:string[])
            n998 = for {
              shift-right: [w2098] -> w2084
              shift-left: i32[] [] -> [w2099]
              tunnel: w2091 -> [w2104]
              tunnel: w2086 -> [w2103]
              tunnel: w2089 -> [w2096] mode=indexing
              tunnel: w2085 -> [w2094] mode=indexing
              i -> [w2097]
              n999 = Equal?(x=w2103, y=w2097) -> (x = y?=w2102:bool)
              n1000 = Not A Number/Path/Refnum?(number/path/refnum=w2096) -> (NaN/Path/Refnum?=w2095:bool)
              n1001 = Equal?(x=w2104, y=w2097) -> (x = y?=w2101:bool)
              n1002 = Equal?(x="FALSE", y=w2094) -> (x = y?=w2092:bool)
              n1003 = Compound Arithmetic op=OR(w2101, w2102, w2095, w2092) -> (w2100:bool)
              n1004 = case shown="False" w2100 {
                tunnel: w2099 -> [w2107 w2108]
                tunnel: [w2106 w2108] -> w2098
                tunnel: w2097 -> [w2105 _]
                frame False {
                  n1005 = Build Array (concatenate)(w2107, w2105) -> (w2106:i32[])
                }
                frame True {
                }
              }
            }
          }
          frame #5 {
            n1006 = local read "Plotted Series"() -> (w2112:bool[][])
            n1007 = for {
              tunnel: w2114 -> [w2128]
              tunnel: [w2127] -> w2117 mode=indexing
              tunnel: w2110 -> [w2126]
              tunnel: w2113 -> [w2125]
              tunnel: w2112 -> [w2124] mode=indexing
              tunnel: i32[] [] -> [w2122]
              tunnel: w2109 -> [w2121]
              n1008 = for {
                shift-right: [w2130] -> w2123
                shift-left: w2122 -> [w2131]
                tunnel: w2124 -> [w2129] mode=indexing
                i -> [w2132]
                n1009 = case shown="True" w2129 {
                  tunnel: w2132 -> [_ w2136]
                  tunnel: w2131 -> [w2133 w2135]
                  tunnel: [w2133 w2134] -> w2130
                  frame False {
                  }
                  frame True {
                    n1010 = Build Array (concatenate)(w2135, w2136) -> (w2134:i32[])
                  }
                }
              }
              n1011 = for {
                tunnel: w2128 -> [w2144]
                tunnel: [w2145] -> w2127 mode=indexing
                tunnel: w2126 -> [w2139] mode=indexing
                tunnel: w2125 -> [w2142]
                tunnel: w2123 -> [w2141]
                tunnel: w2121 -> [w2138]
                n1012 = for {
                  tunnel: w2141 -> [w2150] mode=indexing
                  tunnel: [w2149] -> w2146 mode=indexing
                  tunnel: w2139 -> [w2148]
                  tunnel: w2142 -> [w2147]
                  n1013 = Index Array(array=w2147, index (row)=w2150, index (col)=w2148) -> (element=w2149:string)
                }
                n1014 = Index Array(array=w2138, index=w2139) -> (element=w2140:string)
                n1015 = Index Array(array=w2144, index=w2139) -> (element=w2143:dbl)
                n1016 = call "Value_Occurence_Analysis.vi"("Average Numeric Values?"=FALSE, "Tolerance"=w2143, "Precision (3)"=w2140, "String Array"=w2146) -> ("Output String"=w2145:string)  [unwired: 2 out]
              }
            }
            n1017 = for {
              tunnel: w2110 -> [w2120] mode=indexing
              tunnel: w2116 -> [w2119]
              tunnel: [w2118] -> w2115 mode=indexing
              n1018 = Index Array(array=w2119, index=w2120) -> (element=w2118:string)
            }
          }
          frame #6 {
            n1019 = for {
              shift-right: [w2168] -> w2151
              shift-left: string[][] [] -> [w2169]
              shift-right: [w2164] -> _
              shift-left: _ -> [w2165]
              tunnel: w2155 -> [w2166] mode=indexing
              tunnel: w2154 -> [w2158] mode=indexing
              tunnel: w2153 -> [w2157] mode=indexing
              i -> [w2163]
              n1020 = Greater Than 0?(x=w2163) -> (x > 0?=w2162:bool)
              n1021 = Match Pattern(string=w2166, regular expression="; ") -> (before substring=w2164:string)  [unwired: 4 out]
              n1022 = Equal?(x=w2165, y=w2164) -> (x = y?=w2161:bool)
              n1023 = Build Array (concatenate)(w2158, "", w2157) -> (w2156:string[])
              n1024 = Compound Arithmetic op=AND(w2162, invert w2161) -> (w2160:bool)
              n1025 = case shown="True" w2160 {
                tunnel: w2169 -> [w2173 w2176]
                tunnel: [w2172 w2175] -> w2168
                tunnel: w2156 -> [w2171 w2174]
                frame True {
                  n1026 = Build Array (concatenate)(w2173, string[] [] ("array"), w2171) -> (w2172:string[][])
                }
                frame False {
                  n1027 = Build Array (concatenate)(w2176, w2174) -> (w2175:string[][])
                }
              }
            }
          }
          frame #7 {
            w2181 = TRUE  # Simple Save?
            n1028 = Build Array (concatenate)(w2185, w2184) -> (w2183:string[])
            n1029 = local read "Header"() -> (w2178:string)
            n1030 = call "Write_output_file.vi"("Output filename"="Output Filename", "Header"=w2178, "Channel Names"=w2183, "Data"=w2182, "Simple Save?"=w2181, "Summarise mode"=T9."No data summary") -> ("Output filename Out"=w2179:path)  [unwired: 6 in, 3 out]
            n1031 = local write "Output Filename"(w2179) -> ()
          }
          frame #8 {
            n1032 = local write "Save Plot data"(FALSE ("Save Plot data")) -> ()
            n1033 = local write "Header"("") -> ()
            n1034 = Select(t="Save Surface Fit data", s=w2190, f="Create Selectors") -> (s? t:f=w2188:string)
          }
        }
      }
      frame "What type of row averaging?" {
        n1035 = Two Button Dialog(message="Do you want to Combine rows with identical positions together?", 1:"Just average series" ("F button name (\"Cancel\")"), 2:"Combine rows" ("T button name (\"OK\")")) -> (T button?=w2196:bool)
        n1036 = Select(t="Combine rows" ("T button name (\"OK\")"), s=w2196, f="Average Rows together") -> (s? t:f=w2193:string)
      }
      frame "Combine rows" {
        w2206 = TRUE  # Show panel ?
        n1037 = local read "Output Filename"() -> (w2205:path)
        n1038 = call "Combined_file_Panel.vi"("Show panel ?"=w2206, "Output filename"=w2205) -> ("Only Plotted data?"=w2207:bool, "Include Empty Rows? Out"=w2208:bool, "Give Audit Channels Out"=w2209:bool, "Output filename Out"=w2204:path)  [unwired: 5 out]
        n1039 = case shown="False" w2207 {
          tunnel: w2211 -> [w2220 w2223]
          tunnel: [w2220 w2221] -> w2210
          frame False {
          }
          frame True {
            n1040 = global read "Results_plotter_Global.vi" "Plot Index values"() -> (w2225:dbl[][])
            n1041 = Index Array(array=w2225, index (row)=2) -> (element=w2222:dbl[])  [unwired: 1 in]
            n1042 = for {
              tunnel: w2223 -> [w2228]
              tunnel: w2222 -> [w2227] mode=indexing
              tunnel: [w2226] -> w2221 mode=indexing
              n1043 = Index Array(array=w2228, index (row)=w2227) -> (element=w2226:string[])  [unwired: 1 in]
            }
          }
        }
        n1044 = local write "Save Averaged rows"(FALSE ("Save Plot data")) -> ()
        n1045 = local read "X Ch Name"() -> (w2215:u16)
        n1046 = local read "Y Ch Name"() -> (w2216:u16)
        n1047 = local read "Z Ch Name"() -> (w2217:u16)
        n1048 = call "Find_Rows_to_Combine.vi"("Include Empty Rows?"=w2208, "file path (dialog if empty)"=w2204, "Give Audit Channels"=w2209, "Full Channel Names"=w2214, "Data"=w2210, "Z Column Index"=w2217, "Y Column Index"=w2216, "X Column Index"=w2215) -> ()  [unwired: 4 out]
        n1049 = local write "Output Filename"(w2204) -> ()
      }
      frame "Average Rows together" {
        n1050 = global read "Results_plotter_Global.vi" "XY Graph Cluster"() -> (w2230:cluster{dbl[], dbl[]}[])
        n1051 = local read "Tolerances"() -> (w2236:dbl[])
        n1052 = local read "Absisca"() -> (w2235:u16)
        n1053 = local read "Transpose"() -> (w2234:bool)
        n1054 = global read "Results_plotter_Global.vi" "Precision"() -> (w2232:string[])
        n1055 = global read "Results_plotter_Global.vi" "Summarise"() -> (w2231:string[])
        n1056 = stacked-sequence {
          seq-local: [w2248 _ _ _ _] -> [_ w2265 _ _ _]
          seq-local: [_ w2268 _ _ _] -> [_ _ _ w2350 _]
          seq-local: [w2244 _ _ _ _] -> [_ w2266 _ _ _]
          seq-local: [_ _ w2328 _ _] -> [_ _ _ w2344 _]
          tunnel: [_ _ _ _ TRUE] -> w2242
          tunnel: [_ _ _ _ "Create Selectors"] -> w2241
          tunnel: w2239 -> [_ w2271 _ _ w2353]
          tunnel: w2240 -> [_ _ w2329 _ w2352]
          tunnel: [_ _ _ _ w2352] -> w2238
          tunnel: [_ _ _ _ w2353] -> w2237
          tunnel: w2236 -> [w2250 w2269 _ _ _]
          tunnel: w2230 -> [w2249 _ _ _ _]
          tunnel: w2235 -> [w2247 _ _ _ _]
          tunnel: w2234 -> [w2246 _ _ _ _]
          tunnel: w2233 -> [w2243 _ _ _ _]
          tunnel: w2232 -> [_ w2270 _ _ _]
          tunnel: w2231 -> [_ w2267 w2330 _ _]
          tunnel: [w2243 _ _ _ _] -> w2229
          frame #0 {
            n1057 = Not(x=w2246) -> (.not. x?=w2253:bool)
            n1058 = for {
              tunnel: w2249 -> [w2260] mode=indexing
              tunnel: w2253 -> [w2257]
              shift-right: [w2255] -> w2251
              shift-left: dbl[] [] -> [w2256]
              n1059 = Unbundle(w2260) -> (w2259:dbl[], w2258:dbl[])
              n1060 = Select(t=w2259, s=w2257, f=w2258) -> (s? t:f=w2254:dbl[])
              n1061 = Build Array (concatenate)(w2256, w2254) -> (w2255:dbl[])
            }
            n1062 = Index Array(array=w2250, index=w2247) -> (element=w2245:dbl)
            n1063 = call "Numeric_bins.vi"("Values"=w2251, "Tolerance"=w2245) -> ("Bin Centres"=w2248:dbl[], "Bin Index"=w2244:i32[])  [unwired: 1 out]
          }
          frame #1 {
            n1064 = Array Size(array=w2265) -> (size(s)=w2264:i32)
            n1065 = global read "Results_plotter_Global.vi" "Plot Index values"() -> (w2262:dbl[][])
            n1066 = Index Array(array=w2262, index (row)=2) -> (element=w2261:dbl[])  [unwired: 1 in]
            n1067 = for {
              N: w2264 -> [_]
              tunnel: w2271 -> [w2281]
              tunnel: w2270 -> [w2280]
              tunnel: w2269 -> [w2279]
              tunnel: [w2272] -> w2268 mode=indexing
              tunnel: w2267 -> [w2278]
              tunnel: w2266 -> [w2276]
              tunnel: w2261 -> [w2275]
              i -> [w2277]
              n1068 = stacked-sequence {
                seq-local: [w2285 _] -> [_ w2304]
                tunnel: w2281 -> [_ w2305]
                tunnel: w2280 -> [_ w2303]
                tunnel: w2279 -> [_ w2302]
                tunnel: w2278 -> [_ w2301]
                tunnel: w2277 -> [w2284 _]
                tunnel: w2276 -> [w2283 _]
                tunnel: w2275 -> [w2282 _]
                tunnel: [_ w2299] -> w2274
                tunnel: [_ w2298] -> w2273
                frame #0 {
                  n1069 = for {
                    shift-right: [w2291] -> w2285
                    shift-left: i32[] [] -> [w2292]
                    tunnel: w2284 -> [w2290]
                    tunnel: w2283 -> [w2289] mode=indexing
                    tunnel: w2282 -> [w2287] mode=indexing
                    n1070 = Equal?(x=w2289, y=w2290) -> (x = y?=w2288:bool)
                    n1071 = case shown="False" w2288 {
                      tunnel: w2292 -> [w2293 w2296]
                      tunnel: [w2293 w2297] -> w2291
                      tunnel: w2287 -> [_ w2294]
                      frame False {
                      }
                      frame True {
                        n1072 = To Long Integer(number=w2294) -> (32bit integer=w2295:i32)
                        n1073 = Build Array (concatenate)(w2296, w2295) -> (w2297:i32[])
                      }
                    }
                  }
                }
                frame #1 {
                  n1074 = for {
                    tunnel: w2305 -> [w2319]
                    tunnel: w2304 -> [w2318]
                    tunnel: w2303 -> [w2316] mode=indexing
                    tunnel: w2302 -> [w2315] mode=indexing
                    tunnel: [w2314] -> w2299 mode=indexing
                    tunnel: w2301 -> [w2311] mode=indexing
                    shift-right: [w2306] -> w2298
                    shift-left: string[] [] -> [w2307]
                    i -> [w2313]
                    n1075 = for {
                      tunnel: w2319 -> [w2327]
                      tunnel: w2318 -> [w2326] mode=indexing
                      tunnel: [w2325] -> w2317 mode=indexing
                      tunnel: w2313 -> [w2324]
                      n1076 = Index Array(array=w2327, index (row)=w2326, index (col)=w2324) -> (element=w2325:string)
                    }
                    n1077 = Equal?(x="TRUE", y=w2311) -> (x = y?=w2310:bool)
                    n1078 = Not(x=w2310) -> (.not. x?=w2309:bool)
                    n1079 = call "Value_Occurence_Analysis.vi"("Average Numeric Values?"=w2309, "Tolerance"=w2315, "Precision (3)"=w2316, "String Array"=w2317) -> ("St Dev"=w2308:string, "Output String"=w2314:string)  [unwired: 1 out]
                    n1080 = case shown="False" w2309 {
                      tunnel: w2308 -> [_ w2323]
                      tunnel: w2307 -> [w2320 w2322]
                      tunnel: [w2320 w2321] -> w2306
                      frame False {
                      }
                      frame True {
                        n1081 = Build Array (concatenate)(w2322, w2323) -> (w2321:string[])
                      }
                    }
                  }
                }
              }
              n1082 = Build Array (concatenate)(w2274, w2273) -> (w2272:string[])
            }
          }
          frame #2 {
            n1083 = for {
              tunnel: w2330 -> [w2335] mode=indexing
              shift-right: [w2331] -> w2328
              shift-left: w2329 -> [w2332]
              tunnel: w2329 -> [w2333] mode=indexing
              n1084 = Equal?(x="TRUE", y=w2335) -> (x = y?=w2334:bool)
              n1085 = case shown="False" w2334 {
                tunnel: w2333 -> [w2341 _]
                tunnel: w2332 -> [w2338 w2342]
                tunnel: [w2337 w2342] -> w2331
                frame False {
                  n1086 = Concatenate Strings(w2341, "St Dev") -> (w2339:string)
                  n1087 = Build Array (concatenate)(w2338, w2339) -> (w2337:string[])
                }
                frame True {
                }
              }
            }
          }
          frame #3 {
            w2347 = FALSE  # Save Plotted rows only?
            w2349 = TRUE  # Simple Save?
            n1088 = local read "Output Filename"() -> (w2345:path)
            n1089 = local read "Header"() -> (w2346:string)
            n1090 = local read "Template"() -> (w2348:path)
            n1091 = call "Write_output_file.vi"("Output filename"=w2345, "Header"=w2346, "Template Filename"=w2348, "Channel Names"=w2344, "Data"=w2350, "Simple Save?"=w2349, "Save Plotted rows only?"=w2347, "Summarise mode"=T9."No data summary") -> ("Output filename Out"=w2351:path)  [unwired: 4 in, 3 out]
            n1092 = local write "Output Filename"(w2351) -> ()
          }
          frame #4 {
            n1093 = local write "Save Averaged rows"(FALSE ("Save Plot data")) -> ()
          }
        }
      }
      frame "Save Surface Fit data" {
        n1094 = local read "Transpose"() -> (w2357:bool)
        n1095 = local read "Tolerances"() -> (w2364:dbl[])
        n1096 = local read "Absisca"() -> (w2363:u16)
        n1097 = global read "Results_plotter_Global.vi" "Precision"() -> (w2360:string[])
        n1098 = stacked-sequence {
          seq-local: [w2371 _ _ _ _ _] -> [_ w2390 _ _ _ _]
          seq-local: [_ w2387 _ _ _ _] -> [_ _ _ _ w2474 _]
          seq-local: [_ _ w2413 _ _ _] -> [_ _ _ _ w2493 _]
          seq-local: [w2372 _ _ _ _ _] -> [_ _ w2414 _ _ _]
          seq-local: [_ _ w2409 _ _ _] -> [_ _ _ _ w2477 _]
          seq-local: [_ _ w2408 _ _ _] -> [_ _ _ w2444 _ _]
          seq-local: [_ _ _ w2439 _ _] -> [_ _ _ _ w2475 _]
          tunnel: [_ _ _ _ _ TRUE] -> w2368
          tunnel: [_ _ _ _ _ "Create Selectors"] -> w2367
          tunnel: w2365 -> [_ _ _ _ _ w2499]
          tunnel: w2366 -> [_ w2375 _ _ _ w2500]
          tunnel: w2364 -> [_ w2401 _ _ _ _]
          tunnel: w2363 -> [_ w2402 _ _ _ _]
          tunnel: [_ _ w2419 _ _ _] -> w2362
          tunnel: w2361 -> [_ w2378 w2419 _ _ _]
          tunnel: w2360 -> [_ _ w2415 _ _ _]
          tunnel: [_ _ _ _ _ w2500] -> w2359
          tunnel: [_ _ _ _ _ w2499] -> w2358
          tunnel: w2357 -> [_ _ _ w2438 _ _]
          frame #0 {
            n1099 = global read "Results_plotter_Global.vi" "X Values"() -> (w2371:dbl[])
            n1100 = global read "Results_plotter_Global.vi" "Raw Interpolation"() -> (w2369:dbl[][])
            n1101 = global read "Results_plotter_Global.vi" "Y Values"() -> (w2370:dbl[])
            n1102 = Insert Into Array(array=w2369, index (col)=0 ("disabled index (col)"), new element=w2370) -> (w2372:dbl[][])  [unwired: 1 in]
          }
          frame #1 {
            n1103 = global read "Results_plotter_Global.vi" "Y Axis Name"() -> (w2377:string)
            n1104 = Search 1D Array(1D array=w2378, element=w2377) -> (index of element=w2376:i32)  [unwired: 1 out]
            n1105 = Index Array(array=w2375, index=w2376) -> (element=w2374:string)
            n1106 = Match Pattern(string=w2374, regular expression=":") -> (before substring=w2404:string, after substring=w2403:string)  [unwired: 3 out]
            n1107 = Index Array(array=w2401, index=w2402) -> (element=w2392:dbl)
            n1108 = Concatenate Strings(w2404, " ", w2403, " =:" ("regular expression")) -> (w2386:string)
            n1109 = Greater?(x=w2392, y=0.9) -> (0:w2399:bool)
            n1110 = Greater?(x=w2392, y=0.09) -> (0:w2394:bool)
            n1111 = call <vilib>:"Trim Whitespace.vi"("string"=w2386) -> ("trimmed string"=w2385:string)  [unwired: 1 in]
            n1112 = Select(t=i16 0 ("precision (6)"), s=w2399, f=i16 2 ("precision (6)")) -> (s? t:f=w2395:i16)
            n1113 = Select(t=w2395, s=w2394, f=i16 3) -> (s? t:f=w2391:i16)
            n1114 = Number To Fractional String(number=w2390, precision (6)=w2391) -> (F-format string=w2389:string[])  [unwired: 2 out]
            n1115 = for {
              tunnel: w2385 -> [w2407]
              tunnel: w2389 -> [w2405] mode=indexing
              tunnel: [w2406] -> w2380 mode=indexing
              n1116 = Concatenate Strings(w2407, w2405) -> (w2406:string)
            }
            n1117 = Build Array (concatenate)("Channel:Values:Plotted" ("Input Element"), "Axis:Name:" ("Input Element"), "Axis:Values:" ("Input Element"), w2380) -> (w2387:string[])
          }
          frame #2 {
            n1118 = global read "Results_plotter_Global.vi" "X Axis Name"() -> (w2412:string)
            n1119 = Concatenate Strings(w2412, " =" ("string")) -> (w2410:string)
            n1120 = local read "Multi Ordinate"() -> (w2418:i32[])
            n1121 = Index Array(array=w2418, index=0 ("Index")) -> (element=w2416:i32)
            n1122 = Index Array(array=w2415, index=w2416) -> (element=w2408:string)
            n1123 = Index Array(array=w2419, index=w2416) -> (element=w2409:string)
            n1124 = for {
              tunnel: w2409 -> [w2421]
              tunnel: [w2424] -> w2413 mode=indexing
              tunnel: w2408 -> [w2423]
              tunnel: w2414 -> [w2422] mode=indexing
              tunnel: w2410 -> [w2420]
              n1125 = for {
                tunnel: w2422 -> [w2427] mode=indexing
                tunnel: [w2426] -> w2425 mode=indexing
                tunnel: w2423 -> [w2429]
                n1126 = Not A Number/Path/Refnum?(number/path/refnum=w2427) -> (NaN/Path/Refnum?=w2428:bool)
                n1127 = case shown="False" w2428 {
                  tunnel: w2429 -> [w2432 _]
                  tunnel: w2427 -> [w2431 _]
                  tunnel: [w2430 ""] -> w2426
                  frame False {
                    n1128 = call "Number_2_string.vi"("precision"=w2432, "number"=w2431) -> ("String"=w2430:string)
                  }
                  frame True {
                  }
                }
              }
              n1129 = Build Array (concatenate)(w2421, w2420, w2425) -> (w2424:string[])
            }
          }
          frame #3 {
            w2443 = "\t"
            n1130 = global read "Results_plotter_Global.vi" "Intensity Plot data in rows"() -> (w2445:dbl[][])
            n1131 = global read "Results_plotter_Global.vi" "Value plotted Name"() -> (w2442:string)
            n1132 = global read "Results_plotter_Global.vi" "X Axis Name"() -> (w2436:string)
            n1133 = global read "Results_plotter_Global.vi" "Y Axis Name"() -> (w2435:string)
            n1134 = case shown="False" w2438 {
              tunnel: [w2446 w2449] -> w2437
              tunnel: w2436 -> [w2447 w2449]
              tunnel: w2435 -> [w2446 w2448]
              tunnel: [w2447 w2448] -> w2434
              frame False {
              }
              frame True {
              }
            }
            n1135 = Concatenate Strings(w2437, w2443, w2434, w2443, w2442, "\r\n") -> (w2440:string)
            n1136 = for {
              tunnel: w2445 -> [w2455] mode=indexing
              tunnel: w2444 -> [w2460]
              shift-right: [w2454] -> w2439
              shift-left: w2440 -> [w2459]
              n1137 = Index Array(array=w2455, index=0) -> (element=w2451:dbl)
              n1138 = Index Array(array=w2455, index=1) -> (element=w2450:dbl)
              n1139 = Index Array(array=w2455, index=2) -> (element=w2453:dbl)
              n1140 = Not A Number/Path/Refnum?(number/path/refnum=w2453) -> (NaN/Path/Refnum?=w2452:bool)
              n1141 = case shown="False" w2452 {
                tunnel: w2460 -> [w2471 _]
                tunnel: w2459 -> [w2470 w2472]
                tunnel: w2453 -> [w2469 _]
                tunnel: [w2468 w2472] -> w2454
                tunnel: w2451 -> [w2467 _]
                tunnel: w2450 -> [w2466 _]
                frame False {
                  w2462 = "\t"
                  n1142 = call "Number_2_string.vi"("number"=w2467) -> ("String"=w2465:string)  [unwired: 1 in]
                  n1143 = call "Number_2_string.vi"("number"=w2466) -> ("String"=w2464:string)  [unwired: 1 in]
                  n1144 = call "Number_2_string.vi"("precision"=w2471, "number"=w2469) -> ("String"=w2463:string)
                  n1145 = Concatenate Strings(w2470, w2465, w2462, w2464, w2462, w2463, "\r\n") -> (w2468:string)
                }
                frame True {
                }
              }
            }
          }
          frame #4 {
            w2489 = TRUE  # append to file? (new file:F)
            n1146 = global read "Results_plotter_Global.vi" "Surface Integral"() -> (w2488:dbl)
            n1147 = global read "Results_plotter_Global.vi" "Surface Area"() -> (w2487:dbl)
            n1148 = Initialize Array("", 10 ("Dimension Size")) -> (w2498:string[])
            n1149 = Divide(x=w2488, y=w2487) -> (x/y=w2486:dbl)
            n1150 = call "Asterisk_header.vi"("Channel names"=w2498) -> ("Header string"=w2476:string)
            n1151 = call "Value_to_string.vi"("Value"=w2488, "Label for value"="Surface Integral") -> ("Output string"=w2483:string)  [unwired: 1 in]
            n1152 = call "Value_to_string.vi"("Value"=w2487, "Label for value"="Surface Area") -> ("Output string"=w2484:string)  [unwired: 1 in]
            n1153 = call "Value_to_string.vi"("Value"=w2486, "Label for value"="Surface Average") -> ("Output string"=w2482:string)  [unwired: 1 in]
            n1154 = Concatenate Strings(w2484, w2483, w2482) -> (w2479:string)
            n1155 = call "Ch_names_to_rows.vi"("Channel Names"=w2474) -> ("3 Row names"=w2473:string[][])
            n1156 = local read "Output Filename"() -> (w2490:path)
            n1157 = Build Array (concatenate)(w2473, w2493) -> (w2491:string[][])
            n1158 = Array To Spreadsheet String(array=w2491, 3:"%s" ("format string")) -> (spreadsheet string=w2478:string)  [unwired: 1 out]
            n1159 = Format Into String(format string="\n%s\n\n%s\n%s\n\n\nInterpolated Surface of %s\n%s\n%s\n%s\n\n\n%s", w2476, w2475, w2476, w2477, w2476, w2478, w2476, w2479) -> (resulting string=w2481:string)  [unwired: 2 in, 1 out]
            n1160 = call "Write_Characters_To_File.vi"("file path (dialog if empty)"=w2490, "character string"=w2481, "append to file? (new file:F)"=w2489) -> ()  [unwired: 2 in, 4 out]
          }
          frame #5 {
            n1161 = local write "Save Surface Fit"(FALSE ("Save Plot data")) -> ()
          }
        }
      }
      frame "Save Data in Rows" {
        w2515 = TRUE  # Show panel ?
        n1162 = local read "Output Filename"() -> (w2512:path)
        n1163 = local write "Save Data in Rows"(FALSE ("Save All data")) -> ()
        n1164 = call "Output_file_Panel.vi"("Show panel ?"=w2515, "Channel Names"=w2510, "Header"="Header", "Output filename"=w2512) -> ("Save Full Res Data?"=w2507:bool, "Desired Columns"=w2516:i32[], "Header Out"=w2514:string, "Output filename Out"=w2518:path, "Channels to Tabulate in header Out"=w2504:i32[], "Save Plotted rows only?"=w2505:bool, "Summarise mode"=w2513:T9, "Grouping info"=w2506:T15[])
        "Plotted rows only?" <- w2505
        n1165 = case shown="False" w2507 {
          tunnel: w2518 -> [w2534 w2536]
          tunnel: w2516 -> [w2533 _]
          tunnel: w2514 -> [w2532 _]
          tunnel: w2505 -> [w2531 _]
          tunnel: w2513 -> [w2530 _]
          tunnel: w2511 -> [w2529 _]
          tunnel: w2510 -> [w2528 _]
          tunnel: [w2527 w2536] -> w2509
          tunnel: ["Create Selectors" "Is Filename Empty?"] -> w2508
          tunnel: w2506 -> [w2523 _]
          tunnel: w2504 -> [w2522 _]
          frame False {
            w2525 = FALSE  # Simple Save?
            n1166 = local read "Template"() -> (w2526:path)
            n1167 = call "Write_output_file.vi"("Output filename"=w2534, "Header"=w2532, "Template Filename"=w2526, "Channel Names"=w2528, "Data"=w2529, "Desired Columns"=w2533, "Simple Save?"=w2525, "Save Plotted rows only?"=w2531, "Summarise mode"=w2530, "Grouping info"=w2523, "Channels to Tabulate in header"=w2522) -> ("Output filename Out"=w2527:path)  [unwired: 1 in, 3 out]
          }
          frame True {
            "Mode" <- Plotter_Mode."Save file" ("Mode")
          }
        }
        n1168 = local write "Output Filename"(w2509) -> ()
      }
      frame "Is Filename Empty?" {
        # "This Express VI is the reason we can't strip object code from ResultsFilePlotter; may be able to convert to standard VI"
        n1169 = call "File Dialog"("start path"="Full_Res_Results_Folder", "prompt"="Please select a new or existing folder to save the results files in") -> ("selected path"=w2540:path, "cancelled"=w2538:bool)  [unwired: 5 in, 7 out]
        n1170 = local write "Full_Res_Results_Folder"(w2540) -> ()
        n1171 = case shown="False" w2538 {
          tunnel: ["Full Res file manipulator" ("f") "Create Selectors" ("t")] -> w2542
          frame False {
          }
          frame True {
          }
        }
      }
      frame "Check for overwrite or append" {
        n1172 = local read "Output Filename"() -> (w2556:path)
        n1173 = Format Into String(format string="Do you want to append to the result file\n\"%s\"" ("message"), w2556) -> (resulting string=w2551:string)  [unwired: 2 in, 1 out]
        n1174 = call <vilib>:"Three Button Dialog.vi"("Window Title (\"\")"="Output File Dialog" ("Window Title (\"\")"), "Right Button Text (\"Cancel\")"="Cancel" ("Button 3 Name"), "Center Button Text (\"No\")"="Overwrite" ("F button name (\"Cancel\")"), "Left Button Text (\"Yes\")"="Append" ("T button name (\"OK\")"), "message"=w2551) -> ("Which Button?"=w2550:T11)  [unwired: 6 out]
        n1175 = case shown="\"Center Button\"" w2550 {
          tunnel: w2556 -> [_ w2563 _]
          tunnel: ["Full Res file manipulator" "Full Res file manipulator" "Create Selectors" ("t")] -> w2549
          frame "Left Button" {
          }
          frame "Center Button" {
            n1176 = call "Delete_with_Check.vi"("FilePath"=w2563) -> ()  [unwired: 1 out]
          }
          frame "Right Button", Default {
          }
        }
      }
      frame "Create Plot summary" {
        w2578 = TRUE  # Summarise All
        n1177 = global read "Results_plotter_Global.vi" "Plot Index values"() -> (w2581:dbl[][])
        n1178 = local read "Intensity Plot?"() -> (w2577:bool)
        n1179 = global read "Results_plotter_Global.vi" "Row Reference"() -> (w2573:i32[][])
        n1180 = Index Array(array=w2573, index (col)=0 ("disabled index (col)")) -> (element=w2572:i32[])  [unwired: 1 in]
        n1181 = Index Array(array=w2581, index (row)=2) -> (element=w2583:dbl[])  [unwired: 1 in]
        n1182 = Select(t="Save Intensity plot as jpg", s=w2577, f="Create summary per series") -> (s? t:f=w2568:string)
        n1183 = To Long Integer(number=w2583) -> (32bit integer=w2580:i32[])
        n1184 = for {
          tunnel: w2588 -> [w2601]
          tunnel: [w2600] -> w2579 mode=indexing
          tunnel: w2580 -> [w2598] mode=indexing
          tunnel: w2572 -> [w2599]
          shift-right: [w2595] -> w2570
          shift-left: i32[] [] -> [w2596]
          n1185 = Index Array(array=w2599, index=w2598) -> (element=w2594:i32)
          n1186 = Search 1D Array(1D array=w2596, element=w2594) -> (index of element=w2597:i32)  [unwired: 1 out]
          n1187 = Index Array(array=w2601, index (row)=w2598) -> (element=w2600:string[])  [unwired: 1 in]
          n1188 = case shown="0, Default" w2597 {
            tunnel: w2594 -> [_ w2605]
            tunnel: w2596 -> [w2602 w2604]
            tunnel: [w2602 w2603] -> w2595
            frame 0, Default {
            }
            frame -1 {
              n1189 = Build Array (concatenate)(w2604, w2605) -> (w2603:i32[])
            }
          }
        }
        n1190 = local read "Result files to read"() -> (w2569:path[])
        n1191 = for {
          tunnel: w2570 -> [w2593] mode=indexing
          tunnel: w2569 -> [w2592]
          tunnel: [w2589] -> w2567 mode=indexing
          n1192 = Index Array(array=w2592, index=w2593) -> (element=w2591:path)
          n1193 = Strip Path(path=w2591) -> (name=w2590:string)  [unwired: 1 out]
          n1194 = call "Add_filename_suffix.vi"("Filename"=w2590) -> ("Base name"=w2589:string)  [unwired: 1 in, 3 out]
        }
        n1195 = call "Value_Occurence_Analysis.vi"("String Array"=w2567) -> ("Output String"=w2566:string)  [unwired: 3 in, 2 out]
        n1196 = global write "Results_plotter_Global.vi" "Current Data Filenames"(w2566) -> ()
        n1197 = call "Summarise.vi"("Channel Names"=w2584, "Data"=w2579, "Summarise All"=w2578) -> ("Summary"=w2586:string[][])  [unwired: 2 in]
        n1198 = global write "Results_plotter_Global.vi" "Plot Summary"(w2586) -> ()
      }
      frame "Create summary per series" {
        n1199 = global read "Results_plotter_Global.vi" "Plot Summary"() -> (w2607:string[][])
        n1200 = local read "Plotted Series"() -> (w2609:bool[][])
        n1201 = for {
          tunnel: w2609 -> [w2626] mode=indexing
          tunnel: i32[] [] -> [w2625]
          tunnel: w2614 -> [w2623]
          tunnel: w2611 -> [w2621]
          shift-right: [w2615] -> w2606
          shift-left: w2607 -> [w2617]
          w2620 = TRUE  # Summarise All
          n1202 = for {
            shift-right: [w2634] -> w2624
            shift-left: w2625 -> [w2635]
            tunnel: w2626 -> [w2633] mode=indexing
            i -> [w2636]
            n1203 = case shown="True" w2633 {
              tunnel: w2636 -> [_ w2640]
              tunnel: w2635 -> [w2637 w2639]
              tunnel: [w2637 w2638] -> w2634
              frame False {
              }
              frame True {
                n1204 = Build Array (concatenate)(w2639, w2640) -> (w2638:i32[])
              }
            }
          }
          n1205 = for {
            tunnel: w2624 -> [w2632] mode=indexing
            tunnel: w2623 -> [w2631]
            tunnel: [w2630] -> w2622 mode=indexing
            n1206 = Index Array(array=w2631, index (row)=w2632) -> (element=w2630:string[])  [unwired: 1 in]
          }
          n1207 = call "Summarise.vi"("Channel Names"=w2621, "Data"=w2622, "Summarise All"=w2620) -> ("Summary"=w2618:string[][])  [unwired: 2 in]
          n1208 = Index Array(array=w2618, index (col)=2 ("disabled index (col)")) -> (element=w2616:string[])  [unwired: 1 in]
          n1209 = for {
            tunnel: w2617 -> [w2629] mode=indexing
            tunnel: w2616 -> [w2628] mode=indexing
            tunnel: [w2627] -> w2615 mode=indexing
            n1210 = Build Array (concatenate)(w2629, w2628) -> (w2627:string[])
          }
        }
        n1211 = global write "Results_plotter_Global.vi" "Plot Summary"(w2606) -> ()
      }
      frame "Save Intensity plot as jpg" {
        n1212 = local read "Job Directory"() -> (w2647:path)
        n1213 = global read "Constants_global.vi" "EnFlo SW Folder"() -> (w2649:path)
        n1214 = Build Path(base path=w2649, name or relative path=path "Anemometry/Anemometry Sub Vis/Data_plotting_vis/Intensity Plot Vis") -> (appended path=w2643:path)
        n1215 = call "Remote_call_prep.vi"("Vi Name in"="Create picture Vi Name", "Job Directory In"=w2647, "VI Directory"=w2643) -> ("Vi Name out"=w2645:string, "Job Directory out"=w2642:path, "cancelled"=w2641:bool)
        n1216 = local write "Create picture Vi Name"(w2645) -> ()
        n1217 = local write "Job Directory"(w2642) -> ()
        n1218 = Build Path(base path=w2643, name or relative path=w2645) -> (appended path=w2644:path)
        n1219 = case shown="False" w2641 {
          tunnel: w2644 -> [w2658 _]
          tunnel: w2642 -> [w2657 _]
          frame False {
            n1220 = Open VI Reference(type specifier VI Refnum (for type only)="type specifier VI Refnum (for type only)", vi path=w2658) -> (vi reference=w2663:refnum<vi>, error out=w2662:errorcluster)  [unwired: 2 in, 2 out]
            n1221 = property class="VI Interface Type 0"(reference=w2663, error in=w2662, "Front Panel Window:Open"=TRUE) -> (reference out=w2659:refnum<vi>, error out=w2660:errorcluster)
            n1222 = local read "Intensity Graph"() -> (w2666:dbl[][])
            n1223 = local read "No of Contours"() -> (w2656:i32)
            n1224 = call-by-ref "?"(reference=w2659, error in=w2660, "No of Contours"=w2656, "Job Directory"=w2657, "Intensity Graph"=w2666) -> (reference out=w2665:refnum<vi>, error out=w2664:errorcluster)  [unwired: 3 in]
            n1225 = Close Reference(reference=w2665, error in (no error)=w2664) -> ()  [unwired: 1 out]
          }
          frame True {
          }
        }
        n1226 = local write "Save Plot as jpg"(FALSE ("Save All data")) -> ()
      }
      frame "Run Calculation Routine" {
        n1227 = stacked-sequence {
          seq-local: [w2675 _ _] -> [_ w2685 _]
          seq-local: [w2674 _ _] -> [_ w2686 _]
          tunnel: [_ w2684 _] -> w2669
          tunnel: w2668 -> [_ _ _]
          frame #0 {
            n1228 = global read "Constants_global.vi" "EnFlo SW Folder"() -> (w2681:path)
            n1229 = Build Path(base path=w2681, name or relative path=path "Anemometry/Anemometry Sub Vis/Data_plotting_vis/Calculation Vis") -> (appended path=w2678:path)
            n1230 = local read "Job Directory"() -> (w2677:path)
            n1231 = call "Remote_call_prep.vi"("Vi Name in"="...using routine", "Job Directory In"=w2677, "VI Directory"=w2678) -> ("Vi Name out"=w2679:string, "Job Directory out"=w2676:path, "cancelled"=w2675:bool)
            n1232 = local write "Job Directory"(w2676) -> ()
            n1233 = local write "...using routine"(w2679) -> ()
            n1234 = Build Path(base path=w2678, name or relative path=w2679) -> (appended path=w2674:path)
          }
          frame #1 {
            n1235 = case shown="False" w2685 {
              tunnel: w2686 -> [w2694 _]
              tunnel: [w2690 w2707] -> w2684
              tunnel: "What to do next?" -> [w2689 w2707]
              frame False {
                n1236 = Open VI Reference(type specifier VI Refnum (for type only)="VI Refnum Calculation", vi path=w2694) -> (vi reference=w2700:refnum<vi>, error out=w2699:errorcluster)  [unwired: 1 in, 3 out]
                n1237 = property class="VI Interface Type 1"(reference=w2700, error in=w2699, "Front Panel Window:Open"=TRUE) -> (reference out=w2696:refnum<vi>, error out=w2697:errorcluster)
                n1238 = call-by-ref "?"(reference=w2696, error in=w2697) -> (reference out=w2702:refnum<vi>, error out=w2701:errorcluster, "New Values In"=w2687:string[][], "New Chs In"=w2695:string[])  [unwired: 2 in]
                n1239 = for {
                  tunnel: w2695 -> [w2705] mode=indexing
                  tunnel: [w2704] -> w2688 mode=indexing
                  n1240 = call "Check_Ch_Name_colons.vi"("No of Colons"=2, "Ch Name in"=w2705) -> ("Ch Name out"=w2704:string)
                }
                n1241 = Empty String/Path?(string/path=w2688) -> (empty?=w2692:bool[])
                n1242 = Or Array Elements(Boolean array=w2692) -> (logical OR=w2691:bool)
                n1243 = Close Reference(reference=w2702, error in (no error)=w2701) -> ()  [unwired: 1 out]
                n1244 = Select(t=w2689, s=w2691, f="Input calculated values") -> (s? t:f=w2690:string)
                n1245 = global write "Results_plotter_Global.vi" "New Values In"(w2687) -> ()
                n1246 = global write "Results_plotter_Global.vi" "New Chs In"(w2688) -> ()
              }
              frame True {
              }
            }
          }
          frame #2 {
            w2710 = FALSE ("Raw DF in Orig Pos?")
            n1247 = local write "Edit Raw Data Header Info"(w2710) -> ()
            n1248 = local write "Calculate new metadata"(FALSE ("Save All data")) -> ()
            n1249 = local write "Plotted rows only?"(TRUE ("Plotted rows only?")) -> ()
            n1250 = local write "Raw DF in Orig Pos?"(w2710) -> ()
            n1251 = local write "Edit Raw DF?"(w2710) -> ()
            n1252 = local write "Mode"(Plotter_Mode."Edit values per row" ("Mode")) -> ()
          }
        }
      }
      frame "Input calculated values" {
        n1253 = local read "Result files to read"() -> (w2716:path[])
        n1254 = local read "Raw DF in Orig Pos?"() -> (w2713:bool)
        n1255 = stacked-sequence {
          seq-local: [w2720 _ _ _] -> [_ w2733 w2745 _]
          seq-local: [_ w2730 _ _] -> [_ _ w2746 _]
          tunnel: [_ _ _ w2798] -> w2718
          tunnel: w2716 -> [_ _ w2747 _]
          tunnel: w2715 -> [_ _ w2744 _]
          tunnel: w2714 -> [_ _ w2743 _]
          tunnel: w2713 -> [_ _ w2742 _]
          tunnel: w2712 -> [_ _ _ w2795]
          frame #0 {
            n1256 = global read "Results_plotter_Global.vi" "Plot Index values"() -> (w2723:dbl[][])
            n1257 = global read "Results_plotter_Global.vi" "Row Reference"() -> (w2724:i32[][])
            n1258 = Index Array(array=w2723, index (row)=2) -> (element=w2721:dbl[])  [unwired: 1 in]
            n1259 = for {
              tunnel: w2724 -> [w2728]
              tunnel: w2721 -> [w2727] mode=indexing
              tunnel: [w2726] -> w2720 mode=indexing
              n1260 = Index Array(array=w2728, index (row)=w2727) -> (element=w2726:i32[])  [unwired: 1 in]
            }
            n1261 = local write "Delete Plotted data from file"(FALSE ("Save All data")) -> ()
          }
          frame #1 {
            n1262 = Index Array(array=w2733, index (col)=0 ("disabled index (col)")) -> (element=w2729:i32[])  [unwired: 1 in]
            n1263 = for {
              shift-right: [w2735] -> w2730
              shift-left: i32[] [] -> [w2736]
              tunnel: w2729 -> [w2734] mode=indexing
              n1264 = Search 1D Array(1D array=w2736, element=w2734) -> (index of element=w2737:i32)  [unwired: 1 out]
              n1265 = case shown="-1" w2737 {
                tunnel: w2736 -> [w2738 w2741]
                tunnel: [w2738 w2740] -> w2735
                tunnel: w2734 -> [_ w2739]
                frame 0, Default {
                }
                frame -1 {
                  n1266 = Build Array (concatenate)(w2741, w2739) -> (w2740:i32[])
                }
              }
            }
          }
          frame #2 {
            n1267 = for {
              tunnel: w2747 -> [w2754]
              tunnel: w2746 -> [w2751] mode=indexing
              tunnel: w2745 -> [w2752]
              tunnel: w2744 -> [w2750]
              tunnel: w2743 -> [w2749]
              tunnel: w2742 -> [w2748]
              # "New Values"
              # "Row in file"
              n1268 = Index Array(array=w2754, index=w2751) -> (element=w2753:path)
              n1269 = stacked-sequence {
                seq-local: [w2759 _] -> [_ w2793]
                seq-local: [w2757 _] -> [_ w2788]
                tunnel: w2753 -> [_ w2794]
                tunnel: w2752 -> [w2761 _]
                tunnel: w2751 -> [w2760 _]
                tunnel: w2750 -> [_ _]
                tunnel: w2749 -> [_ _]
                tunnel: w2748 -> [_ w2792]
                frame #0 {
                  n1270 = global read "Results_plotter_Global.vi" "New Values In"() -> (w2755:string[][])
                  n1271 = for {
                    tunnel: w2760 -> [w2772]
                    tunnel: w2761 -> [w2768] mode=indexing
                    shift-right: [w2766] -> w2759
                    shift-left: i32[] [] -> [w2767]
                    shift-right: [w2765] -> w2757
                    shift-left: string[][] [] -> [w2764]
                    tunnel: w2755 -> [w2763]
                    i -> [w2762]
                    n1272 = Index Array(array=w2768, index=0) -> (element=w2770:i32)
                    n1273 = Equal?(x=w2770, y=w2772) -> (x = y?=w2769:bool)
                    n1274 = case shown="True" w2769 {
                      tunnel: w2768 -> [_ w2778]
                      tunnel: w2767 -> [w2774 w2783]
                      tunnel: [w2774 w2781] -> w2766
                      tunnel: w2764 -> [w2773 w2779]
                      tunnel: [w2773 w2780] -> w2765
                      tunnel: w2763 -> [_ w2776]
                      tunnel: w2762 -> [_ w2775]
                      frame False {
                      }
                      frame True {
                        n1275 = Index Array(array=w2776, index (row)=w2775) -> (element=w2777:string[])  [unwired: 1 in]
                        n1276 = Index Array(array=w2778, index=1) -> (element=w2782:i32)
                        n1277 = Build Array (concatenate)(w2783, w2782) -> (w2781:i32[])
                        n1278 = Build Array (concatenate)(w2779, w2777) -> (w2780:string[][])
                      }
                    }
                  }
                }
                frame #1 {
                  w2787 = FALSE  # Edit all Rows?
                  w2789 = FALSE  # Edit Raw DF?
                  w2790 = FALSE  # Edit Raw Data Header Info
                  w2791 = FALSE  # Value  Constant?
                  n1279 = global read "Results_plotter_Global.vi" "New Chs In"() -> (w2785:string[])
                  n1280 = local read "Job Directory"() -> (w2786:path)
                  n1281 = call "Add_Update_Values.vi"("Filename"=w2794, "Value  Constant?"=w2791, "Edit Raw data files?"=w2789, "New Chs In"=w2785, "Edit Raw Data Header Info"=w2790, "New Values In"=w2788, "Selected Rows"=w2793, "Edit all Rows?"=w2787, "Raw DF in Orig Pos?"=w2792, "Job Directory"=w2786) -> ()  [unwired: 1 in, 5 out]
                }
              }
            }
          }
          frame #3 {
            n1282 = local read "nRows"() -> (w2797:i32)
            n1283 = Less?(x=w2797, y=w2795) -> (x < y?=w2796:bool)
            n1284 = Current VI's Path() -> (path=w2799:path)
            n1285 = case shown="True" w2796 {
              tunnel: ["Create Selectors" "Initialise" ("t")] -> w2798
              frame False {
              }
              frame True {
              }
            }
            n1286 = call "Bring_to_front.vi"("path"=w2799) -> ()
          }
        }
      }
      frame "Save XY plot as jpg" {
        n1287 = local read "Create picture Vi Name"() -> (w2806:string)
        n1288 = local read "Job Directory"() -> (w2809:path)
        n1289 = global read "Constants_global.vi" "EnFlo SW Folder"() -> (w2811:path)
        n1290 = Build Path(base path=w2811, name or relative path=path "Anemometry/Anemometry Sub Vis/Data_plotting_vis/XY Plot Vis") -> (appended path=w2807:path)
        n1291 = call "Remote_call_prep.vi"("Vi Name in"=w2806, "Job Directory In"=w2809, "VI Directory"=w2807) -> ("Vi Name out"=w2808:string, "Job Directory out"=w2804:path, "cancelled"=w2803:bool)
        n1292 = local write "Create picture Vi Name"(w2808) -> ()
        n1293 = local write "Job Directory"(w2804) -> ()
        n1294 = Build Path(base path=w2807, name or relative path=w2808) -> (appended path=w2805:path)
        n1295 = case shown="False" w2803 {
          tunnel: [w2824 FALSE ("Saved Automatically?")] -> w2814
          tunnel: [w2823 path "" ("Plot data file")] -> w2813
          tunnel: [w2822 "" ("Tex Info String")] -> w2812
          tunnel: w2805 -> [w2821 _]
          tunnel: w2804 -> [w2820 _]
          frame False {
            n1296 = Open VI Reference(type specifier VI Refnum (for type only)="type specifier VI Refnum (for type only) 2", vi path=w2821) -> (vi reference=w2831:refnum<vi>, error out=w2830:errorcluster)  [unwired: 1 in, 3 out]
            n1297 = property class="VI Interface Type 2"(reference=w2831, error in=w2830, "Front Panel Window:Open"=TRUE) -> (reference out=w2827:refnum<vi>, error out=w2828:errorcluster)
            n1298 = global read "Results_plotter_Global.vi" "XY Graph Cluster"() -> (w2825:cluster{dbl[], dbl[]}[])
            n1299 = call-by-ref "?"(reference=w2827, error in=w2828, "Plot Array"=w2825, "Template"=w2820) -> (reference out=w2833:refnum<vi>, error out=w2832:errorcluster, "Saved Automatically?"=w2824:bool, "Tex Info String"=w2822:string, "Plot data file"=w2823:path)
            n1300 = Close Reference(reference=w2833, error in (no error)=w2832) -> ()  [unwired: 1 out]
          }
          frame True {
          }
        }
        n1301 = local write "Save Plot as jpg"(FALSE ("Save All data")) -> ()
        n1302 = case shown="True" w2814 {
          tunnel: w2813 -> [_ w2845]
          tunnel: [w2837 "Save Plot Data"] -> w2802
          tunnel: w2812 -> [_ w2843]
          frame False {
            n1303 = global read "Results_plotter_Global.vi" "New Chs In"() -> (w2842:string[])
            n1304 = Array Size(array=w2842) -> (size(s)=w2841:i32)
            n1305 = Greater Than 0?(x=w2841) -> (x > 0?=w2840:bool)
            n1306 = Select(t="Input calculated values", s=w2840, f="Create Selectors") -> (s? t:f=w2837:string)
          }
          frame True {
            n1307 = local write "Output Filename"(w2845) -> ()
            n1308 = local write "Header"(w2843) -> ()
          }
        }
      }
      frame "Full Res file manipulator" {
        n1309 = local read "Result files to read"() -> (w2855:path[])
        n1310 = local read "Output Filename"() -> (w2853:path)
        n1311 = local read "Mode"() -> (w2854:T4)
        n1312 = local read "Raw DF in Orig Pos?"() -> (w2850:bool)
        n1313 = global read "Results_plotter_Global.vi" "New Values In"() -> (w2847:string[][])
        n1314 = local read "Plotted rows only?"() -> (w2846:bool)
        n1315 = global read "Results_plotter_Global.vi" "New Chs In"() -> (w2848:string[])
        n1316 = stacked-sequence {
          seq-local: [w2860 _ _ _ _] -> [_ w2888 w2923 _ _]
          seq-local: [_ w2887 _ _ _] -> [_ _ w2924 _ _]
          seq-local: [_ w2883 _ _ _] -> [_ _ w2915 _ _]
          seq-local: [_ _ w2913 _ _] -> [_ _ _ w3136 _]
          seq-local: [_ _ w2912 _ _] -> [_ _ _ w3135 _]
          seq-local: [_ _ w2907 _ _] -> [_ _ _ w3132 _]
          tunnel: [_ _ _ w3139 _] -> w2857
          tunnel: w2855 -> [_ _ w2925 _ _]
          tunnel: w2854 -> [_ w2885 w2922 w3137 _]
          tunnel: w2853 -> [_ _ w2921 _ _]
          tunnel: w2846 -> [w2859 _ w2920 _ _]
          tunnel: w2848 -> [_ _ w2919 _ _]
          tunnel: w2852 -> [_ _ w2918 w3133 _]
          tunnel: w2851 -> [_ _ w2917 w3134 _]
          tunnel: w2850 -> [_ _ w2916 _ _]
          tunnel: w2849 -> [_ _ _ w3138 _]
          tunnel: w2847 -> [_ _ w2909 _ _]
          frame #0 {
            n1317 = global read "Results_plotter_Global.vi" "Row Reference"() -> (w2861:i32[][])
            n1318 = case shown="True" w2859 {
              tunnel: w2861 -> [w2863 w2864]
              tunnel: [w2863 w2865] -> w2860
              frame False {
              }
              frame True {
                n1319 = local read "Plotted Series"() -> (w2867:bool[][])
                n1320 = for {
                  tunnel: w2867 -> [w2874]
                  shift-right: [w2868] -> w2865
                  shift-left: i32[][] [] -> [w2870]
                  tunnel: w2864 -> [w2869] mode=indexing
                  i -> [w2873]
                  n1321 = Index Array(array=w2874, index (col)=w2873) -> (element=w2872:bool[])  [unwired: 1 in]
                  n1322 = Or Array Elements(Boolean array=w2872) -> (logical OR=w2871:bool)
                  n1323 = case shown="True" w2871 {
                    tunnel: w2870 -> [w2875 w2878]
                    tunnel: w2869 -> [_ w2877]
                    tunnel: [w2875 w2876] -> w2868
                    frame False {
                    }
                    frame True {
                      n1324 = Build Array (concatenate)(w2878, w2877) -> (w2876:i32[][])
                    }
                  }
                }
              }
            }
            n1325 = local write "Delete Plotted data from file"(FALSE ("Save All data")) -> ()
          }
          frame #1 {
            n1326 = local read "Job Directory"() -> (w2884:path)
            n1327 = case shown="\"Delete unwanted rows\", Default" w2885 {
              tunnel: [FALSE w2901] -> w2886
              tunnel: [w2897 w2899] -> w2883
              tunnel: w2884 -> [w2897 w2900]
              tunnel: [w2897 w2899] -> w2882
              frame "Post Process Plotted Rows" {
              }
              frame "Delete unwanted rows", Default {
                n1328 = call "Remote_call_prep.vi"("Job Directory In"=w2900) -> ("Job Directory out"=w2899:path)  [unwired: 2 in, 2 out]
                n1329 = local write "Job Directory"(w2899) -> ()
                n1330 = Not Equal?(x=w2900, y=w2899) -> (x != y?=w2901:bool)
              }
            }
            n1331 = Index Array(array=w2888, index (col)=0 ("disabled index (col)")) -> (element=w2880:i32[])  [unwired: 1 in]
            n1332 = for {
              shift-right: [w2890] -> w2887
              shift-left: i32[] [] -> [w2891]
              tunnel: w2880 -> [w2889] mode=indexing
              n1333 = Search 1D Array(1D array=w2891, element=w2889) -> (index of element=w2892:i32)  [unwired: 1 out]
              n1334 = case shown="-1" w2892 {
                tunnel: w2891 -> [w2893 w2896]
                tunnel: [w2893 w2895] -> w2890
                tunnel: w2889 -> [_ w2894]
                frame 0, Default {
                }
                frame -1 {
                  n1335 = Build Array (concatenate)(w2896, w2894) -> (w2895:i32[])
                }
              }
            }
            n1336 = case shown="True" w2886 {
              tunnel: w2882 -> [_ w2903]
              frame False {
              }
              frame True {
                n1337 = local read "Template"() -> (w2902:path)
                n1338 = Path To String(path=w2903) -> (string=w2906:string)
                n1339 = call "Read_Write_Template.vi"("Template File"=w2902, "Mode"=Global_mode."Write Global to File", "Single Value In"=w2906, "Data type"="Log Folder Name" ("Variable name")) -> ()  [unwired: 4 in, 8 out]
              }
            }
          }
          frame #2 {
            w2911 = path[] []
            n1340 = local read "Full_Res_Results_Folder"() -> (w2910:path)
            n1341 = for {
              tunnel: w2925 -> [w2947]
              tunnel: w2924 -> [w2944] mode=indexing
              tunnel: w2923 -> [w2945]
              tunnel: w2922 -> [w2943]
              tunnel: w2921 -> [w2942]
              tunnel: w2920 -> [w2941]
              tunnel: w2919 -> [w2940]
              tunnel: w2918 -> [w2939]
              tunnel: w2917 -> [w2938]
              tunnel: w2916 -> [w2937]
              tunnel: w2915 -> [w2936]
              shift-right: [w2935] -> _
              shift-left: FALSE -> [w2934]
              shift-right: [w2932] -> w2913
              shift-left: w2911 -> [w2933]
              shift-right: [w2930] -> w2912
              shift-left: w2911 -> [w2931]
              tunnel: w2910 -> [w2929]
              tunnel: w2909 -> [w2928]
              shift-right: [w2926] -> w2907
              shift-left: i32[] [] -> [w2927]
              # "Row No in file"
              # "Row No in plotter"
              n1342 = Index Array(array=w2947, index=w2944) -> (element=w2946:path)
              n1343 = stacked-sequence {
                seq-local: [w2952 _ _ _] -> [_ w2988 w3037 _]
                seq-local: [_ w2986 _ _] -> [_ _ w3036 _]
                seq-local: [w2948 _ _ _] -> [_ _ w3029 w3130]
                tunnel: w2946 -> [_ w2987 w3038 _]
                tunnel: w2945 -> [w2962 _ _ _]
                tunnel: w2944 -> [w2955 _ _ _]
                tunnel: w2943 -> [_ w2985 w3035 _]
                tunnel: w2942 -> [_ _ w3034 _]
                tunnel: w2941 -> [_ _ w3033 _]
                tunnel: w2940 -> [_ _ w3032 _]
                tunnel: w2939 -> [_ _ w3031 _]
                tunnel: w2938 -> [_ _ w3030 _]
                tunnel: w2937 -> [_ _ w3028 _]
                tunnel: w2936 -> [_ _ w3027 _]
                tunnel: [_ w2984 _ _] -> w2935
                tunnel: w2934 -> [_ w2983 _ _]
                tunnel: w2933 -> [_ _ w3026 _]
                tunnel: [_ _ w3025 _] -> w2932
                tunnel: w2931 -> [_ _ w3024 _]
                tunnel: [_ _ w3023 _] -> w2930
                tunnel: w2929 -> [_ _ w3022 _]
                tunnel: w2928 -> [_ _ w3021 _]
                tunnel: w2927 -> [_ _ _ w3131]
                tunnel: [_ _ _ w3129] -> w2926
                frame #0 {
                  w2961 = i32[] []
                  # "10/30/13\n#optimation"
                  n1344 = global read "Results_plotter_Global.vi" "Row Reference"() -> (w2960:i32[][])
                  n1345 = local read "Cursor index"() -> (w2959:i32)
                  n1346 = for {
                    tunnel: w2955 -> [w2971]
                    tunnel: w2962 -> [w2967] mode=indexing
                    shift-right: [w2965] -> w2953
                    shift-left: w2961 -> [w2966]
                    shift-right: [w2964] -> w2949
                    shift-left: w2961 -> [w2963]
                    n1347 = Index Array(array=w2967, index=0) -> (element=w2969:i32)
                    n1348 = Equal?(x=w2969, y=w2971) -> (x = y?=w2968:bool)
                    n1349 = case shown="True" w2968 {
                      tunnel: w2967 -> [_ w2975]
                      tunnel: w2966 -> [w2973 w2981]
                      tunnel: [w2973 w2979] -> w2965
                      tunnel: w2963 -> [w2972 w2977]
                      tunnel: [w2972 w2978] -> w2964
                      frame False {
                      }
                      frame True {
                        n1350 = Index Array(array=w2975, index=2) -> (element=w2974:i32)
                        n1351 = Build Array (concatenate)(w2977, w2974) -> (w2978:i32[])
                        n1352 = Index Array(array=w2975, index=1) -> (element=w2980:i32)
                        n1353 = Build Array (concatenate)(w2981, w2980) -> (w2979:i32[])
                      }
                    }
                  }
                  n1354 = Index Array(array=w2960, index (row)=w2959) -> (element=w2957:i32[])  [unwired: 1 in]
                  n1355 = local read "Selected Row?"() -> (w2950:bool)
                  n1356 = Index Array(array=w2957, index #1=0 ("index"), index #2=1 ("index")) -> (element #2=w2954:i32)  [unwired: 1 out]
                  n1357 = Build Array(w2954) -> (w2951:i32[])
                  n1358 = Select(t=w2951, s=w2950, f=w2949) -> (s? t:f=w2948:i32[])
                  n1359 = Select(t=w2951, s=w2950, f=w2953) -> (s? t:f=w2952:i32[])
                }
                frame #1 {
                  n1360 = case shown="\"Edit values per row\"" w2985 {
                    tunnel: w2988 -> [_ _ _ _ _ w3004]
                    tunnel: w2987 -> [_ _ _ _ _ w3002]
                    tunnel: [TRUE ("T button?") TRUE ("T button?") TRUE ("T button?") TRUE ("T button?") TRUE ("T button?") w3001] -> w2986
                    tunnel: [w2989 w2991 w2993 w2995 w2997 w3000] -> w2984
                    tunnel: w2983 -> [w2989 w2991 w2993 w2995 w2997 w2999]
                    frame "Save file" {
                    }
                    frame "Edit values per row" {
                    }
                    frame "Edit Values with constants" {
                    }
                    frame "Edit Raw Data file header" {
                    }
                    frame "Post Process Plotted Rows" {
                    }
                    frame "Delete unwanted rows" {
                      n1361 = Array Size(array=w3004) -> (size(s)=w3003:i32)
                      n1362 = case shown="False" w2999 {
                        tunnel: w3003 -> [w3013 _]
                        tunnel: w3002 -> [w3012 _]
                        tunnel: [w3007 w3020] -> w3001
                        tunnel: [w3006 w3020] -> w3000
                        frame False {
                          n1363 = Format Into String(format string="Remove %d rows from \"%s\"", w3013, w3012) -> (resulting string=w3010:string)  [unwired: 2 in, 1 out]
                          n1364 = call <vilib>:"Three Button Dialog.vi"("Allow user to close window? (TRUE)"=TRUE, "Right Button Text (\"Cancel\")"="Yes To All Files" ("Right Button Text (\"Cancel\")"), "message"=w3010) -> ("Which Button?"=w3008:T11)  [unwired: 3 in, 5 out]
                          n1365 = case shown="\"Left Button\"" w3008 {
                            tunnel: [TRUE TRUE w3018 w3019] -> w3007
                            tunnel: [FALSE TRUE w3018 w3019] -> w3006
                            frame "Left Button" {
                            }
                            frame "Right Button" {
                            }
                            frame "Center Button" {
                              w3018 = FALSE
                            }
                            frame "Window Close" {
                              w3019 = FALSE
                            }
                          }
                        }
                        frame True {
                          w3020 = TRUE
                        }
                      }
                    }
                  }
                }
                frame #2 {
                  n1366 = case shown="True" w3036 {
                    tunnel: w3038 -> [_ w3057]
                    tunnel: w3037 -> [_ w3056]
                    tunnel: w3035 -> [_ w3055]
                    tunnel: w3034 -> [_ w3054]
                    tunnel: w3033 -> [_ w3053]
                    tunnel: w3032 -> [_ w3052]
                    tunnel: w3031 -> [_ w3051]
                    tunnel: w3030 -> [_ w3050]
                    tunnel: w3029 -> [_ w3049]
                    tunnel: w3028 -> [_ w3048]
                    tunnel: w3027 -> [_ w3047]
                    tunnel: w3026 -> [w3040 w3046]
                    tunnel: [w3040 w3045] -> w3025
                    tunnel: w3024 -> [w3039 w3044]
                    tunnel: [w3039 w3043] -> w3023
                    tunnel: w3022 -> [_ w3042]
                    tunnel: w3021 -> [_ w3041]
                    frame False {
                    }
                    frame True {
                      n1367 = case shown="\"Edit Values with constants\"" w3055 {
                        tunnel: w3057 -> [w3063 w3069 w3087 w3100 w3117]
                        tunnel: w3056 -> [w3066 w3076 w3086 w3099 w3116]
                        tunnel: w3054 -> [_ _ _ _ _]
                        tunnel: w3053 -> [_ _ _ w3097 w3114]
                        tunnel: w3052 -> [_ _ _ w3095 w3112]
                        tunnel: w3051 -> [_ _ _ _ w3111]
                        tunnel: w3050 -> [_ _ _ _ w3109]
                        tunnel: w3049 -> [_ _ _ _ w3108]
                        tunnel: w3048 -> [_ _ _ w3094 w3106]
                        tunnel: w3047 -> [_ _ _ w3092 w3104]
                        tunnel: w3046 -> [w3065 w3073 w3085 w3090 w3102]
                        tunnel: [w3065 w3074 w3085 w3090 w3102] -> w3045
                        tunnel: w3044 -> [w3064 w3072 w3084 w3089 w3101]
                        tunnel: [w3064 w3070 w3084 w3089 w3101] -> w3043
                        tunnel: w3042 -> [w3062 _ _ _ _]
                        tunnel: w3041 -> [_ _ _ w3088 _]
                        frame "Save file" {
                          n1368 = Strip Path(path=w3063) -> (name=w3060:string)  [unwired: 1 out]
                          n1369 = call "Add_filename_suffix.vi"("Filename"=w3060, "Suffix to add"=".xls") -> ("Filename out"=w3058:string)  [unwired: 3 out]
                          n1370 = Build Path(base path=w3062, name or relative path=w3058) -> (appended path=w3061:path)
                          n1371 = call "Save_full_Res_rows.vi"("Selected Rows"=w3066, "Filename to write"=w3061, "Filename Orig"=w3063) -> ()  [unwired: 2 out]
                        }
                        frame "Edit Raw Data file header", Default {
                          n1372 = call "GetRawDataFilePaths.vi"("Results file or Folder"=w3069) -> ("RawDataFilePaths"=w3067:string[], "RowNumbers"=w3068:i32[])  [unwired: 9 in]
                          n1373 = for {
                            tunnel: w3067 -> [w3083]
                            tunnel: w3076 -> [w3077] mode=indexing
                            tunnel: [w3081] -> w3075 mode=indexing
                            tunnel: [w3080] -> w3071 mode=indexing
                            tunnel: w3069 -> [w3080]
                            tunnel: w3068 -> [w3079]
                            n1374 = Search 1D Array(1D array=w3079, element=w3077) -> (index of element=w3078:i32)  [unwired: 1 in]
                            n1375 = Index Array(array=w3083, index=w3078) -> (element=w3082:string)
                            n1376 = call "String_to_Pathname.vi"("Input String"=w3082) -> ("path"=w3081:path)
                          }
                          n1377 = Build Array (concatenate)(w3072, w3071) -> (w3070:path[])
                          n1378 = Build Array (concatenate)(w3073, w3075) -> (w3074:path[])
                        }
                        frame "Delete unwanted rows" {
                          n1379 = call "Delete_unwanted_rows.vi"("Selected Rows"=w3086, "Filename"=w3087) -> ()  [unwired: 1 out]
                        }
                        frame "Edit Values with constants" {
                          w3098 = TRUE  # Value  Constant?
                          n1380 = local read "Edit Raw Data Header Info"() -> (w3091:bool)
                          n1381 = local read "Edit Raw DF?"() -> (w3093:bool)
                          n1382 = Not(x=w3097) -> (.not. x?=w3096:bool)
                          n1383 = call "Add_Update_Values.vi"("Filename"=w3100, "Value  Constant?"=w3098, "Edit Raw data files?"=w3093, "New Chs In"=w3095, "Edit Raw Data Header Info"=w3091, "New Values In"=w3088, "Selected Rows"=w3099, "Edit all Rows?"=w3096, "Raw DF in Orig Pos?"=w3094, "Job Directory"=w3092) -> ()  [unwired: 1 in, 5 out]
                        }
                        frame "Edit values per row" {
                          w3103 = FALSE  # Edit Raw Data Header Info
                          w3115 = FALSE  # Value  Constant?
                          n1384 = for {
                            tunnel: w3112 -> [w3128] mode=indexing
                            tunnel: w3111 -> [w3127]
                            tunnel: [w3126] -> w3110 mode=indexing
                            n1385 = Search 1D Array(1D array=w3127, element=w3128) -> (index of element=w3126:i32)  [unwired: 1 out]
                          }
                          n1386 = for {
                            tunnel: w3110 -> [w3122]
                            tunnel: w3109 -> [w3121]
                            tunnel: w3108 -> [w3119] mode=indexing
                            tunnel: [w3118] -> w3107 mode=indexing
                            n1387 = Index Array(array=w3121, index (row)=w3119) -> (element=w3120:string[])  [unwired: 1 in]
                            n1388 = for {
                              tunnel: w3122 -> [w3125] mode=indexing
                              tunnel: w3120 -> [w3124]
                              tunnel: [w3123] -> w3118 mode=indexing
                              n1389 = Index Array(array=w3124, index=w3125) -> (element=w3123:string)
                            }
                          }
                          n1390 = Not(x=w3114) -> (.not. x?=w3113:bool)
                          n1391 = local read "Edit Raw DF?"() -> (w3105:bool)
                          n1392 = call "Add_Update_Values.vi"("Filename"=w3117, "Value  Constant?"=w3115, "Edit Raw data files?"=w3105, "New Chs In"=w3112, "Edit Raw Data Header Info"=w3103, "New Values In"=w3107, "Selected Rows"=w3116, "Edit all Rows?"=w3113, "Raw DF in Orig Pos?"=w3106, "Job Directory"=w3104) -> ()  [unwired: 1 in, 5 out]
                        }
                      }
                    }
                  }
                }
                frame #3 {
                  n1393 = Build Array (concatenate)(w3131, w3130) -> (w3129:i32[])
                }
              }
            }
          }
          frame #3 {
            n1394 = case shown="\"Edit Raw Data file header\"" w3137 {
              tunnel: ["Create Selectors" w3147 "Initialise" ("t") w3206] -> w3139
              tunnel: w3138 -> [_ _ _ w3203]
              tunnel: w3136 -> [w3140 w3146 _ _]
              tunnel: w3135 -> [_ w3145 _ _]
              tunnel: w3134 -> [_ w3144 _ _]
              tunnel: w3133 -> [_ w3143 _ _]
              tunnel: w3132 -> [_ w3142 _ _]
              frame "Edit Raw Data file header" {
                n1395 = call "Edit_Raw_DF_Header.vi"("Selected files"=w3140) -> ()  [unwired: 15 out]
              }
              frame "Post Process Plotted Rows" {
                n1396 = stacked-sequence {
                  seq-local: [w3149 _ _] -> [_ w3173 _]
                  seq-local: [w3148 _ _] -> [_ _ w3198]
                  seq-local: [_ w3170 _] -> [_ _ w3197]
                  tunnel: [_ _ "Create Selectors"] -> w3147
                  tunnel: w3146 -> [_ _ w3200]
                  tunnel: w3145 -> [_ _ w3199]
                  tunnel: w3144 -> [_ w3172 _]
                  tunnel: w3143 -> [w3150 _ _]
                  tunnel: w3142 -> [_ w3169 _]
                  frame #0 {
                    n1397 = global read "Results_plotter_Global.vi" "Dispose"() -> (w3152:string[])
                    n1398 = for {
                      tunnel: w3152 -> [w3161] mode=indexing
                      shift-right: [w3157] -> w3149
                      shift-left: i32[] [] -> [w3159]
                      i -> [w3158]
                      n1399 = String Subset(string=w3161, length (rest)=1 ("length (rest)")) -> (substring=w3163:string)  [unwired: 1 out]
                      n1400 = Equal?(x="T", y=w3163) -> (x = y?=w3160:bool)
                      n1401 = case shown="False" w3160 {
                        tunnel: w3159 -> [w3167 w3168]
                        tunnel: [w3166 w3168] -> w3157
                        tunnel: w3158 -> [w3165 _]
                        frame False {
                          n1402 = Build Array (concatenate)(w3167, w3165) -> (w3166:i32[])
                        }
                        frame True {
                        }
                      }
                    }
                    n1403 = for {
                      tunnel: w3150 -> [w3156]
                      tunnel: w3149 -> [w3155] mode=indexing
                      tunnel: [w3154] -> w3148 mode=indexing
                      n1404 = Index Array(array=w3156, index=w3155) -> (element=w3154:string)
                    }
                    n1405 = local write "Post Process Plotted Data"(FALSE ("Post Process Plotted Data")) -> ()
                  }
                  frame #1 {
                    n1406 = global read "Results_plotter_Global.vi" "Precision"() -> (w3171:string[])
                    n1407 = for {
                      tunnel: w3173 -> [w3179]
                      tunnel: w3172 -> [w3175]
                      tunnel: w3171 -> [w3178]
                      tunnel: [w3177] -> w3170 mode=indexing
                      tunnel: w3169 -> [w3176] mode=indexing
                      n1408 = Index Array(array=w3175, index (row)=w3176) -> (element=w3174:string[])  [unwired: 1 in]
                      n1409 = for {
                        tunnel: w3179 -> [w3189] mode=indexing
                        tunnel: w3174 -> [w3191]
                        tunnel: w3178 -> [w3190]
                        tunnel: [w3183] -> w3177 mode=indexing
                        n1410 = Index Array(array=w3191, index=w3189) -> (element=w3182:string)
                        n1411 = Index Array(array=w3190, index=w3189) -> (element=w3181:string)
                        n1412 = Fract/Exp String To Number(string=w3182) -> (offset past number=w3187:i32, number=w3184:dbl)  [unwired: 3 out]
                        n1413 = String Length(string=w3182) -> (length=w3188:i32)
                        n1414 = Equal?(x=w3188, y=w3187) -> (x = y?=w3185:bool)
                        n1415 = Empty String/Path?(string/path=w3182) -> (empty?=w3186:bool)
                        n1416 = Compound Arithmetic op=AND(invert w3186, w3185) -> (w3180:bool)
                        n1417 = case shown="True" w3180 {
                          tunnel: w3181 -> [_ w3194]
                          tunnel: w3184 -> [_ w3195]
                          tunnel: [w3192 w3193] -> w3183
                          tunnel: w3182 -> [w3192 _]
                          frame False {
                          }
                          frame True {
                            n1418 = call "Number_2_string.vi"("precision"=w3194, "number"=w3195) -> ("String"=w3193:string)
                          }
                        }
                      }
                    }
                  }
                  frame #2 {
                    n1419 = Build Array (concatenate)(w3198, w3197) -> (w3196:string[][])
                    n1420 = call "Post_Process_Profile_Remote.vi"("Results Plotter Rows"=w3196, "Raw Data files to PP"=w3200, "Current Results filenames"=w3199) -> ()  [unwired: 1 out]
                  }
                }
              }
              frame "Delete unwanted rows" {
              }
              frame "Edit Values with constants", Default {
                n1421 = local read "nRows"() -> (w3205:i32)
                n1422 = Less?(x=w3205, y=w3203) -> (x < y?=w3204:bool)
                n1423 = case shown="True" w3204 {
                  tunnel: ["Create Selectors" "Initialise" ("t")] -> w3206
                  frame False {
                  }
                  frame True {
                  }
                }
              }
            }
          }
          frame #4 {
            n1424 = Current VI's Path() -> (path=w3209:path)
            n1425 = call "Bring_to_front.vi"("path"=w3209) -> ()
          }
        }
      }
      frame "End" {
        n1426 = local read "Template"() -> (w3211:path)
        n1427 = local read "Empty"() -> (w3212:bool)
        n1428 = call "Valid_Path.vi"("Filename"=w3211) -> ("Valid Path?"=w3210:bool)
        n1429 = case shown="True" w3212 {
          frame False {
          }
          frame True {
            n1430 = property on="Result files to read" class="Arr (strict)"("Index Values"=u32[] [0] ("Write Attribute")) -> ()  [unwired: 2 in, 2 out]
            n1431 = local write "Result files to read"(path[] [] ("Result files to read")) -> ()
            n1432 = local write "Empty"(FALSE ("Empty")) -> ()
          }
        }
        n1433 = case shown="False" w3210 {
          tunnel: w3213 -> [w3222 _]
          frame False {
            n1434 = local write "Template"(w3222) -> ()
          }
          frame True {
          }
        }
      }
      frame "Empty Results file array" {
        n1435 = local read "Template"() -> (w3224:path)
        n1436 = call "Valid_Path.vi"("Filename"=w3224) -> ("Valid Path?"=w3223:bool)
        n1437 = case shown="True" w3223 {
          tunnel: w3225 -> [w3234 _]
          frame False {
            n1438 = local write "Template"(w3234) -> ()
          }
          frame True {
          }
        }
        n1439 = property on="Result files to read" class="Arr (strict)"("Index Values"=u32[] [0] ("Write Attribute")) -> ()  [unwired: 2 in, 2 out]
        n1440 = local write "Result files to read"(path[] [] ("Result files to read")) -> ()
        n1441 = local write "Empty"(FALSE ("Empty")) -> ()
      }
      frame "Save Setup" {
        w3239 = "Current_Setup.xls" ("Setup filename")
        n1442 = local read "Create picture Vi Name"() -> (w3254:string)
        n1443 = local read "Additional X Values"() -> (w3260:dbl[])
        n1444 = local read "Additional Y Values"() -> (w3259:dbl[])
        n1445 = local read "Result files to read"() -> (w3262:path[])
        n1446 = local read "Output Filename"() -> (w3255:path)
        n1447 = local read "Multi Ordinate?"() -> (w3252:bool)
        n1448 = local read "Intensity Plot?"() -> (w3253:bool)
        n1449 = local read "Multi Ordinate"() -> (w3248:i32[])
        n1450 = local read "Filter Array"() -> (w3256:u16[])
        n1451 = local read "Transpose"() -> (w3261:bool)
        n1452 = local read "Template"() -> (w3240:path)
        n1453 = local read "Ordinate"() -> (w3258:u16)
        n1454 = local read "Filter Bins 2"() -> (w3249:i32[])
        n1455 = local read "Filter Bins 1"() -> (w3250:i32[])
        n1456 = local read "Absisca"() -> (w3257:u16)
        n1457 = call "Read_Write_Plot_Setup.vi"("Mode"=enum16{"Load", "Save"}."Load", "Setup filename"=w3239) -> ("Cluster 2"=w3263:T10)  [unwired: 1 in, 1 out]
        n1458 = Bundle By Name(cluster=w3263, "Result files to read"=w3262, "Template"=w3240, "Transpose"=w3261, "Additional X Values"=w3260, "Additional Y Values"=w3259, "Ordinate"=w3258, "Absisca"=w3257, "Filter Array"=w3256, "color and symbol"=TRUE, "Output Filename"=w3255, "Jpg Vi Name"=w3254, "Intensity Plot?"=w3253, "Multi Ordinate?"=w3252, "Filter Bins 1"=w3250, "Filter Bins 2"=w3249, "Multi Ordinate"=w3248) -> (w3251:T10)
        n1459 = local read "Save Setup"() -> (w3238:bool)
        n1460 = local read "stop"() -> (w3246:bool)
        n1461 = Not(x=w3246) -> (.not. x?=w3245:bool)
        n1462 = Path To String(path="Job Directory") -> (string=w3244:string)
        n1463 = call "Read_Write_Plot_Setup.vi"("Mode"=enum16{"Load", "Save"}."Save", "Setup filename"=w3239, "Cluster"=w3251) -> ()  [unwired: 2 out]
        n1464 = call "Read_Write_Template.vi"("Template File"=w3240, "Mode"=Global_mode."Write Global to File", "Single Value In"=w3244, "Data type"="Log Folder Name" ("Variable name")) -> ()  [unwired: 4 in, 8 out]
        n1465 = Select(t="Save to named setup file", s=w3238, f="Check modification dates?") -> (s? t:f=w3236:string)
      }
      frame "Save to named setup file" {
        w3270 = TRUE  # Save New File?
        n1466 = call "Save_current_setup.vi"("Save New File?"=w3270, "Setup File Type"=Setup_Filetype."Results File Plotter Setups") -> ()  [unwired: 4 out]
        n1467 = local write "Save Setup"(FALSE ("Save Setup")) -> ()
      }
    }
    "Current" <- w11
  }
